vi "SpectrometerSpinCoater_v10.vi"() -> ()   [LabVIEW 2020]
uses:
  <instrlib>/Classes/CCD/Abstract_CCD/Abstract_CCD.lvclass
  TypDef/DeviceQueue_Action.ctl
  TypDef/DeviceQueue_TypeDef.ctl
  TypDef/DataQueue_Action.ctl
  TypDef/DataQueue_TypeDef.ctl
  <instrlib>/Classes/CCD/Avantes/Avantes.lvclass
  <vilib>/Utility/error.llb/DialogType.ctl
  <vilib>/Analysis/NI_AALBase.lvlib
  <vilib>/Analysis/baseanly.llb/A x Vector.vi
  <instrlib>/Classes/SpinCoater/SpinCoater.lvclass
  TypDef/TabControl.ctl
  C:/Program Files/National Instruments/LabVIEW 2020/instr.lib/Classes/CCD/Abstract_CCD/Abstract_CCD.lvclass
  C:/Program Files/National Instruments/LabVIEW 2020/instr.lib/Classes/CCD/Avantes/Avantes.lvclass
panel:
  out "Nr After Spin":u16
  out "Action":string="TimeOut"
  out "Time.spin":refnum<file>
  out "Meas.spin":refnum<file>
  out "Arduino":bool
  out "NKT":bool
  out "Spectromter":bool
  in  "Abort Button":bool
  in  "Stop Button":bool=TRUE
  in  "Tab Control":T1(tab)
  in  "Shutter Toggle":bool
  in  "Spin at end":bool
  in  "Duration after":dbl[unit]
  in  "periodic time":dbl[unit]=2.0
  in  "Program Spin Coater":T2(array[cluster])=[{"Speed (rpm)"=1500.0, "Time (s)"=5.0, "Acc (rpm/s)"=0.0}]
  in  "Spectra Count":u16
  in  "Measure_MeasureSpectrum":bool
  out "Overall Time":dbl=13.0
  in  "Seconds after Spin":dbl[unit]=3.0
  in  "Seconds to Spin":dbl[unit]=5.0
  in  "Calculate Frames":bool=TRUE
  in  "Frames":i32=34211
  in  "StartMeasurement_Button":bool
  in  "Measure_Preview":bool
  out "Measure_Graph":T3(graph) caption="XY Graph"
  in  "Measure_FramesSpectrometer":dbl=200.0 caption="Frames for Spectrometer"
  in  "StartSpin_Button":bool
  in  "Record RefSpec":bool
  in  "Measure:\nRecord_Darkspec":bool
  in  "Measure_Comments":string="Just for testing" caption="Comments"
  in  "Measure_FileName":string="TestingAfter" caption="File Name"
  in  "Measure_SavePath":path=path "C:/Users/Timo/Desktop/testz" caption="Save Path"
  out "Measure_FrameRate":dbl[unit]=2631.5791015625 caption="Frame Rate"
  in  "Measure_IntegrationTime":dbl[unit]=3e-05 caption="Integration Time"
  out "SS_StepsLeft":dbl
  out "SS_TimePrediction":dbl[unit]=-6.0
  out "Horizontal Progress Bar":u8(slide) scale=0.0..100.0
  in  "SpectralStability:\nRecord_Darkspec":bool
  in  "SpectralStability_Record":bool
  in  "SpectralStability_\nMeasurementNumber":u32 caption="Measurement Number"
  in  "SpectralStability_Duration":dbl[unit] caption="Duration"
  in  "Duration/Times":bool
  in  "SpectralStability_\nPeriodicTime":dbl[unit] caption="Periodic Time"
  in  "SpectralStability_MeasureSpectrum":bool
  in  "SpectralStability_Preview":bool
  out "SpectralStability_Graph":T3(graph) caption="XY Graph"
  in  "SpectralStability_FramesSpectrometer":dbl=200.0 caption="Frames for Spectrometer"
  in  "SpectralStability_Comments":string="Just for testing" caption="Comments"
  in  "SpectralStability_FileName":string="TestingAfter" caption="File Name"
  in  "SpectralStability_SavePath":path=path "C:/Users/Timo/Desktop/Test/180824" caption="Save Path"
  out "SpectralStability_FrameRate":dbl[unit]=2631.5791015625 caption="Frame Rate"
  in  "SpectralStability_IntegrationTime":dbl[unit]=3e-05 caption="Integration Time"
  in  "Shutter Close":bool
  in  "Shutter Open":bool
  in  "SHUTTER DEBUG":bool
  in  "Shutter Position":u16=1000
  in  "Dividider Get Spectra":u32=1 min=1
  in  "Automatically \nadjust count":bool=TRUE
  in  "Reset Count\nafter Spin Coating":bool=TRUE
  in  "ESC_Speed":dbl
  in  "ESC_Milliseconds":dbl
  in  "ESC DEBUG":bool
  in  "Port Arduino":refnum<visa-resource-name>="COM4"
  out "Error Arduino":bool caption="Error"
  in  "Init_Arduino":bool caption="Init"
  out "Caption_Settings_Arduino":string="Arduino"
  out "Caption_Settings_NKT":string="NKT Laser"
  out "Error_Spectromter":bool caption="Error"
  in  "Init_Spectrometer":bool caption="Init"
  out "Caption_Settings_Spectrometer":string="Spectromter"
  # "Speed (rpm)   Time (s)        Acceleration \n                                               (rpm/s)"
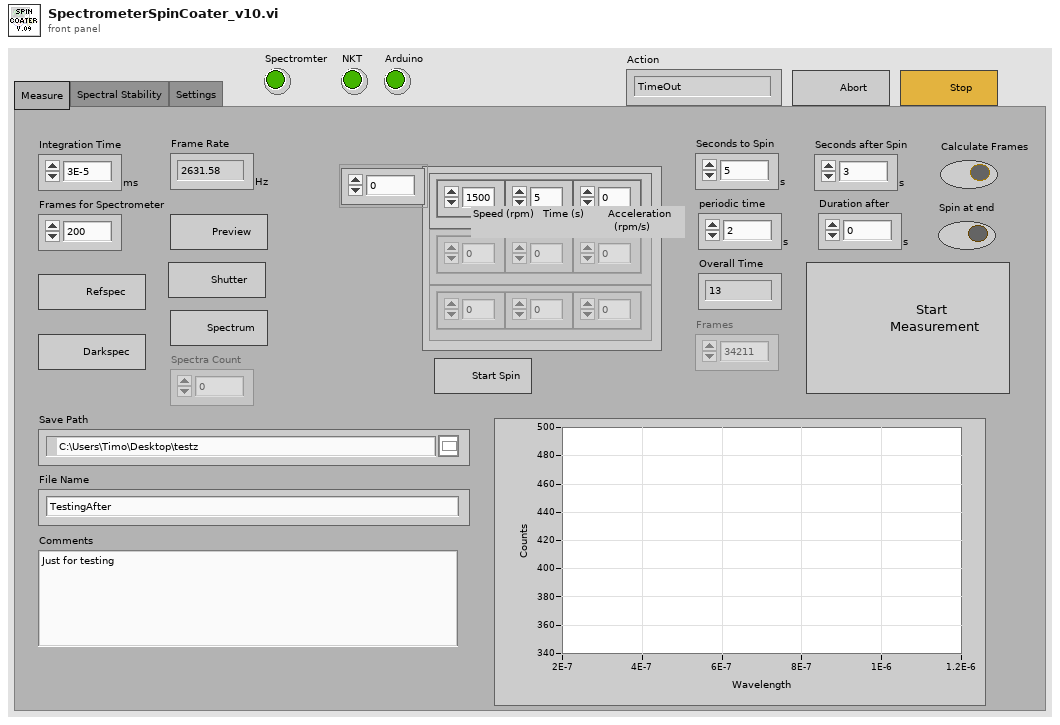
[diagram p1: front panel]
types:
  T1 = enum32{"Measure", "Spectral Stability", "Settings"}
  T2 = cluster{"Speed (rpm)":dbl, "Time (s)":dbl, "Acc (rpm/s)":dbl}[]
  T3 = cluster{"Wavlength":dbl[unit][], "Image":dbl[]}[]
  T4 = cluster{"Dark":cluster{"Image":dbl[][][], "Frame Size":cluster{"F":i32, "Y":i32, "X":i32}}[], "Ref":cluster{"Image":dbl[][][], "Frame Size":cluster{"F":i32, "Y":i32, "X":i32}}[], "Wavlength":dbl[unit][], "spec":dbl[][]}
  T5 = cluster{"Abstract_CCD.lvclass":refnum<class "Abstract_CCD.lvclass">, "SpinCoater.lvclass":refnum<class "SpinCoater.lvclass">}
  T6 = typedef "DataQueue_TypeDef.ctl" = cluster{"QueueAction":T7, "Data":cluster{"Image":dbl[][][], "Frame Size":cluster{"F":i32, "Y":i32, "X":i32}}[], "Data_Raw":cluster{"Image":dbl[][][], "Frame Size":cluster{"F":i32, "Y":i32, "X":i32}}[], "Data_Dark":cluster{"Image":dbl[][][], "Frame Size":cluster{"F":i32, "Y":i32, "X":i32}}[], "Data_Ref":cluster{"Image":dbl[][][], "Frame Size":cluster{"F":i32, "Y":i32, "X":i32}}[], "Device Information":string[], "Numeric Control":dbl, "Boolean":bool, "Wavelength":dbl[unit][], "Time":dbl[], "Time Stamp":timestamp, "Numeric Control 2":dbl, "TabControl":T8}
  T7 = typedef "DataQueue_Action.ctl" = enum16{"TimeOut", "Close_Program", "Abort", "Stop_Measurement", "Measure_InSituSpinCoating", "Measure_Spectrum", "Measure_SpectrumAdvanced", "Measure_SpectralStability", "Save_InSitu", "Save_SpectralStability", "Set_Ref", "Set_Dark", "Set_Wavelength", "Spectrometer_Measure", "Spectrometer_Preview", "Transfer_Settings"}
  T8 = typedef "TabControl.ctl" = enum16{"Measure", "Spectral Stability", "Settings"}
  T9 = typedef "DeviceQueue_TypeDef.ctl" = cluster{"QueueAction":T10, "Numeric 1":dbl, "Numeric 2":dbl, "Boolean 1":bool, "Boolean 2":bool, "Spin Program":dbl[][], "Spin Prg v07":cluster{"Speed (rpm)":dbl, "Time (s)":dbl, "Acc (rpm/s)":dbl}[], "Time Stamp":timestamp, "TabControl":T8}
  T10 = typedef "DeviceQueue_Action.ctl" = enum16{"TimeOut", "Wait", "Close_Program", "Abort", "Spectrometer_Init", "Spectrometer_Close", "Spectrometer_DeviceInformation", "Spectrometer_Measure", "Spectrometer_MeasureAdvanced", "Spectrometer_Preview", "Spectrometer_Abort", "Spectrometer_StartMeasurement", "Spectrometer_GetData", "Spectrometer_StopMeasurement", "Spectrometer_SetIntegrationTime", "Spectrometer_SetFrames", "Spectrometer_SetDarkspec", "Spectrometer_SetReference", "Spectrometer_SetTriggerMode", "Laser_Init", "Laser_Close", "Arduino_Init", "Arduino_Close", "Arduino_LoadProgram", "Arduino_StartProgram", "Arduino_SetSpeed", "Arduino_SetMillis", "Arduino_StopSpin", "Arduino_Shutter_SetPosition", "Arduino_Shutter_Close", "Arduino_Shutter_Open", "Measure_InSitu", "Measure_Spectrum", "Measure_InSituAdvanced", "Measure_SpectralStability", "Measure_Stop"}
  T11 = cluster{"Image":dbl[][][], "Frame Size":cluster{"F":i32, "Y":i32, "X":i32}}[]
  T12 = typedef "DialogType.ctl" = u16
  T13 = enum16{"open", "replace", "create", "open or create", "replace or create", "replace or create with confirmation"}
  T14 = cluster{"Image":dbl[][][], "Frame Size":cluster{"F":i32, "Y":i32, "X":i32}}
  T15 = cluster{"Wavlength":dbl[unit][], "A x Vector":dbl[]}
  T16 = cluster{"Wavlength":dbl[unit][], "A x Vector":dbl[]}[]
  T17 = cluster{u16[][][], u16[][][], dbl[], "Numeric Control":dbl, "Numeric Control 2":dbl}
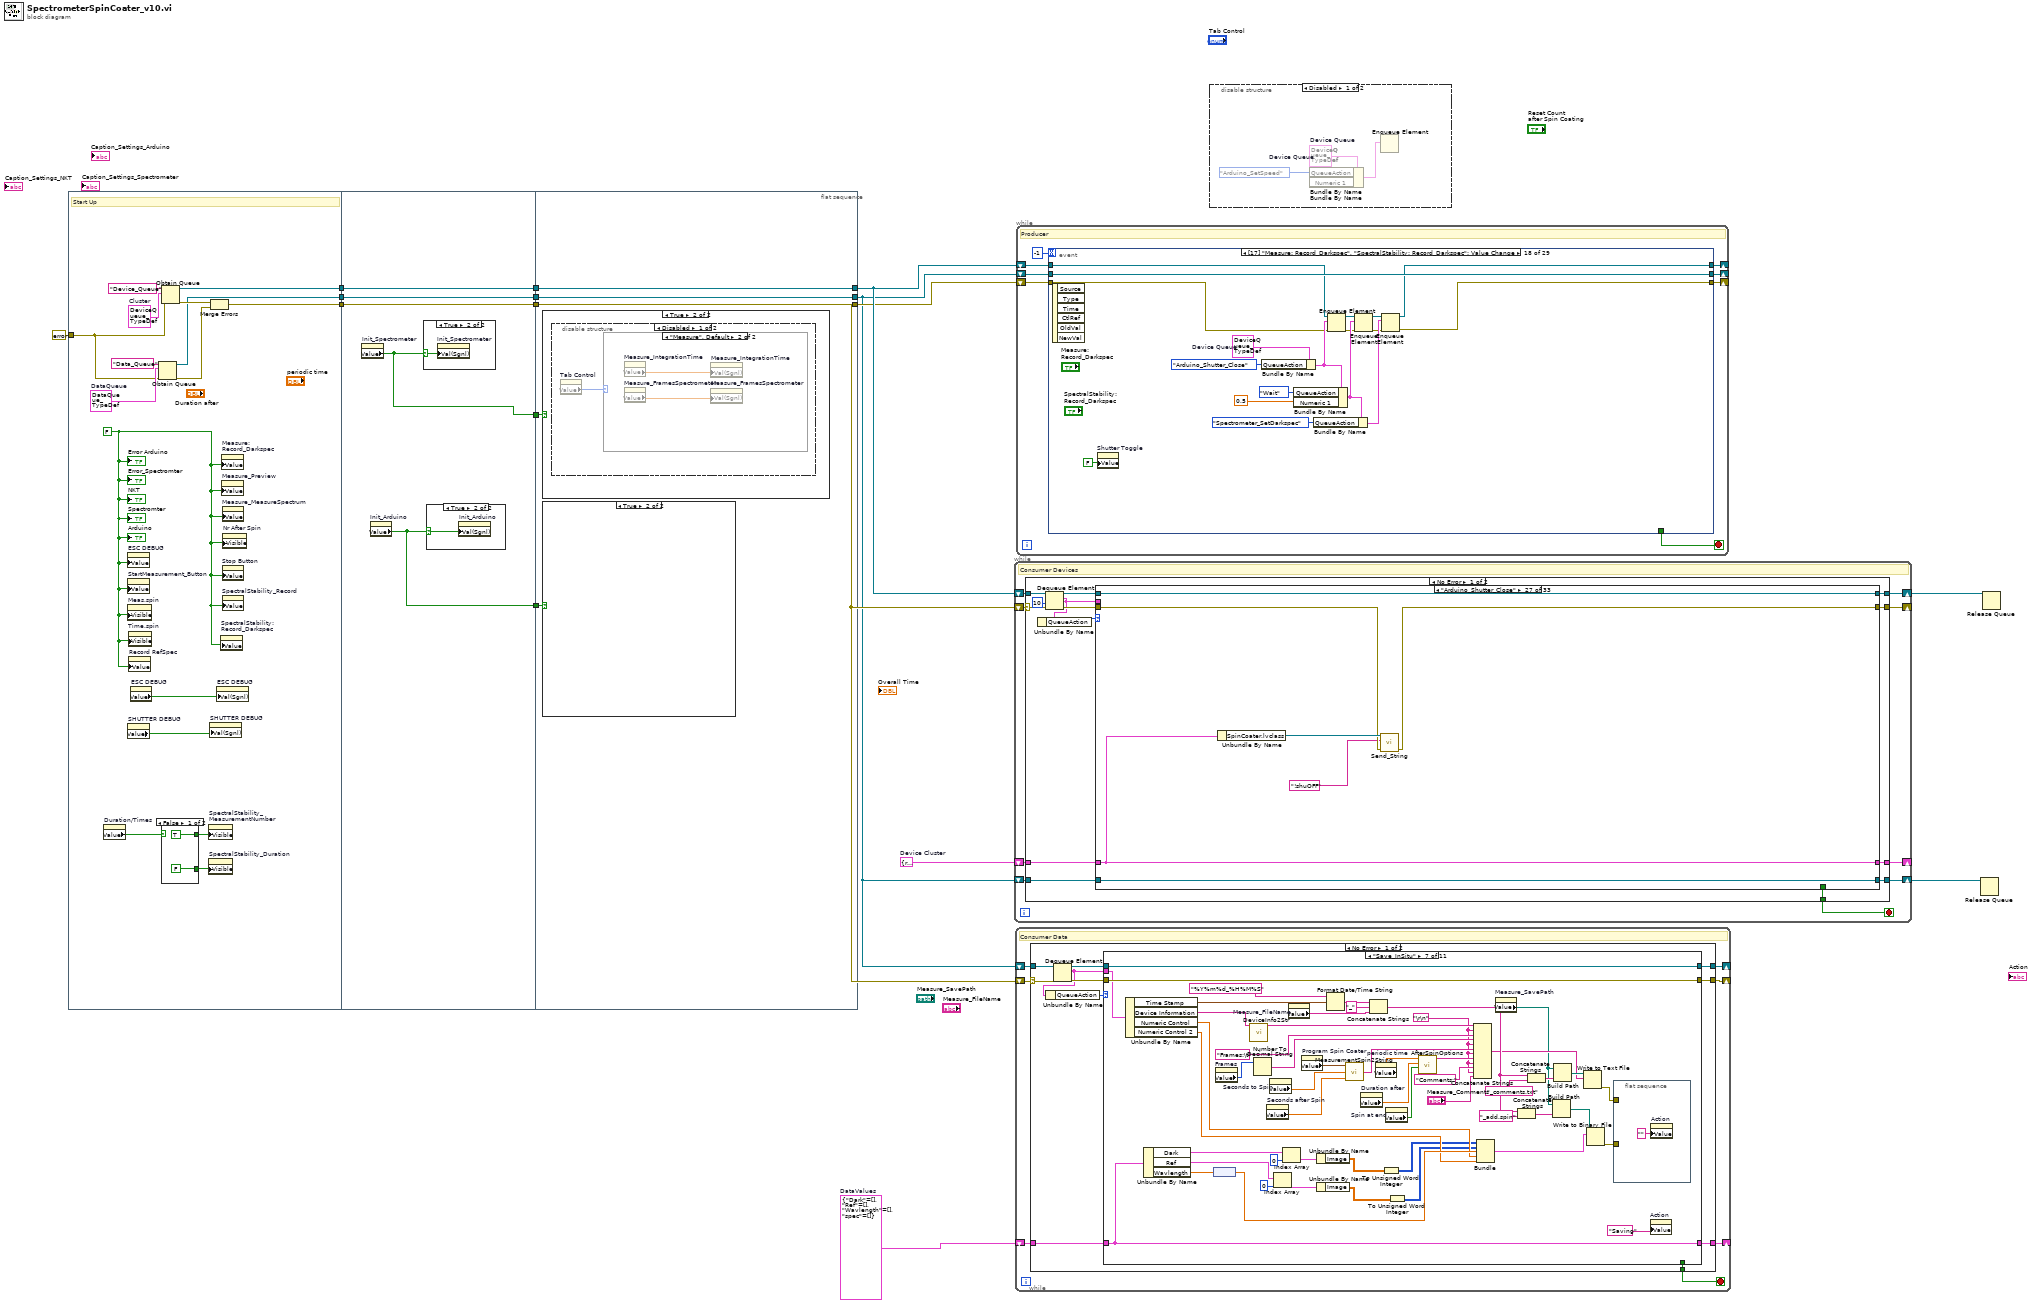
[diagram p0: block diagram]
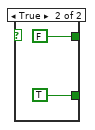
[diagram p3: hidden frame]
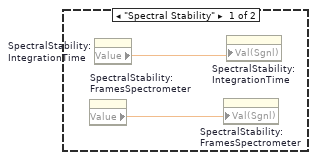
[diagram p8: hidden frame]
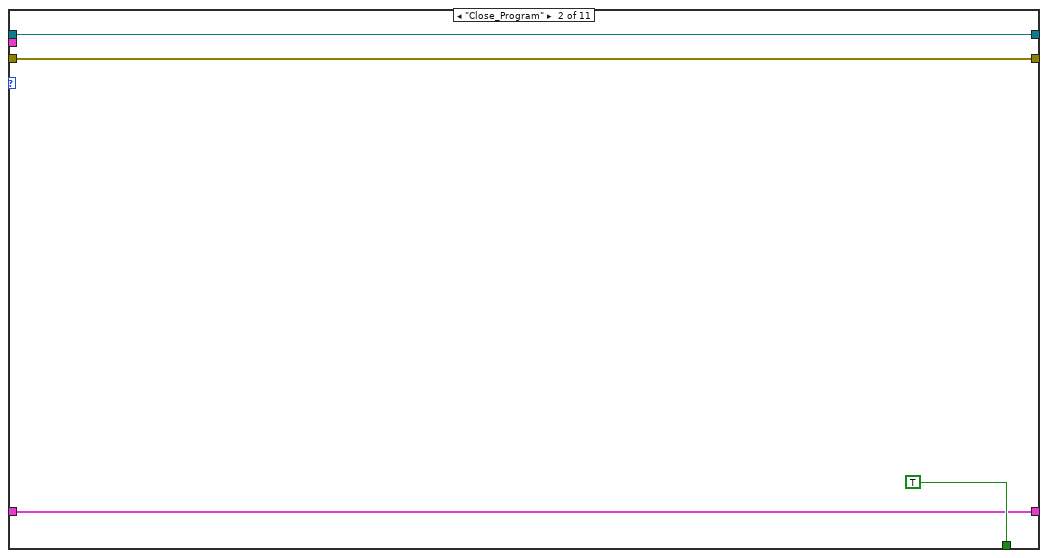
[diagram p11: hidden frame]
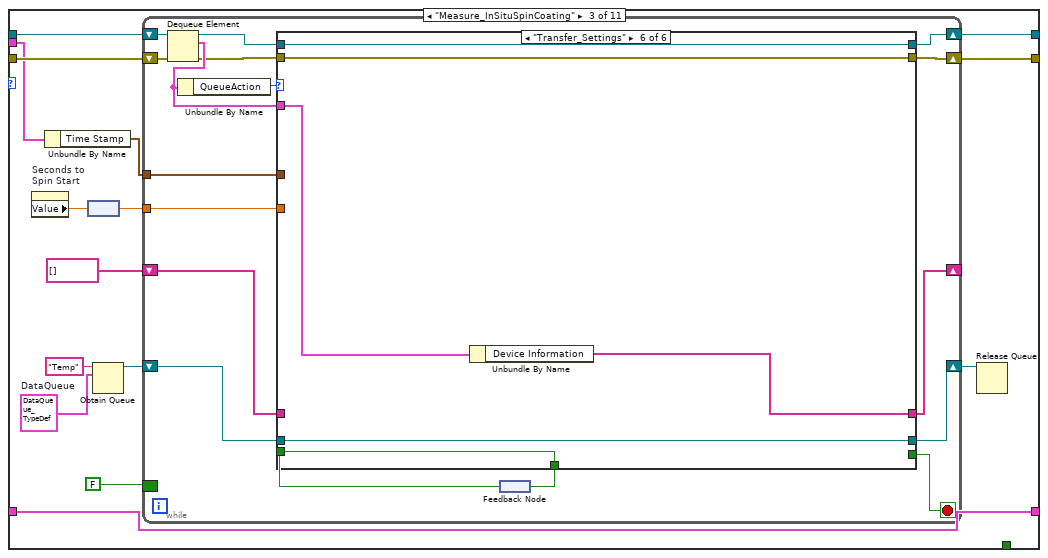
[diagram p12: hidden frame]
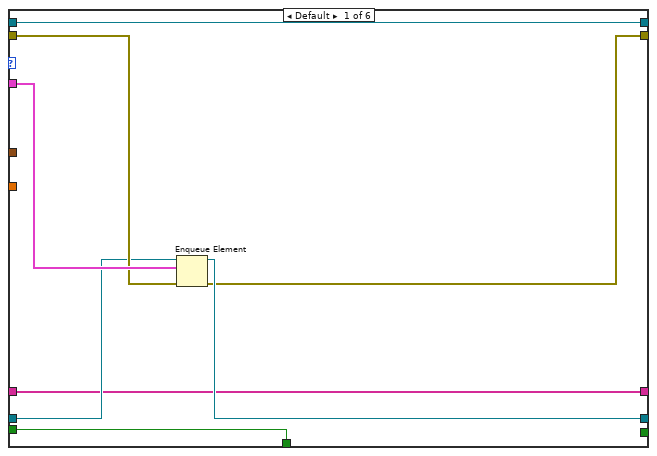
[diagram p13: hidden frame]
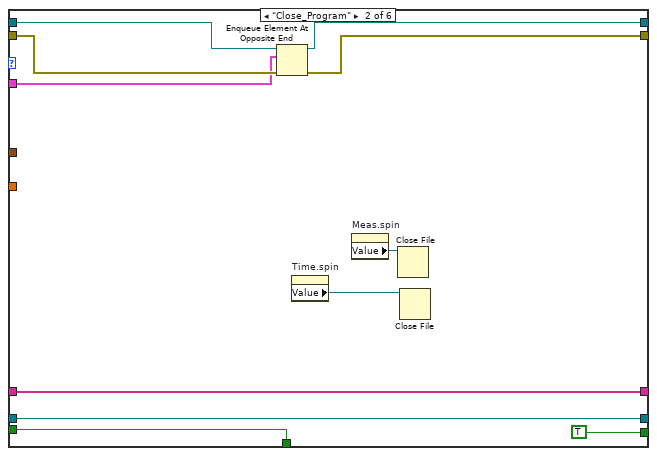
[diagram p14: hidden frame]
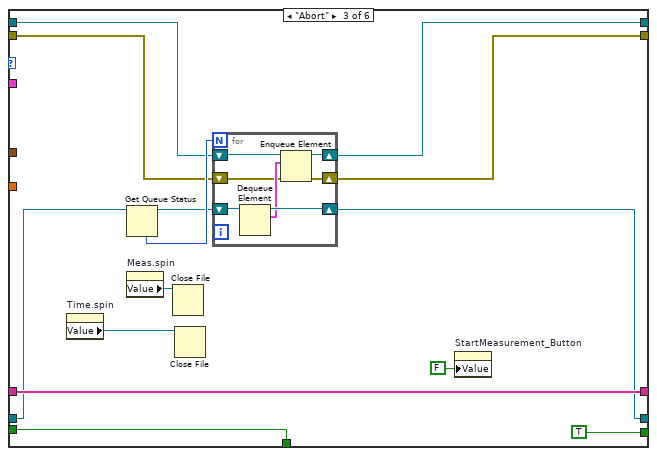
[diagram p15: hidden frame]
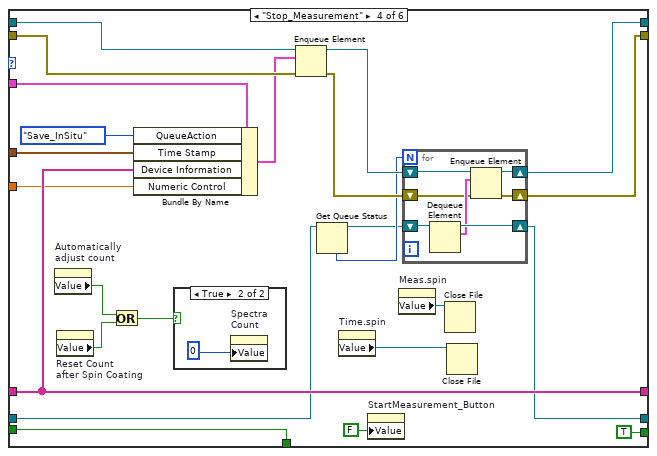
[diagram p16: hidden frame]
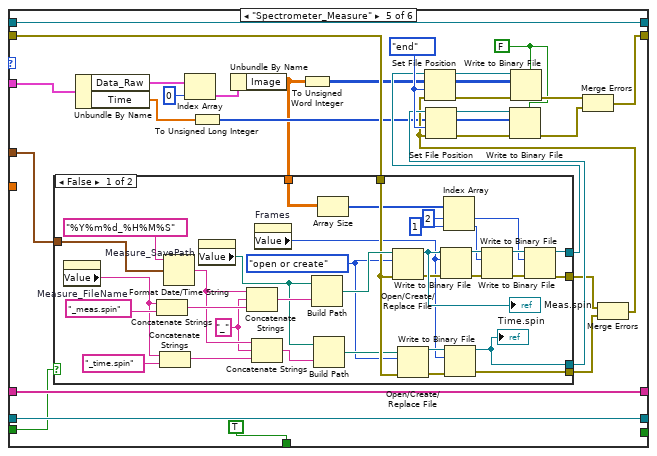
[diagram p18: hidden frame]
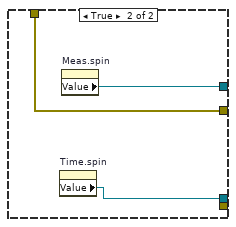
[diagram p19: hidden frame]
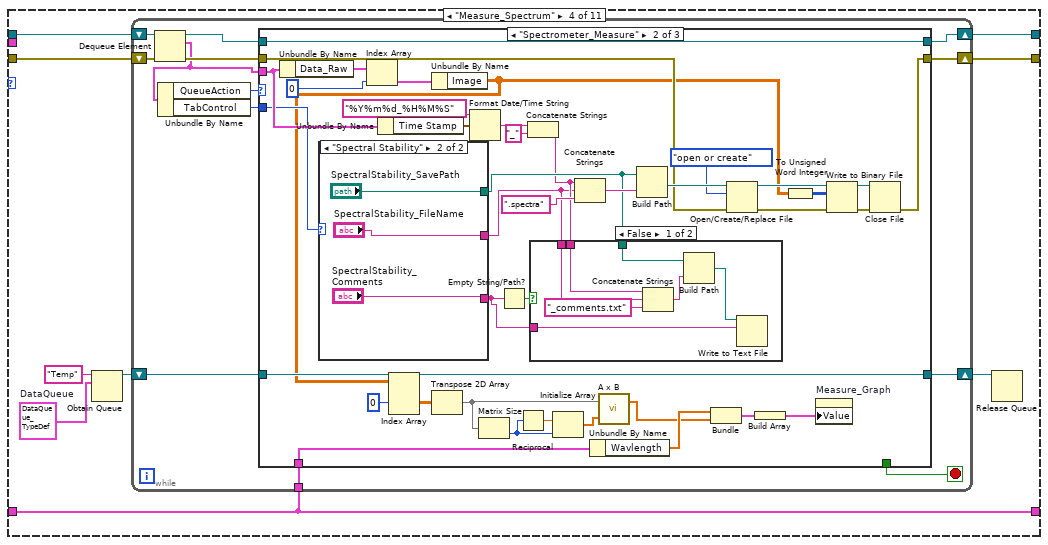
[diagram p20: hidden frame]
diagram:
  w6 = T4 {"Dark"=[], "Ref"=[], "Wavlength"=[], "spec"=[]}  # DataValues
  w11 = T5 {"Abstract_CCD.lvclass"=refnum, "SpinCoater.lvclass"=refnum}  # Device Cluster
  n1 = flat-sequence {
    tunnel: errorcluster {"status"=FALSE, "code"=0, "source"=""} ("error constant") -> [w27]
    tunnel: [w30] -> w15
    tunnel: [w24] -> w14
    tunnel: [w23] -> w13
    tunnel: w15 -> [w41]
    tunnel: w14 -> [w40]
    tunnel: w13 -> [w39]
    tunnel: [w41] -> w5
    tunnel: [w40] -> w4
    tunnel: [w39] -> w3
    tunnel: [w38] -> w2
    tunnel: [w37] -> w1
    tunnel: [w46] -> w8
    tunnel: [w47] -> w7
    tunnel: [w48] -> w12
    tunnel: w5 -> [w48]
    tunnel: w4 -> [w47]
    tunnel: w3 -> [w46]
    tunnel: w2 -> [w45]
    tunnel: w1 -> [w44]
    frame #0 {
      w28 = T6 {"QueueAction"=enum."TimeOut", "Data"=[], "Data_Raw"=[], "Data_Dark"=[], "Data_Ref"=[], "Device Information"=[], "Numeric Control"=0.0, "Boolean"=FALSE, "Wavelength"=[], "Time"=[], "Time Stamp"=timestamp(0 s since 1904-01-01), "Numeric Control 2"=0.0, "TabControl"=enum."Measure"}  # DataQueue
      w31 = T9 {"QueueAction"=enum."TimeOut", "Numeric 1"=0.0, "Numeric 2"=0.0, "Boolean 1"=FALSE, "Boolean 2"=FALSE, "Spin Program"=[], "Spin Prg v07"=[], "Time Stamp"=timestamp(0 s since 1904-01-01), "TabControl"=enum."Measure"}  # Cluster
      w18 = FALSE ("Error Arduino")
      # "Start Up"
      n2 = property on="Duration/Times" class="Bool (strict)"() -> ("Value"=w19:bool)  [unwired: 2 in, 2 out]
      n3 = property on="ESC DEBUG" class="Bool (strict)"("Value"=w18) -> ()  [unwired: 2 in, 2 out]
      n4 = property on="StartMeasurement_Button" class="Bool (strict)"("Value"=w18) -> ()  [unwired: 2 in, 2 out]
      n5 = property on="Meas.spin" class="Ref (strict)"("Visible"=w18) -> ()  [unwired: 2 in, 2 out]
      n6 = property on="SHUTTER DEBUG" class="Bool (strict)"() -> ("Value"=w17:bool)  [unwired: 2 in, 2 out]
      n7 = property on="Time.spin" class="Ref (strict)"("Visible"=w18) -> ()  [unwired: 2 in, 2 out]
      n8 = property on="Record RefSpec" class="Bool (strict)"("Value"=w18) -> ()  [unwired: 2 in, 2 out]
      n9 = property on="ESC DEBUG" class="Bool (strict)"() -> ("Value"=w22:bool)  [unwired: 2 in, 2 out]
      n10 = Obtain Queue(name (unnamed)="Data_Queue", element data type=w28, error in (no error)=w27) -> (queue out=w24:refnum<queue>, error out=w25:errorcluster)  [unwired: 2 in, 1 out]
      n11 = case shown="False" w19 {
        tunnel: [FALSE TRUE] -> w21
        tunnel: [TRUE FALSE] -> w20
        frame False {
        }
        frame True {
        }
      }
      n12 = Obtain Queue(name (unnamed)="Device_Queue", element data type=w31, error in (no error)=w27) -> (queue out=w30:refnum<queue>, error out=w26:errorcluster)  [unwired: 2 in, 1 out]
      n13 = property on="SpectralStability_\nMeasurementNumber" class="DigNum (strict)"("Visible"=w20) -> ()  [unwired: 2 in, 2 out]
      n14 = property on="SpectralStability_Duration" class="DigNum (strict)"("Visible"=w21) -> ()  [unwired: 2 in, 2 out]
      n15 = property on="SHUTTER DEBUG" class="Bool (strict)"("Val(Sgnl)"=w17) -> ()  [unwired: 2 in, 2 out]
      n16 = Merge Errors(w26, w25) -> (w23:errorcluster)
      n17 = property on="ESC DEBUG" class="Bool (strict)"("Val(Sgnl)"=w22) -> ()  [unwired: 2 in, 2 out]
      n18 = property on="SpectralStability:\nRecord_Darkspec" class="Bool (strict)"("Value"=w18) -> ()  [unwired: 2 in, 2 out]
      n19 = property on="Measure:\nRecord_Darkspec" class="Bool (strict)"("Value"=w18) -> ()  [unwired: 2 in, 2 out]
      n20 = property on="Measure_Preview" class="Bool (strict)"("Value"=w18) -> ()  [unwired: 2 in, 2 out]
      n21 = property on="Measure_MeasureSpectrum" class="Bool (strict)"("Value"=w18) -> ()  [unwired: 2 in, 2 out]
      n22 = property on="Stop Button" class="Bool (strict)"("Value"=w18) -> ()  [unwired: 2 in, 2 out]
      n23 = property on="SpectralStability_Record" class="Bool (strict)"("Value"=w18) -> ()  [unwired: 2 in, 2 out]
      n24 = property on="Nr After Spin" class="DigNum (strict)"("Visible"=w18) -> ()  [unwired: 2 in, 2 out]
      "Error_Spectromter" <- w18
      "Error Arduino" <- w18
      "Spectromter" <- w18
      "NKT" <- w18
      "Arduino" <- w18
    }
    frame #1 {
      n25 = property on="Init_Spectrometer" class="Bool (strict)"() -> ("Value"=w38:bool)  [unwired: 2 in, 2 out]
      n26 = property on="Init_Arduino" class="Bool (strict)"() -> ("Value"=w37:bool)  [unwired: 2 in, 2 out]
      n27 = case shown="True" w38 {
        selector: w38 -> [_ w43]
        frame False {
        }
        frame True {
          n28 = property on="Init_Spectrometer" class="Bool (strict)"("Val(Sgnl)"=w43) -> ()  [unwired: 2 in, 2 out]
        }
      }
      n29 = case shown="True" w37 {
        selector: w37 -> [_ w42]
        frame False {
        }
        frame True {
          n30 = property on="Init_Arduino" class="Bool (strict)"("Val(Sgnl)"=w42) -> ()  [unwired: 2 in, 2 out]
        }
      }
    }
    frame #2 {
      n31 = case shown="True" w45 {
        frame False {
        }
        frame True {
          n32 = disable-structure shown="Disabled" {
            frame Disabled {
              n33 = property on="Tab Control" class="TabCtl (strict)"() -> ("Value"=w49:T1)  [unwired: 2 in, 2 out]
              n34 = case shown="\"Measure\", Default" w49 {
                frame "Spectral Stability" {
                  n35 = property on="SpectralStability:\nFramesSpectrometer" class="DigNum (strict)"() -> ("Value"=w50:dbl)  [unwired: 2 in, 2 out]
                  n36 = property on="SpectralStability:\nIntegrationTime" class="DigNum (strict)"() -> ("Value"=w51:dbl[unit])  [unwired: 2 in, 2 out]
                  n37 = property on="SpectralStability:\nFramesSpectrometer" class="DigNum (strict)"("Val(Sgnl)"=w50) -> ()  [unwired: 2 in, 2 out]
                  n38 = property on="SpectralStability:\nIntegrationTime" class="DigNum (strict)"("Val(Sgnl)"=w51) -> ()  [unwired: 2 in, 2 out]
                }
                frame "Measure", Default {
                  n39 = property on="Measure_IntegrationTime" class="DigNum (strict)"() -> ("Value"=w52:dbl[unit])  [unwired: 2 in, 2 out]
                  n40 = property on="Measure_FramesSpectrometer" class="DigNum (strict)"() -> ("Value"=w53:dbl)  [unwired: 2 in, 2 out]
                  n41 = property on="Measure_IntegrationTime" class="DigNum (strict)"("Val(Sgnl)"=w52) -> ()  [unwired: 2 in, 2 out]
                  n42 = property on="Measure_FramesSpectrometer" class="DigNum (strict)"("Val(Sgnl)"=w53) -> ()  [unwired: 2 in, 2 out]
                }
              }
            }
            frame Enabled {
            }
          }
        }
      }
      n43 = case shown="True" w44 {
        frame False {
        }
        frame True {
        }
      }
    }
  }
  n44 = while {
    shift-right: [w58] -> _
    shift-left: w8 -> [w62]
    shift-right: [w59] -> w10
    shift-left: w12 -> [w61]
    shift-right: [w56] -> w9
    shift-left: w7 -> [w57]
    shift-right: [w54] -> _
    shift-left: w11 -> [w55]
    stop <- w60 stop-if-true
    # "Consumer Devices"
    n45 = case shown="No Error" w62 {
      selector: w62 -> [w75 w792]
      tunnel: w61 -> [w76 w793]
      tunnel: [w72 _] -> w60
      tunnel: [w71 w793] -> w59
      tunnel: [w69 w789] -> w58
      tunnel: w57 -> [w67 w787]
      tunnel: [w68 w787] -> w56
      tunnel: w55 -> [w66 w788]
      tunnel: [w65 w788] -> w54
      frame No Error {
        n46 = Dequeue Element(queue=w76, timeout in ms (-1)=10, error in (no error)=w75) -> (queue out=w74:refnum<queue>, element=w64:T9, error out=w70:errorcluster)  [unwired: 1 out]
        n47 = Unbundle By Name(w64) -> ("QueueAction"=w73:T10)
        n48 = case shown="\"Arduino_Shutter_Close\"" w73 {
          tunnel: w74 -> [w81 w102 w143 w161 w172 w227 w246 w271 w282 w305 w312 w331 w333 w364 w383 w398 w408 w420 w432 w453 w475 w480 w487 w499 w505 w517 w524 w531 w540 w586 w680 w748 w758]
          tunnel: [_ _ w145 _ _ _ _ _ _ _ _ _ _ _ _ _ _ _ _ _ _ _ _ _ _ _ _ _ _ _ _ _ _] -> w72
          tunnel: [w81 w102 w128 w147 w168 w227 w246 w271 w283 w305 w312 w331 w333 w364 w383 w398 w408 w420 w431 w453 w475 w480 w487 w499 w505 w517 w524 w531 w540 w548 w596 w739 w761] -> w71
          tunnel: w70 -> [w80 w101 w127 w160 w183 w228 w245 w270 w278 w308 w316 w328 w343 w362 w373 w389 w405 w416 w427 w456 w469 w477 w485 w494 w502 w508 w520 w527 w533 w542 w641 w747 w757]
          tunnel: [w80 w101 w126 w148 w171 w222 w244 w269 w276 w306 w313 w318 w337 w361 w368 w385 w403 w410 w430 w455 w466 w476 w483 w493 w501 w507 w519 w526 w532 w549 w595 w738 w762] -> w69
          tunnel: [w78 w99 w125 w165 w169 w224 w237 w251 w287 w304 w311 w322 w345 w365 w377 w392 w399 w412 w434 w454 w474 w482 w491 w497 w506 w516 w523 w530 w535 w557 w653 w746 w778] -> w68
          tunnel: w67 -> [w78 w99 w125 w165 w170 w224 w236 w260 w288 w304 w311 w323 w345 w365 w380 w395 w399 w414 w434 w454 w474 w482 w491 w497 w506 w516 w523 w530 w536 w557 w653 w746 w778]
          tunnel: w66 -> [w79 w100 w124 w164 w180 w226 w243 w268 w281 w303 w315 w324 w336 w358 w376 w391 w402 w409 w429 w449 w468 w481 w490 w496 w504 w515 w522 w529 w534 w589 w683 w745 w777]
          tunnel: [w79 w100 w124 w164 w174 w225 w243 w268 w280 w301 w310 w324 w334 w359 w375 w390 w400 w409 w433 w447 w465 w481 w490 w496 w504 w515 w522 w529 w534 w589 w683 w745 w777] -> w65
          tunnel: w64 -> [_ w95 _ _ w167 _ w235 w262 w274 _ _ w330 w340 w366 _ _ w406 _ _ _ w473 _ w489 w498 _ w513 _ _ _ _ w623 w736 w752]
          frame "TimeOut", Default {
            n49 = property on="Action" class="Str"("Value"="TimeOut" ("Action")) -> ()  [unwired: 2 in, 2 out]
          }
          frame "Wait" {
            n50 = flat-sequence {
              tunnel: [w113] -> w96
              tunnel: w95 -> [w113]
              tunnel: [w112] -> w93
              frame #0 {
                n51 = Tick Count (ms)() -> (millisecond timer value=w112:u32)
              }
            }
            n52 = Unbundle By Name(w96) -> ("Numeric 1"=w87:dbl)
            n53 = property on="SS:PeriodicTime" class="DigNum (strict)"() -> ("Value"=w89:dbl[unit])  [unwired: 2 in, 2 out]
            n54 = Multiply(x=w87, y=1000.0) -> (x*y=w91:dbl)
            n55 = node(w87) -> (w88:dbl[unit])
            n56 = property on="SS_StepsLeft" class="DigNum (strict)"() -> ("Value"=w86:dbl)  [unwired: 2 in, 2 out]
            n57 = Round Toward -Infinity(1:w87) -> (0:w90:dbl)
            n58 = Subtract(x=w89, y=w88) -> (x-y=w83:dbl[unit])
            n59 = Decrement(x=w86) -> (x-1=w85:dbl)
            n60 = Multiply(x=w85, y=w89) -> (x*y=w84:dbl[unit])
            n61 = Add(x=w84, y=w83) -> (x+y=w82:dbl[unit])
            n62 = for {
              N: w90 -> [_]
              tunnel: 1000.0 ("y") -> [w114]
              tunnel: [w122] -> w94
              tunnel: w82 -> [w119]
              i -> [w117]
              stop <- w122 stop-if-true
              n63 = Increment(x=w117) -> (x+1=w115:i32)
              n64 = Multiply(x=w114, y=w115) -> (x*y=w116:dbl)
              n65 = node(w116) -> (w118:dbl[unit])
              n66 = property on="Stop Button" class="Bool (strict)"() -> ("Value"=w122:bool)  [unwired: 2 in, 2 out]
              n67 = Wait (ms)(milliseconds to wait=w114) -> (millisecond timer value=w120:u32)
              n68 = Subtract(x=w119, y=w118) -> (x-y=w121:dbl[unit])
              n69 = flat-sequence {
                tunnel: w121 -> [w123]
                tunnel: w120 -> [_]
                frame #0 {
                  n70 = property on="SS_TimePrediction" class="DigNum (strict)"("Value"=w123) -> ()  [unwired: 2 in, 2 out]
                }
              }
            }
            n71 = property on="Action" class="Str"("Value"="Wait" ("Action")) -> ()  [unwired: 2 in, 2 out]
            n72 = case shown="False" w94 {
              tunnel: w93 -> [w108 _]
              tunnel: w91 -> [w103 _]
              frame False {
                n73 = flat-sequence {
                  tunnel: [w111] -> w109
                  frame #0 {
                    n74 = Tick Count (ms)() -> (millisecond timer value=w111:u32)
                  }
                }
                n75 = Subtract(x=w109, y=w108) -> (x-y=w107:u32)
                n76 = To Double Precision Float(number=w107) -> (double precision float=w104:dbl)
                n77 = Subtract(x=w103, y=w104) -> (x-y=w105:dbl)
                n78 = Greater Than 0?(x=w105) -> (x > 0?=w106:bool)
                n79 = case shown="True" w106 {
                  tunnel: w105 -> [_ w110]
                  frame False {
                  }
                  frame True {
                    n80 = Wait (ms)(milliseconds to wait=w110) -> ()  [unwired: 1 out]
                  }
                }
              }
              frame True {
                # "If Aborted, do nothing"
              }
            }
          }
          frame "Close_Program" {
            w144 = T9 {"QueueAction"=enum."TimeOut", "Numeric 1"=0.0, "Numeric 2"=0.0, "Boolean 1"=FALSE, "Boolean 2"=FALSE, "Spin Program"=[], "Spin Prg v07"=[], "Time Stamp"=timestamp(0 s since 1904-01-01), "TabControl"=enum."Measure"}  # Device Queue
            n81 = Bundle By Name(cluster=w144, "QueueAction"=DeviceQueue_Action."Spectrometer_Close") -> (w139:T9)
            n82 = Bundle By Name(cluster=w139, "QueueAction"=DeviceQueue_Action."Laser_Close") -> (w137:T9)
            n83 = Bundle By Name(cluster=w137, "QueueAction"=DeviceQueue_Action."Arduino_Close") -> (w131:T9)
            n84 = Enqueue Element(queue=w143, element=w139, error in (no error)=w127) -> (queue out=w141:refnum<queue>, error out=w136:errorcluster)  [unwired: 1 in, 1 out]
            n85 = Bundle By Name(cluster=w131, "QueueAction"=DeviceQueue_Action."Close_Program") -> (w129:T9)
            n86 = Enqueue Element(queue=w141, element=w137, error in (no error)=w136) -> (queue out=w135:refnum<queue>, error out=w134:errorcluster)  [unwired: 1 in, 1 out]
            n87 = Enqueue Element(queue=w135, element=w131, error in (no error)=w134) -> (queue out=w133:refnum<queue>, error out=w132:errorcluster)  [unwired: 1 in, 1 out]
            n88 = Enqueue Element(queue=w133, element=w129, error in (no error)=w132) -> (queue out=w128:refnum<queue>, error out=w126:errorcluster)  [unwired: 1 in, 1 out]
            n89 = First Call?() -> (First Call?: T/F=w146:bool)
            n90 = Not(x=w146) -> (.not. x?=w145:bool)
          }
          frame "Abort" {
            w163 = T9 {"QueueAction"=enum."TimeOut", "Numeric 1"=0.0, "Numeric 2"=0.0, "Boolean 1"=FALSE, "Boolean 2"=FALSE, "Spin Program"=[], "Spin Prg v07"=[], "Time Stamp"=timestamp(0 s since 1904-01-01), "TabControl"=enum."Measure"}  # Device Queue
            n91 = Flush Queue(queue=w161, error in (no error)=w160) -> (queue out=w159:refnum<queue>, error out=w158:errorcluster)  [unwired: 1 out]
            n92 = Bundle By Name(cluster=w163, "QueueAction"=DeviceQueue_Action."Spectrometer_StopMeasurement") -> (w155:T9)
            n93 = Bundle By Name(cluster=w155, "QueueAction"=DeviceQueue_Action."Arduino_StopSpin") -> (w151:T9)
            n94 = Enqueue Element(queue=w159, element=w155, error in (no error)=w158) -> (queue out=w157:refnum<queue>, error out=w156:errorcluster)  [unwired: 1 in, 1 out]
            n95 = Bundle By Name(cluster=w151, "QueueAction"=DeviceQueue_Action."Measure_Stop") -> (w150:T9)
            n96 = Enqueue Element(queue=w157, element=w151, error in (no error)=w156) -> (queue out=w153:refnum<queue>, error out=w152:errorcluster)  [unwired: 1 in, 1 out]
            n97 = Enqueue Element(queue=w153, element=w150, error in (no error)=w152) -> (queue out=w147:refnum<queue>, error out=w148:errorcluster)  [unwired: 1 in, 1 out]
          }
          frame "Spectrometer_Init" {
            n98 = call-dynamic "Init.vi"("error in (no error)"=w183, "Variant"=0, "Avantes in"=refnum<class "Avantes.lvclass"> refnum ("Avantes.lvclass")) -> ("error out"=w182:errorcluster, "Avantes out"=w181:refnum<class "Avantes.lvclass">)  [unwired: 7 in]
            n99 = call-dynamic "IsInit.vi"("error in (no error)"=w182, "Avantes in"=w181) -> ("error out"=w178:errorcluster, "Is Init?"=w177:bool, "Avantes out"=w179:refnum<class "Avantes.lvclass">)  [unwired: 7 in]
            n100 = Unbundle By Name(w167) -> ("TabControl"=w166:T8)
            n101 = property on="Spectromter" class="Bool (strict)"("Value"=w177) -> ()  [unwired: 2 in, 2 out]
            n102 = property on="Init_Spectrometer" class="Bool (strict)"("Value"=w177) -> ()  [unwired: 2 in, 2 out]
            n103 = call-dynamic "Set_ExposurePerFrame.vi"("error in (no error)"=w178, "Exposure per Frame"=1, "Avantes in"=w179) -> ("error out"=w173:errorcluster, "Avantes out"=w176:refnum<class "Avantes.lvclass">)  [unwired: 7 in]
            n104 = case shown="False" w177 {
              tunnel: w176 -> [_ w206]
              tunnel: w173 -> [w189 w204]
              tunnel: [refnum<class "Abstract_CCD.lvclass"> refnum ("Abstract_CCD.lvclass") w205] -> w175
              tunnel: w172 -> [w187 w216]
              tunnel: [w189 w209] -> w171
              tunnel: w170 -> [w188 w201]
              tunnel: [w188 w199] -> w169
              tunnel: [w187 w197] -> w168
              tunnel: w167 -> [_ w194]
              tunnel: w166 -> [_ w193]
              frame False {
              }
              frame True {
                w207 = T6 {"QueueAction"=enum."TimeOut", "Data"=[], "Data_Raw"=[], "Data_Dark"=[], "Data_Ref"=[], "Device Information"=[], "Numeric Control"=0.0, "Boolean"=FALSE, "Wavelength"=[], "Time"=[], "Time Stamp"=timestamp(0 s since 1904-01-01), "Numeric Control 2"=0.0, "TabControl"=enum."Measure"}  # DataQueue
                n105 = case shown="\"Spectral Stability\"" w193 {
                  tunnel: [w218 w220] -> w192
                  tunnel: [w217 w219] -> w191
                  frame "Measure", Default {
                    n106 = property on="Measure_IntegrationTime" class="DigNum (strict)"() -> ("Value"=w218:dbl[unit])  [unwired: 2 in, 2 out]
                    n107 = property on="Measure_FramesSpectrometer" class="DigNum (strict)"() -> ("Value"=w217:dbl)  [unwired: 2 in, 2 out]
                  }
                  frame "Spectral Stability" {
                    n108 = property on="SpectralStability_FramesSpectrometer" class="DigNum (strict)"() -> ("Value"=w219:dbl)  [unwired: 2 in, 2 out]
                    n109 = property on="SpectralStability_IntegrationTime" class="DigNum (strict)"() -> ("Value"=w220:dbl[unit])  [unwired: 2 in, 2 out]
                  }
                }
                n110 = call-dynamic "Get_WavelengthAxis.vi"("error in (no error)"=w204, "Avantes in"=w206) -> ("error out"=w203:errorcluster, "lambda"=w198:dbl[unit][], "Avantes out"=w205:refnum<class "Avantes.lvclass">)  [unwired: 7 in]
                n111 = Unbundle(w203) -> ("status"=w202:bool)  [unwired: 2 out]
                n112 = property on="Error_Spectromter" class="Bool (strict)"("Value"=w202) -> ()  [unwired: 2 in, 2 out]
                n113 = property on="Calculate Frames" class="Bool (strict)"() -> ("Value"=w195:bool)  [unwired: 2 in, 2 out]
                n114 = Bundle By Name(cluster=w207, "QueueAction"=DataQueue_Action."Set_Wavelength", "Wavelength"=w198) -> (w208:T6)
                n115 = node(w192) -> (w214:dbl)
                n116 = Bundle By Name(cluster=w194, "QueueAction"=DeviceQueue_Action."Spectrometer_SetIntegrationTime", "Numeric 1"=w214, "Boolean 1"=w195) -> (w212:T9)
                n117 = Enqueue Element(queue=w201, element=w208) -> (queue out=w199:refnum<queue>)  [unwired: 2 in, 2 out]
                n118 = Bundle By Name(cluster=w212, "QueueAction"=DeviceQueue_Action."Spectrometer_SetFrames", "Numeric 1"=w191) -> (w211:T9)
                n119 = Enqueue Element(queue=w216, element=w212, error in (no error)=w204) -> (queue out=w213:refnum<queue>, error out=w210:errorcluster)  [unwired: 1 in, 1 out]
                n120 = Enqueue Element(queue=w213, element=w211, error in (no error)=w210) -> (queue out=w197:refnum<queue>, error out=w209:errorcluster)  [unwired: 1 in, 1 out]
              }
            }
            n121 = Bundle By Name(cluster=w180, "Abstract_CCD.lvclass"=w175) -> (w174:T5)
          }
          frame "Spectrometer_Close" {
            n122 = property on="Spectromter" class="Bool (strict)"("Value"=FALSE ("Spectromter")) -> ()  [unwired: 2 in, 2 out]
            n123 = Unbundle By Name(w226) -> ("Abstract_CCD.lvclass"=w229:refnum<class "Abstract_CCD.lvclass">)
            n124 = flat-sequence {
              tunnel: [refnum<class "Abstract_CCD.lvclass"> refnum ("Abstract_CCD.lvclass")] -> w223
              tunnel: w222 -> [_]
              frame #0 {
              }
            }
            n125 = call-dynamic "Close.vi"("error in (no error)"=w228, "Abstract_CCD in"=w229) -> ("error out"=w222:errorcluster)  [unwired: 8 in, 1 out]
            n126 = Bundle By Name(cluster=w226, "Abstract_CCD.lvclass"=w223) -> (w225:T5)
          }
          frame "Spectrometer_Measure" {
            w248 = T6 {"QueueAction"=enum."TimeOut", "Data"=[], "Data_Raw"=[], "Data_Dark"=[], "Data_Ref"=[], "Device Information"=[], "Numeric Control"=0.0, "Boolean"=FALSE, "Wavelength"=[], "Time"=[], "Time Stamp"=timestamp(0 s since 1904-01-01), "Numeric Control 2"=0.0, "TabControl"=enum."Measure"}  # DataQueue
            n127 = Unbundle By Name(w243) -> ("Abstract_CCD.lvclass"=w247:refnum<class "Abstract_CCD.lvclass">)
            n128 = Unbundle By Name(w235) -> ("Time Stamp"=w232:timestamp, "TabControl"=w233:T8)
            n129 = Get Date/Time In Seconds() -> (seconds since 1Jan1904=w231:timestamp)
            n130 = Subtract(x=w231, y=w232) -> (x-y=w234:dbl)
            n131 = call-dynamic "Measure.vi"("error in (no error)"=w245, "Abstract_CCD in"=w247) -> ("error out"=w244:errorcluster, "Data Raw"=w240:T11, "Data"=w241:T11, "Darkspec"=w239:T11, "Time"=w238:dbl[])  [unwired: 3 in, 2 out]
            n132 = Bundle By Name(cluster=w248, "QueueAction"=DataQueue_Action."Spectrometer_Measure", "Data"=w241, "Data_Raw"=w240, "Data_Dark"=w239, "Time"=w238, "Time Stamp"=w232, "Numeric Control 2"=w234, "TabControl"=w233) -> (w249:T6)
            n133 = Enqueue Element(queue=w236, element=w249) -> (queue out=w237:refnum<queue>)  [unwired: 2 in, 2 out]
          }
          frame "Spectrometer_MeasureAdvanced" {
            w259 = T6 {"QueueAction"=enum."TimeOut", "Data"=[], "Data_Raw"=[], "Data_Dark"=[], "Data_Ref"=[], "Device Information"=[], "Numeric Control"=0.0, "Boolean"=FALSE, "Wavelength"=[], "Time"=[], "Time Stamp"=timestamp(0 s since 1904-01-01), "Numeric Control 2"=0.0, "TabControl"=enum."Measure"}  # DataQueue
            w273 = T6 {"QueueAction"=enum."TimeOut", "Data"=[], "Data_Raw"=[], "Data_Dark"=[], "Data_Ref"=[], "Device Information"=[], "Numeric Control"=0.0, "Boolean"=FALSE, "Wavelength"=[], "Time"=[], "Time Stamp"=timestamp(0 s since 1904-01-01), "Numeric Control 2"=0.0, "TabControl"=enum."Measure"}  # DataQueue
            n134 = Unbundle By Name(w268) -> ("Abstract_CCD.lvclass"=w272:refnum<class "Abstract_CCD.lvclass">)
            n135 = Unbundle By Name(w262) -> ("Time Stamp"=w261:timestamp)
            n136 = call-dynamic "Measure.vi"("error in (no error)"=w270, "Abstract_CCD in"=w272) -> ("error out"=w269:errorcluster, "Data Raw"=w265:T11, "Data"=w266:T11, "Darkspec"=w264:T11, "Time"=w263:dbl[])  [unwired: 3 in, 2 out]
            n137 = Bundle By Name(cluster=w259, "QueueAction"=DataQueue_Action."Measure_SpectrumAdvanced") -> (w257:T6)
            n138 = Bundle By Name(cluster=w273, "QueueAction"=DataQueue_Action."Spectrometer_Measure", "Data"=w266, "Data_Raw"=w265, "Data_Dark"=w264, "Time"=w263, "Time Stamp"=w261) -> (w254:T6)
            n139 = Enqueue Element(queue=w260, element=w257) -> (queue out=w256:refnum<queue>)  [unwired: 2 in, 2 out]
            n140 = Enqueue Element(queue=w256, element=w254) -> (queue out=w255:refnum<queue>)  [unwired: 2 in, 2 out]
            n141 = Bundle By Name(cluster=w254, "QueueAction"=DataQueue_Action."Stop_Measurement") -> (w252:T6)
            n142 = property on="Action" class="Str"("Value"="Measure Spectra A" ("Action")) -> ()  [unwired: 2 in, 2 out]
            n143 = Enqueue Element(queue=w255, element=w252) -> (queue out=w251:refnum<queue>)  [unwired: 2 in, 2 out]
          }
          frame "Spectrometer_Preview" {
            w289 = T6 {"QueueAction"=enum."TimeOut", "Data"=[], "Data_Raw"=[], "Data_Dark"=[], "Data_Ref"=[], "Device Information"=[], "Numeric Control"=0.0, "Boolean"=FALSE, "Wavelength"=[], "Time"=[], "Time Stamp"=timestamp(0 s since 1904-01-01), "Numeric Control 2"=0.0, "TabControl"=enum."Measure"}  # DataQueue
            n144 = Unbundle By Name(w281) -> ("Abstract_CCD.lvclass"=w279:refnum<class "Abstract_CCD.lvclass">)
            n145 = Unbundle By Name(w274) -> ("TabControl"=w275:T8)
            n146 = call-dynamic "Measure.vi"("error in (no error)"=w278, "Abstract_CCD in"=w279) -> ("error out"=w276:errorcluster, "Data Raw"=w286:T11, "Abstract_CCD out"=w277:refnum<class "Abstract_CCD.lvclass">)  [unwired: 3 in, 4 out]
            n147 = case shown="\"Measure\"" w275 {
              tunnel: [FALSE ("Value") w293 w294] -> w284
              tunnel: w276 -> [_ w292 _]
              frame Default {
              }
              frame "Measure" {
                n148 = property on="Measure_Preview" class="Bool (strict)"(error in=w292) -> ("Value"=w293:bool)  [unwired: 1 in, 2 out]
              }
              frame "Spectral Stability" {
                n149 = property on="SpectralStability_Preview" class="Bool (strict)"() -> ("Value"=w294:bool)  [unwired: 2 in, 2 out]
              }
            }
            n150 = case shown="True" w284 {
              tunnel: [w295 w298] -> w283
              tunnel: w282 -> [w295 w297]
              tunnel: w274 -> [_ w296]
              frame False {
              }
              frame True {
                n151 = Bundle By Name(cluster=w296, "QueueAction"=DeviceQueue_Action."Spectrometer_Preview") -> (w299:T9)
                n152 = Enqueue Element(queue=w297, element=w299) -> (queue out=w298:refnum<queue>)  [unwired: 2 in, 2 out]
              }
            }
            n153 = Bundle By Name(cluster=w289, "Data_Raw"=w286, "QueueAction"=DataQueue_Action."Spectrometer_Preview", "TabControl"=w275) -> (w290:T6)
            n154 = Enqueue Element(queue=w288, element=w290) -> (queue out=w287:refnum<queue>)  [unwired: 2 in, 2 out]
            n155 = Bundle By Name(cluster=w281, "Abstract_CCD.lvclass"=w277) -> (w280:T5)
          }
          frame "Spectrometer_StartMeasurement" {
            n156 = Unbundle By Name(w303) -> ("Abstract_CCD.lvclass"=w307:refnum<class "Abstract_CCD.lvclass">)
            n157 = call-dynamic "StartMeasure.vi"("error in (no error)"=w308, "Frames"=-1, "Abstract_CCD in"=w307) -> ("error out"=w306:errorcluster, "Abstract_CCD out"=w302:refnum<class "Abstract_CCD.lvclass">)  [unwired: 7 in]
            n158 = Bundle By Name(cluster=w303, "Abstract_CCD.lvclass"=w302) -> (w301:T5)
          }
          frame "Spectrometer_StopMeasurement" {
            n159 = Unbundle By Name(w315) -> ("Abstract_CCD.lvclass"=w317:refnum<class "Abstract_CCD.lvclass">)
            n160 = call-dynamic "StopMeasurement.vi"("error in (no error)"=w316, "Abstract_CCD in"=w317) -> ("error out"=w313:errorcluster, "Abstract_CCD out"=w314:refnum<class "Abstract_CCD.lvclass">)  [unwired: 8 in]
            n161 = Bundle By Name(cluster=w315, "Abstract_CCD.lvclass"=w314) -> (w310:T5)
          }
          frame "Spectrometer_GetData" {
            w327 = T6 {"QueueAction"=enum."TimeOut", "Data"=[], "Data_Raw"=[], "Data_Dark"=[], "Data_Ref"=[], "Device Information"=[], "Numeric Control"=0.0, "Boolean"=FALSE, "Wavelength"=[], "Time"=[], "Time Stamp"=timestamp(0 s since 1904-01-01), "Numeric Control 2"=0.0, "TabControl"=enum."Measure"}  # DataQueue
            n162 = Unbundle By Name(w324) -> ("Abstract_CCD.lvclass"=w329:refnum<class "Abstract_CCD.lvclass">)
            n163 = Unbundle By Name(w330) -> ("Numeric 1"=w321:dbl)
            n164 = call-dynamic "Measure_GetData.vi"("error in (no error)"=w328, "SpectraCount"=w321, "Abstract_CCD in"=w329) -> ("error out"=w318:errorcluster, "Data_Raw"=w320:T11, "Time"=w319:dbl[])  [unwired: 5 in, 1 out]
            n165 = Bundle By Name(cluster=w327, "QueueAction"=DataQueue_Action."Spectrometer_Measure", "Data_Raw"=w320, "Time"=w319) -> (w326:T6)
            n166 = Enqueue Element(queue=w323, element=w326) -> (queue out=w322:refnum<queue>)  [unwired: 2 in, 2 out]
          }
          frame "Spectrometer_SetIntegrationTime" {
            n167 = Unbundle By Name(w340) -> ("Numeric 1"=w342:dbl)
            n168 = Unbundle By Name(w336) -> ("Abstract_CCD.lvclass"=w344:refnum<class "Abstract_CCD.lvclass">)
            n169 = Unbundle By Name(w340) -> ("TabControl"=w332:T8, "Boolean 1"=w339:bool)
            n170 = node(w342) -> (w341:dbl[unit])
            n171 = call-dynamic "Set_ExposureTime.vi"("error in (no error)"=w343, "Exposure Time"=w341, "Abstract_CCD in"=w344) -> ("error out"=w347:errorcluster, "Abstract_CCD out"=w346:refnum<class "Abstract_CCD.lvclass">)  [unwired: 7 in]
            n172 = call-dynamic "Get_FrameRate.vi"("error in (no error)"=w347, "Abstract_CCD in"=w346) -> ("error out"=w337:errorcluster, "Frame Rate"=w338:dbl[unit], "Abstract_CCD out"=w335:refnum<class "Abstract_CCD.lvclass">)  [unwired: 7 in]
            n173 = Bundle By Name(cluster=w336, "Abstract_CCD.lvclass"=w335) -> (w334:T5)
            n174 = case shown="\"Measure\"" w332 {
              tunnel: w339 -> [_ _ w350]
              tunnel: w338 -> [_ w348 w349]
              frame Default {
              }
              frame "Spectral Stability" {
                "SpectralStability_FrameRate" <- w348
              }
              frame "Measure" {
                n175 = case shown="True" w350 {
                  tunnel: w349 -> [_ w354]
                  frame False {
                  }
                  frame True {
                    n176 = property on="Program Spin Coater" class="Arr (strict)"() -> ("Value"=w351:T2)  [unwired: 2 in, 2 out]
                    n177 = property on="Seconds to Spin" class="DigNum (strict)"() -> ("Value"=w356:dbl[unit])  [unwired: 2 in, 2 out]
                    n178 = property on="Seconds after Spin" class="DigNum (strict)"() -> ("Value"=w355:dbl[unit])  [unwired: 2 in, 2 out]
                    n179 = call "CalculateFrames_v02.vi"("Program Spin Coater"=w351, "Seconds End"=w355, "Seconds Start"=w356, "Frame Rate"=w354) -> ("Time"=w353:dbl, "Frames"=w352:i32)  [unwired: 6 in]
                    n180 = property on="Frames" class="DigNum (strict)"("Value"=w352) -> ()  [unwired: 2 in, 2 out]
                    n181 = property on="Overall Time" class="DigNum (strict)"("Value"=w353) -> ()  [unwired: 2 in, 2 out]
                  }
                }
                "Measure_FrameRate" <- w349
              }
            }
          }
          frame "Spectrometer_SetFrames" {
            n182 = Unbundle By Name(w358) -> ("Abstract_CCD.lvclass"=w363:refnum<class "Abstract_CCD.lvclass">)
            n183 = Unbundle By Name(w366) -> ("Numeric 1"=w360:dbl)
            n184 = call-dynamic "Set_Frames.vi"("error in (no error)"=w362, "Frames"=w360, "Abstract_CCD in"=w363) -> ("error out"=w361:errorcluster, "Abstract_CCD out"=w357:refnum<class "Abstract_CCD.lvclass">)  [unwired: 7 in]
            n185 = Bundle By Name(cluster=w358, "Abstract_CCD.lvclass"=w357) -> (w359:T5)
          }
          frame "Spectrometer_SetDarkspec" {
            w381 = T6 {"QueueAction"=enum."TimeOut", "Data"=[], "Data_Raw"=[], "Data_Dark"=[], "Data_Ref"=[], "Device Information"=[], "Numeric Control"=0.0, "Boolean"=FALSE, "Wavelength"=[], "Time"=[], "Time Stamp"=timestamp(0 s since 1904-01-01), "Numeric Control 2"=0.0, "TabControl"=enum."Measure"}  # DataQueue
            n186 = Unbundle By Name(w376) -> ("Abstract_CCD.lvclass"=w374:refnum<class "Abstract_CCD.lvclass">)
            n187 = call-dynamic "Measure.vi"("error in (no error)"=w373, "Abstract_CCD in"=w374) -> ("error out"=w371:errorcluster, "Data Raw"=w378:T11, "Abstract_CCD out"=w372:refnum<class "Abstract_CCD.lvclass">)  [unwired: 3 in, 4 out]
            n188 = Bundle By Name(cluster=w381, "QueueAction"=DataQueue_Action."Set_Dark", "Data_Dark"=w378) -> (w382:T6)
            n189 = Enqueue Element(queue=w380, element=w382) -> (queue out=w377:refnum<queue>)  [unwired: 2 in, 2 out]
            n190 = Bundle By Name(cluster=w376, "Abstract_CCD.lvclass"=w372) -> (w375:T5)
            n191 = property on="Measure:\nRecord_Darkspec" class="Bool (strict)"(error in=w371, "Value"=FALSE ("Record_Darkspec")) -> (error out=w369:errorcluster)  [unwired: 1 in, 1 out]
            n192 = property on="SpectralStability:\nRecord_Darkspec" class="Bool (strict)"(error in=w369, "Value"=FALSE ("SpectralStability:\nRecord_Darkspec")) -> (error out=w368:errorcluster)  [unwired: 1 in, 1 out]
          }
          frame "Spectrometer_SetReference" {
            w396 = T6 {"QueueAction"=enum."TimeOut", "Data"=[], "Data_Raw"=[], "Data_Dark"=[], "Data_Ref"=[], "Device Information"=[], "Numeric Control"=0.0, "Boolean"=FALSE, "Wavelength"=[], "Time"=[], "Time Stamp"=timestamp(0 s since 1904-01-01), "Numeric Control 2"=0.0, "TabControl"=enum."Measure"}  # DataQueue
            n193 = Unbundle By Name(w391) -> ("Abstract_CCD.lvclass"=w388:refnum<class "Abstract_CCD.lvclass">)
            n194 = call-dynamic "Measure.vi"("error in (no error)"=w389, "Abstract_CCD in"=w388) -> ("error out"=w386:errorcluster, "Data Raw"=w393:T11, "Abstract_CCD out"=w387:refnum<class "Abstract_CCD.lvclass">)  [unwired: 3 in, 4 out]
            n195 = Bundle By Name(cluster=w396, "QueueAction"=DataQueue_Action."Set_Ref", "Data_Ref"=w393) -> (w397:T6)
            n196 = Enqueue Element(queue=w395, element=w397) -> (queue out=w392:refnum<queue>)  [unwired: 2 in, 2 out]
            n197 = Bundle By Name(cluster=w391, "Abstract_CCD.lvclass"=w387) -> (w390:T5)
            n198 = property on="Record RefSpec" class="Bool (strict)"(error in=w386, "Value"=FALSE ("Record RefSpec")) -> (error out=w385:errorcluster)  [unwired: 1 in, 1 out]
          }
          frame "Spectrometer_SetTriggerMode" {
            n199 = Unbundle By Name(w402) -> ("Abstract_CCD.lvclass"=w407:refnum<class "Abstract_CCD.lvclass">)
            n200 = Unbundle By Name(w406) -> ("Numeric 1"=w404:dbl)
            n201 = call-dynamic "Set_TriggerMode.vi"("error in (no error)"=w405, "Trigger Mode"=w404, "Abstract_CCD in"=w407) -> ("error out"=w403:errorcluster, "Abstract_CCD out"=w401:refnum<class "Abstract_CCD.lvclass">)  [unwired: 7 in]
            n202 = Bundle By Name(cluster=w402, "Abstract_CCD.lvclass"=w401) -> (w400:T5)
          }
          frame "Spectrometer_DeviceInformation" {
            w415 = T6 {"QueueAction"=enum."TimeOut", "Data"=[], "Data_Raw"=[], "Data_Dark"=[], "Data_Ref"=[], "Device Information"=[], "Numeric Control"=0.0, "Boolean"=FALSE, "Wavelength"=[], "Time"=[], "Time Stamp"=timestamp(0 s since 1904-01-01), "Numeric Control 2"=0.0, "TabControl"=enum."Measure"}  # DataQueue
            n203 = Unbundle By Name(w409) -> ("Abstract_CCD.lvclass"=w417:refnum<class "Abstract_CCD.lvclass">)
            n204 = call-dynamic "Get_DeviceInformation.vi"("error in (no error)"=w416, "Abstract_CCD in"=w417) -> ("error out"=w411:errorcluster, "Array"=w418:string[])  [unwired: 7 in, 1 out]
            n205 = Bundle By Name(cluster=w415, "QueueAction"=DataQueue_Action."Transfer_Settings", "Device Information"=w418) -> (w413:T6)
            n206 = Enqueue Element(queue=w414, element=w413, error in (no error)=w411) -> (queue out=w412:refnum<queue>, error out=w410:errorcluster)  [unwired: 1 in, 1 out]
          }
          frame "Arduino_Init" {
            n207 = Unbundle By Name(w429) -> ("SpinCoater.lvclass"=w428:refnum<class "SpinCoater.lvclass">)
            n208 = call-dynamic "Init.vi"("error in (no error)"=w427, "Variant"="Port Arduino", "SpinCoater in"=w428) -> ("error out"=w424:errorcluster, "SpinCoater out"=w425:refnum<class "SpinCoater.lvclass">)  [unwired: 7 in]
            n209 = call-dynamic "IsInit.vi"("error in (no error)"=w424, "SpinCoater in"=w425) -> ("error out"=w421:errorcluster, "Init"=w422:bool, "SpinCoater out"=w423:refnum<class "SpinCoater.lvclass">)  [unwired: 7 in]
            n210 = property on="Arduino" class="Bool (strict)"("Value"=w422) -> ()  [unwired: 2 in, 2 out]
            n211 = case shown="True" w422 {
              tunnel: w432 -> [w436 w445]
              tunnel: [w436 w439] -> w431
              tunnel: [w435 w438] -> w430
              tunnel: w421 -> [w435 w442]
              frame False {
              }
              frame True {
                w446 = T9 {"QueueAction"=enum."TimeOut", "Numeric 1"=0.0, "Numeric 2"=0.0, "Boolean 1"=FALSE, "Boolean 2"=FALSE, "Spin Program"=[], "Spin Prg v07"=[], "Time Stamp"=timestamp(0 s since 1904-01-01), "TabControl"=enum."Measure"}  # Device Queue
                n212 = property on="Program Spin Coater" class="Arr (strict)"() -> ("Value"=w437:T2)  [unwired: 2 in, 2 out]
                n213 = property on="Seconds to Spin" class="DigNum (strict)"() -> ("Value"=w441:dbl[unit])  [unwired: 2 in, 2 out]
                n214 = node(w441) -> (w440:dbl)
                n215 = Bundle By Name(cluster=w446, "QueueAction"=DeviceQueue_Action."Arduino_LoadProgram", "Spin Prg v07"=w437, "Numeric 1"=w440) -> (w444:T9)
                n216 = Enqueue Element(queue=w445, element=w444, error in (no error)=w442) -> (queue out=w439:refnum<queue>, error out=w438:errorcluster)  [unwired: 1 in, 1 out]
              }
            }
            n217 = Bundle By Name(cluster=w429, "SpinCoater.lvclass"=w423) -> (w433:T5)
          }
          frame "Arduino_Close" {
            n218 = Unbundle By Name(w449) -> ("SpinCoater.lvclass"=w457:refnum<class "SpinCoater.lvclass">)
            n219 = property on="Arduino" class="Bool (strict)"() -> (error out=w451:errorcluster, "Value"=w450:bool)  [unwired: 2 in, 1 out]
            n220 = property on="Arduino" class="Bool (strict)"(error in=w451, "Value"=FALSE ("Arduino")) -> ()  [unwired: 1 in, 2 out]
            n221 = case shown="False" w450 {
              tunnel: w457 -> [w458 w463]
              tunnel: w456 -> [w459 w462]
              tunnel: [w459 w461] -> w455
              tunnel: [w458 w460] -> w448
              frame False {
              }
              frame True {
                n222 = call-dynamic "Close.vi"("error in (no error)"=w462, "SpinCoater in"=w463) -> ("error out"=w461:errorcluster, "SpinCoater out"=w460:refnum<class "SpinCoater.lvclass">)  [unwired: 8 in]
              }
            }
            n223 = Bundle By Name(cluster=w449, "SpinCoater.lvclass"=w448) -> (w447:T5)
          }
          frame "Arduino_LoadProgram" {
            n224 = Unbundle By Name(w473) -> ("Spin Prg v07"=w464:T2, "Numeric 1"=w472:dbl)
            n225 = Unbundle By Name(w468) -> ("SpinCoater.lvclass"=w471:refnum<class "SpinCoater.lvclass">)
            n226 = node(w472) -> (w470:dbl[unit])
            n227 = call-dynamic "Program_Load_v02.vi"("error in (no error)"=w469, "Time Start"=w470, "Program Spin Coater"=w464, "SpinCoater in"=w471) -> ("error out"=w466:errorcluster, "SpinCoater out"=w467:refnum<class "SpinCoater.lvclass">)  [unwired: 6 in]
            n228 = Bundle By Name(cluster=w468, "SpinCoater.lvclass"=w467) -> (w465:T5)
          }
          frame "Arduino_StartProgram" {
            n229 = Unbundle By Name(w481) -> ("SpinCoater.lvclass"=w478:refnum<class "SpinCoater.lvclass">)
            n230 = call-dynamic "Program_Run.vi"("error in (no error)"=w477, "SpinCoater in"=w478) -> ("error out"=w476:errorcluster)  [unwired: 8 in, 1 out]
            n231 = property on="Action" class="Str"("Value"="Measuring" ("Action")) -> ()  [unwired: 2 in, 2 out]
          }
          frame "Arduino_SetSpeed" {
            n232 = Unbundle By Name(w490) -> ("SpinCoater.lvclass"=w486:refnum<class "SpinCoater.lvclass">)
            n233 = Unbundle By Name(w489) -> ("Numeric 1"=w488:dbl)
            n234 = To Unsigned Long Integer(number=w488) -> (unsigned 32bit integer=w484:u32)
            n235 = call-dynamic "Debug_SetSpeed.vi"("error in (no error)"=w485, "Speed"=w484, "SpinCoater in"=w486) -> ("error out"=w483:errorcluster)  [unwired: 7 in, 1 out]
          }
          frame "Arduino_SetMillis" {
            n236 = Unbundle By Name(w496) -> ("SpinCoater.lvclass"=w495:refnum<class "SpinCoater.lvclass">)
            n237 = Unbundle By Name(w498) -> ("Numeric 1"=w500:dbl)
            n238 = To Unsigned Long Integer(number=w500) -> (unsigned 32bit integer=w492:u32)
            n239 = call-dynamic "Debug_SetMillis.vi"("error in (no error)"=w494, "Milliseconds"=w492, "SpinCoater in"=w495) -> ("error out"=w493:errorcluster)  [unwired: 7 in, 1 out]
          }
          frame "Arduino_StopSpin" {
            n240 = Unbundle By Name(w504) -> ("SpinCoater.lvclass"=w503:refnum<class "SpinCoater.lvclass">)
            n241 = call-dynamic "Stop_Spin.vi"("error in (no error)"=w502, "SpinCoater in"=w503) -> ("error out"=w501:errorcluster)  [unwired: 8 in, 1 out]
          }
          frame "Arduino_Shutter_SetPosition" {
            n242 = Unbundle By Name(w513) -> ("Numeric 1"=w512:dbl)
            n243 = Unbundle By Name(w515) -> ("SpinCoater.lvclass"=w514:refnum<class "SpinCoater.lvclass">)
            n244 = Number To Decimal String(number=w512) -> (decimal integer string=w511:string)  [unwired: 1 in]
            n245 = Concatenate Strings("!shu_M" ("string"), w511) -> (w509:string)
            n246 = call-dynamic "Send_String.vi"("error in (no error)"=w508, "String"=w509, "SpinCoater in"=w514) -> ("error out"=w507:errorcluster)  [unwired: 6 in, 2 out]
          }
          frame "Arduino_Shutter_Close" {
            n247 = Unbundle By Name(w522) -> ("SpinCoater.lvclass"=w521:refnum<class "SpinCoater.lvclass">)
            n248 = call-dynamic "Send_String.vi"("error in (no error)"=w520, "String"="!shuOFF" ("string"), "SpinCoater in"=w521) -> ("error out"=w519:errorcluster)  [unwired: 6 in, 2 out]
          }
          frame "Arduino_Shutter_Open" {
            n249 = Unbundle By Name(w529) -> ("SpinCoater.lvclass"=w528:refnum<class "SpinCoater.lvclass">)
            n250 = call-dynamic "Send_String.vi"("error in (no error)"=w527, "String"="!shuON" ("string"), "SpinCoater in"=w528) -> ("error out"=w526:errorcluster)  [unwired: 6 in, 2 out]
          }
          frame "Measure_Stop" {
            w538 = T6 {"QueueAction"=enum."TimeOut", "Data"=[], "Data_Raw"=[], "Data_Dark"=[], "Data_Ref"=[], "Device Information"=[], "Numeric Control"=0.0, "Boolean"=FALSE, "Wavelength"=[], "Time"=[], "Time Stamp"=timestamp(0 s since 1904-01-01), "Numeric Control 2"=0.0, "TabControl"=enum."Measure"}  # DataQueue
            n251 = Bundle By Name(cluster=w538, "QueueAction"=DataQueue_Action."Stop_Measurement") -> (w539:T6)
            n252 = Enqueue Element(queue=w536, element=w539, error in (no error)=w533) -> (queue out=w535:refnum<queue>, error out=w532:errorcluster)  [unwired: 1 in, 1 out]
          }
          frame "Measure_InSitu" {
            w580 = T9 {"QueueAction"=enum."TimeOut", "Numeric 1"=0.0, "Numeric 2"=0.0, "Boolean 1"=FALSE, "Boolean 2"=FALSE, "Spin Program"=[], "Spin Prg v07"=[], "Time Stamp"=timestamp(0 s since 1904-01-01), "TabControl"=enum."Measure"}  # Device Queue
            w587 = T9 {"QueueAction"=enum."TimeOut", "Numeric 1"=0.0, "Numeric 2"=0.0, "Boolean 1"=FALSE, "Boolean 2"=FALSE, "Spin Program"=[], "Spin Prg v07"=[], "Time Stamp"=timestamp(0 s since 1904-01-01), "TabControl"=enum."Measure"}  # Device Queue
            n253 = Bundle By Name(cluster=w587, "QueueAction"=DeviceQueue_Action."Spectrometer_SetTriggerMode", "Numeric 1"=1.0) -> (w585:T9)
            n254 = Bundle By Name(cluster=w580, "QueueAction"=DeviceQueue_Action."Spectrometer_DeviceInformation") -> (w577:T9)
            n255 = Bundle By Name(cluster=w577, "QueueAction"=DeviceQueue_Action."Spectrometer_StartMeasurement") -> (w573:T9)
            n256 = Enqueue Element(queue=w586, element=w585, error in (no error)=w542) -> (queue out=w582:refnum<queue>, error out=w583:errorcluster)  [unwired: 1 in, 1 out]
            n257 = property on="Frames" class="DigNum (strict)"() -> ("Value"=w543:i32)  [unwired: 2 in, 2 out]
            n258 = Bundle By Name(cluster=w573, "QueueAction"=DeviceQueue_Action."Arduino_StartProgram") -> (w568:T9)
            n259 = Enqueue Element(queue=w582, element=w577, error in (no error)=w583) -> (queue out=w579:refnum<queue>, error out=w578:errorcluster)  [unwired: 1 in, 1 out]
            n260 = Bundle By Name(cluster=w568, "QueueAction"=DeviceQueue_Action."Spectrometer_GetData", "Numeric 1"="Dividider Get Spectra") -> (w563:T9)
            n261 = Divide(x=w543, y="Dividider Get Spectra") -> (x/y=w575:dbl)
            n262 = Round Toward +Infinity(x=w575) -> (ceil(x): smallest int >= x=w574:dbl)
            n263 = Enqueue Element(queue=w579, element=w573, error in (no error)=w578) -> (queue out=w572:refnum<queue>, error out=w571:errorcluster)  [unwired: 1 in, 1 out]
            n264 = Enqueue Element(queue=w572, element=w568, error in (no error)=w571) -> (queue out=w569:refnum<queue>, error out=w566:errorcluster)  [unwired: 1 in, 1 out]
            n265 = for {
              N: w574 -> [_]
              shift-right: [w590] -> w565
              shift-left: w569 -> [w594]
              tunnel: w563 -> [w591]
              shift-right: [w592] -> w564
              shift-left: w566 -> [w593]
              n266 = Enqueue Element(queue=w594, element=w591, error in (no error)=w593) -> (queue out=w590:refnum<queue>, error out=w592:errorcluster)  [unwired: 1 in, 1 out]
            }
            n267 = Bundle By Name(cluster=w563, "QueueAction"=DeviceQueue_Action."Spectrometer_StopMeasurement") -> (w559:T9)
            n268 = property on="Measure_FramesSpectrometer" class="DigNum (strict)"() -> ("Value"=w545:dbl)  [unwired: 2 in, 2 out]
            n269 = Bundle By Name(cluster=w559, "QueueAction"=DeviceQueue_Action."Measure_Stop") -> (w552:T9)
            n270 = Enqueue Element(queue=w565, element=w559, error in (no error)=w564) -> (queue out=w560:refnum<queue>, error out=w561:errorcluster)  [unwired: 1 in, 1 out]
            n271 = Bundle By Name(cluster=w552, "QueueAction"=DeviceQueue_Action."Spectrometer_SetTriggerMode", "Numeric 1"=0.0) -> (w547:T9)
            n272 = Enqueue Element(queue=w560, element=w552, error in (no error)=w561) -> (queue out=w555:refnum<queue>, error out=w556:errorcluster)  [unwired: 1 in, 1 out]
            n273 = Bundle By Name(cluster=w547, "QueueAction"=DeviceQueue_Action."Spectrometer_SetFrames", "Numeric 1"=w545) -> (w544:T9)
            n274 = Enqueue Element(queue=w555, element=w547, error in (no error)=w556) -> (queue out=w554:refnum<queue>, error out=w553:errorcluster)  [unwired: 1 in, 1 out]
            n275 = Enqueue Element(queue=w554, element=w544, error in (no error)=w553) -> (queue out=w548:refnum<queue>, error out=w549:errorcluster)  [unwired: 1 in, 1 out]
          }
          frame "Measure_InSituAdvanced" {
            w681 = T9 {"QueueAction"=enum."TimeOut", "Numeric 1"=0.0, "Numeric 2"=0.0, "Boolean 1"=FALSE, "Boolean 2"=FALSE, "Spin Program"=[], "Spin Prg v07"=[], "Time Stamp"=timestamp(0 s since 1904-01-01), "TabControl"=enum."Measure"}  # Device Queue
            n276 = property on="Dividider Get Spectra" class="DigNum (strict)"() -> ("Value"=w640:u32)  [unwired: 2 in, 2 out]
            n277 = Bundle By Name(cluster=w681, "QueueAction"=DeviceQueue_Action."Spectrometer_SetTriggerMode", "Numeric 1"=1.0) -> (w636:T9)
            n278 = Bundle By Name(cluster=w636, "QueueAction"=DeviceQueue_Action."Spectrometer_DeviceInformation") -> (w673:T9)
            n279 = Bundle By Name(cluster=w673, "QueueAction"=DeviceQueue_Action."Spectrometer_StartMeasurement") -> (w669:T9)
            n280 = Enqueue Element(queue=w680, element=w636, error in (no error)=w641) -> (queue out=w677:refnum<queue>, error out=w678:errorcluster)  [unwired: 1 in, 1 out]
            n281 = Bundle By Name(cluster=w669, "QueueAction"=DeviceQueue_Action."Arduino_StartProgram") -> (w664:T9)
            n282 = property on="Frames" class="DigNum (strict)"() -> ("Value"=w642:i32)  [unwired: 2 in, 2 out]
            n283 = Unbundle By Name(w623) -> ("Time Stamp"=w622:timestamp)
            n284 = Enqueue Element(queue=w677, element=w673, error in (no error)=w678) -> (queue out=w675:refnum<queue>, error out=w674:errorcluster)  [unwired: 1 in, 1 out]
            n285 = Divide(x=w642, y=w640) -> (x/y=w671:dbl)
            n286 = Bundle By Name(cluster=w664, "QueueAction"=DeviceQueue_Action."Spectrometer_GetData", "Numeric 1"=w640) -> (w659:T9)
            n287 = Round Toward +Infinity(x=w671) -> (ceil(x): smallest int >= x=w670:dbl)
            n288 = Enqueue Element(queue=w675, element=w669, error in (no error)=w674) -> (queue out=w668:refnum<queue>, error out=w667:errorcluster)  [unwired: 1 in, 1 out]
            n289 = Enqueue Element(queue=w668, element=w664, error in (no error)=w667) -> (queue out=w665:refnum<queue>, error out=w662:errorcluster)  [unwired: 1 in, 1 out]
            n290 = Bundle By Name(cluster=w659, "QueueAction"=DeviceQueue_Action."Spectrometer_StopMeasurement") -> (w655:T9)
            n291 = for {
              N: w670 -> [_]
              shift-right: [w731] -> w661
              shift-left: w665 -> [w735]
              tunnel: w659 -> [w732]
              shift-right: [w733] -> w660
              shift-left: w662 -> [w734]
              n292 = Enqueue Element(queue=w735, element=w732, error in (no error)=w734) -> (queue out=w731:refnum<queue>, error out=w733:errorcluster)  [unwired: 1 in, 1 out]
            }
            n293 = property on="Measure_FramesSpectrometer" class="DigNum (strict)"() -> ("Value"=w643:dbl)  [unwired: 2 in, 2 out]
            n294 = property on="periodic time" class="DigNum (strict)"() -> ("Value"=w635:dbl[unit])  [unwired: 2 in, 2 out]
            n295 = Bundle By Name(cluster=w655, "QueueAction"=DeviceQueue_Action."Measure_Stop") -> (w648:T9)
            n296 = property on="Duration after" class="DigNum (strict)"() -> ("Value"=w634:dbl[unit])  [unwired: 2 in, 2 out]
            n297 = node(w635) -> (w605:dbl)
            n298 = property on="periodic time" class="DigNum (strict)"() -> ("Value"=w633:dbl[unit])  [unwired: 2 in, 2 out]
            n299 = Bundle By Name(cluster=w648, "QueueAction"=DeviceQueue_Action."Spectrometer_SetTriggerMode", "Numeric 1"=0.0) -> (w645:T9)
            n300 = Enqueue Element(queue=w661, element=w655, error in (no error)=w660) -> (queue out=w656:refnum<queue>, error out=w657:errorcluster)  [unwired: 1 in, 1 out]
            n301 = node(w634) -> (w628:dbl)
            n302 = Bundle By Name(cluster=w645, "QueueAction"=DeviceQueue_Action."Spectrometer_SetFrames", "Numeric 1"=w643) -> (w625:T9)
            n303 = Enqueue Element(queue=w656, element=w648, error in (no error)=w657) -> (queue out=w651:refnum<queue>, error out=w652:errorcluster)  [unwired: 1 in, 1 out]
            n304 = node(w633) -> (w627:dbl)
            n305 = Bundle By Name(cluster=w625, "QueueAction"=DeviceQueue_Action."Wait", "Numeric 1"=w605) -> (w607:T9)
            n306 = Enqueue Element(queue=w651, element=w645, error in (no error)=w652) -> (queue out=w650:refnum<queue>, error out=w649:errorcluster)  [unwired: 1 in, 1 out]
            n307 = Not Equal To 0?(x=w627) -> (x != 0?=w631:bool)
            n308 = Not Equal To 0?(x=w628) -> (x != 0?=w632:bool)
            n309 = Divide(x=w628, y=w627) -> (x/y=w629:dbl)
            n310 = Bundle By Name(cluster=w607, "QueueAction"=DeviceQueue_Action."Spectrometer_MeasureAdvanced", "Time Stamp"=w622) -> (w606:T9)
            n311 = And(x=w632, y=w631) -> (x .and. y?=w630:bool)
            n312 = Round Toward +Infinity(x=w629) -> (ceil(x): smallest int >= x=w626:dbl)
            n313 = Enqueue Element(queue=w650, element=w625, error in (no error)=w649) -> (queue out=w639:refnum<queue>, error out=w638:errorcluster)  [unwired: 1 in, 1 out]
            n314 = Bundle By Name(cluster=w606, "QueueAction"=DeviceQueue_Action."Arduino_SetSpeed", "Numeric 1"=1500.0) -> (w617:T9)
            n315 = Bundle By Name(cluster=w617, "Numeric 1"=0.0) -> (w609:T9)
            n316 = property on="Measure_FrameRate" class="DigNum (strict)"() -> ("Value"=w614:dbl[unit])  [unwired: 2 in, 2 out]
            n317 = property on="Measure_FramesSpectrometer" class="DigNum (strict)"() -> ("Value"=w613:dbl)  [unwired: 2 in, 2 out]
            n318 = Divide(x=w613, y=w614) -> (x/y=w615:dbl[unit])
            n319 = Bundle By Name(cluster=w607, "Numeric 1"=1.0) -> (w610:T9)
            n320 = node(w615) -> (w604:dbl)
            n321 = Subtract(x=w605, y=w604) -> (x-y=w603:dbl)
            n322 = Bundle By Name(cluster=w607, "Numeric 1"=w603) -> (w602:T9)
            n323 = Round Toward +Infinity(x=w604) -> (ceil(x): smallest int >= x=w616:dbl)
            n324 = Add(x=w616, y=2.0) -> (x+y=w611:dbl)
            n325 = Bundle By Name(cluster=w610, "Numeric 1"=w611) -> (w599:T9)
            n326 = case shown="True" w630 {
              tunnel: w639 -> [w685 w687]
              tunnel: w638 -> [w684 w690]
              tunnel: w626 -> [_ w703]
              tunnel: w606 -> [_ w702]
              tunnel: w602 -> [_ w698]
              tunnel: w617 -> [_ w697]
              tunnel: w610 -> [_ w696]
              tunnel: w606 -> [_ w695]
              tunnel: w599 -> [_ w694]
              tunnel: w609 -> [_ w693]
              tunnel: [w684 w692] -> w601
              tunnel: [w685 w691] -> w600
              tunnel: w607 -> [_ w686]
              frame False {
              }
              frame True {
                n327 = Enqueue Element(queue=w687, element=w686, error in (no error)=w690) -> (queue out=w688:refnum<queue>, error out=w689:errorcluster)  [unwired: 1 in, 1 out]
                n328 = for {
                  N: w703 -> [_]
                  shift-right: [w724] -> w700
                  shift-left: w688 -> [w730]
                  shift-right: [w723] -> w699
                  shift-left: w689 -> [w729]
                  tunnel: w702 -> [w728]
                  tunnel: w698 -> [w725]
                  n329 = Enqueue Element(queue=w730, element=w728, error in (no error)=w729) -> (queue out=w726:refnum<queue>, error out=w727:errorcluster)  [unwired: 1 in, 1 out]
                  n330 = Enqueue Element(queue=w726, element=w725, error in (no error)=w727) -> (queue out=w724:refnum<queue>, error out=w723:errorcluster)  [unwired: 1 in, 1 out]
                }
                n331 = case shown="True" "Spin at end" {
                  tunnel: w700 -> [w705 w722]
                  tunnel: w699 -> [w704 w721]
                  tunnel: w697 -> [_ w716]
                  tunnel: w696 -> [_ w715]
                  tunnel: w695 -> [_ w714]
                  tunnel: w694 -> [_ w709]
                  tunnel: w693 -> [_ w708]
                  tunnel: [w704 w707] -> w692
                  tunnel: [w705 w706] -> w691
                  frame False {
                  }
                  frame True {
                    n332 = Enqueue Element(queue=w722, element=w716, error in (no error)=w721) -> (queue out=w720:refnum<queue>, error out=w719:errorcluster)  [unwired: 1 in, 1 out]
                    n333 = Enqueue Element(queue=w720, element=w715, error in (no error)=w719) -> (queue out=w718:refnum<queue>, error out=w717:errorcluster)  [unwired: 1 in, 1 out]
                    n334 = Enqueue Element(queue=w718, element=w714, error in (no error)=w717) -> (queue out=w713:refnum<queue>, error out=w712:errorcluster)  [unwired: 1 in, 1 out]
                    n335 = Enqueue Element(queue=w713, element=w709, error in (no error)=w712) -> (queue out=w710:refnum<queue>, error out=w711:errorcluster)  [unwired: 1 in, 1 out]
                    n336 = Enqueue Element(queue=w710, element=w708, error in (no error)=w711) -> (queue out=w706:refnum<queue>, error out=w707:errorcluster)  [unwired: 1 in, 1 out]
                  }
                }
              }
            }
            n337 = Bundle By Name(cluster=w599, "QueueAction"=DeviceQueue_Action."Arduino_Shutter_Close") -> (w598:T9)
            n338 = Enqueue Element(queue=w600, element=w598, error in (no error)=w601) -> (queue out=w596:refnum<queue>, error out=w595:errorcluster)  [unwired: 1 in, 1 out]
            "Nr After Spin" <- u16 0 ("Nr After Spin")
          }
          frame "Measure_Spectrum" {
            n339 = Unbundle By Name(w736) -> ("Time Stamp"=w737:timestamp)
            n340 = Bundle By Name(cluster=w736, "QueueAction"=DeviceQueue_Action."Spectrometer_Measure", "Time Stamp"=w737) -> (w742:T9)
            n341 = Bundle By Name(cluster=w742, "QueueAction"=DeviceQueue_Action."Measure_Stop") -> (w740:T9)
            n342 = Enqueue Element(queue=w748, element=w742, error in (no error)=w747) -> (queue out=w743:refnum<queue>, error out=w744:errorcluster)  [unwired: 1 in, 1 out]
            n343 = Enqueue Element(queue=w743, element=w740, error in (no error)=w744) -> (queue out=w739:refnum<queue>, error out=w738:errorcluster)  [unwired: 1 in, 1 out]
          }
          frame "Measure_SpectralStability" {
            n344 = Bundle By Name(cluster=w752, "QueueAction"=DeviceQueue_Action."Spectrometer_DeviceInformation") -> (w755:T9)
            n345 = property on="SpectralStability_\nFrameRate" class="DigNum (strict)"() -> ("Value"=w775:dbl[unit])  [unwired: 2 in, 2 out]
            n346 = property on="SpectralStability_\nFramesSpectrometer" class="DigNum (strict)"() -> ("Value"=w776:dbl)  [unwired: 2 in, 2 out]
            n347 = Bundle By Name(cluster=w755, "QueueAction"=DeviceQueue_Action."Spectrometer_Measure") -> (w754:T9)
            n348 = Enqueue Element(queue=w758, element=w755, error in (no error)=w757) -> (queue out=w760:refnum<queue>, error out=w759:errorcluster)  [unwired: 1 in, 1 out]
            n349 = Divide(x=w776, y=w775) -> (x/y=w770:dbl[unit])
            n350 = Unbundle By Name(w752) -> ("Numeric 1"=w751:dbl)
            n351 = Subtract(x="SpectralStability_\nPeriodicTime", y=w770) -> (x-y=w769:dbl[unit])
            n352 = Enqueue Element(queue=w760, element=w754, error in (no error)=w759) -> (queue out=w774:refnum<queue>, error out=w773:errorcluster)  [unwired: 1 in, 1 out]
            n353 = node(w769) -> (w768:dbl)
            n354 = Decrement(x=w751) -> (x-1=w750:dbl)
            n355 = Bundle By Name(cluster=w754, "QueueAction"=DeviceQueue_Action."Wait", "Numeric 1"=w768) -> (w764:T9)
            n356 = for {
              N: w750 -> [_]
              shift-right: [w780] -> w767
              shift-left: w774 -> [w786]
              shift-right: [w779] -> w766
              shift-left: w773 -> [w785]
              tunnel: w764 -> [w782]
              tunnel: w754 -> [w781]
              n357 = Enqueue Element(queue=w786, element=w782, error in (no error)=w785) -> (queue out=w784:refnum<queue>, error out=w783:errorcluster)  [unwired: 1 in, 1 out]
              n358 = Enqueue Element(queue=w784, element=w781, error in (no error)=w783) -> (queue out=w780:refnum<queue>, error out=w779:errorcluster)  [unwired: 1 in, 1 out]
            }
            n359 = Bundle By Name(cluster=w764, "QueueAction"=DeviceQueue_Action."Measure_Stop") -> (w763:T9)
            n360 = Enqueue Element(queue=w767, element=w763, error in (no error)=w766) -> (queue out=w761:refnum<queue>, error out=w762:errorcluster)  [unwired: 1 in, 1 out]
          }
        }
      }
      frame Error {
        w791 = T12 4 items=["no dialog", "OK message", "continue or stop message", "OK message + warnings", "continue/stop + warnings"] ("type of dialog (OK msg:1)")
        n361 = call <vilib>:"General Error Handler.vi"("type of dialog (OK msg:1)"=w791, "error in (no error)"=w792) -> ("error out"=w790:errorcluster)  [unwired: 9 in, 4 out]
        n362 = call <vilib>:"Clear Errors.vi"("error in (no error)"=w790) -> ("error out"=w789:errorcluster)  [unwired: 5 in, 1 out]
      }
    }
  }
  n363 = while {
    shift-right: [w794] -> _
    shift-left: w8 -> [w800]
    shift-right: [w795] -> _
    shift-left: w7 -> [w799]
    shift-right: [w796] -> _
    shift-left: w6 -> [w798]
    stop <- w797 stop-if-true
    # "Consumer Data"
    n364 = case shown="No Error" w800 {
      selector: w800 -> [w811 w1498]
      tunnel: w799 -> [w810 w1499]
      tunnel: w798 -> [w808 w1496]
      tunnel: [w807 _] -> w797
      tunnel: [w806 w1496] -> w796
      tunnel: [w805 w1499] -> w795
      tunnel: [w803 w1497] -> w794
      frame No Error {
        n365 = Dequeue Element(queue=w810, error in (no error)=w811) -> (queue out=w804:refnum<queue>, element=w801:T6, error out=w802:errorcluster)  [unwired: 1 in, 1 out]
        n366 = Unbundle By Name(w801) -> ("QueueAction"=w809:T7)
        n367 = case shown="\"Save_InSitu\"" w809 {
          tunnel: w808 -> [w812 w817 w823 w996 w1101 w1203 w1411 w1447 w1456 w1478 w1491]
          tunnel: [_ TRUE _ _ _ _ _ _ _ _ _] -> w807
          tunnel: [w812 w817 w823 w996 w1101 w1194 w1411 w1451 w1470 w1477 w1491] -> w806
          tunnel: [w814 w816 w833 w1002 w1107 w1187 w1434 w1452 w1471 w1474 w1493] -> w805
          tunnel: w804 -> [w814 w816 w831 w1003 w1108 w1198 w1434 w1452 w1471 w1474 w1493]
          tunnel: [w813 w815 w832 w1001 w1106 w1188 w1433 w1453 w1472 w1475 w1492] -> w803
          tunnel: w802 -> [w813 w815 w830 w1004 w1109 w1197 w1433 w1453 w1472 w1475 w1492]
          tunnel: w801 -> [_ _ w825 _ _ w1190 w1424 w1454 w1473 w1476 w1482]
          frame "TimeOut", Default {
          }
          frame "Close_Program" {
          }
          frame "Measure_InSituSpinCoating" {
            w828 = T6 {"QueueAction"=enum."TimeOut", "Data"=[], "Data_Raw"=[], "Data_Dark"=[], "Data_Ref"=[], "Device Information"=[], "Numeric Control"=0.0, "Boolean"=FALSE, "Wavelength"=[], "Time"=[], "Time Stamp"=timestamp(0 s since 1904-01-01), "Numeric Control 2"=0.0, "TabControl"=enum."Measure"}  # DataQueue
            n368 = property on="Seconds to\nSpin Start" class="DigNum (strict)"() -> ("Value"=w820:dbl[unit])  [unwired: 2 in, 2 out]
            n369 = Unbundle By Name(w825) -> ("Time Stamp"=w824:timestamp)
            n370 = node(w820) -> (w819:dbl)
            n371 = Obtain Queue(name (unnamed)="Temp", element data type=w828) -> (queue out=w827:refnum<queue>)  [unwired: 3 in, 2 out]
            n372 = while {
              shift-right: [w841] -> w833
              shift-left: w831 -> [w850]
              shift-right: [w842] -> w832
              shift-left: w830 -> [w849]
              shift-right: [w843] -> w826
              shift-left: w827 -> [w844]
              tunnel: w824 -> [w837]
              shift-right: [w838] -> _
              shift-left: string[] [] ("Device Information") -> [w839]
              border: FALSE -> [_]
              tunnel: w819 -> [w834]
              stop <- w840 stop-if-true
              n373 = Dequeue Element(queue=w850, error in (no error)=w849) -> (queue out=w845:refnum<queue>, element=w847:T6, error out=w846:errorcluster)  [unwired: 1 in, 1 out]
              n374 = Unbundle By Name(w847) -> ("QueueAction"=w848:T7)
              n375 = feedback #1() -> (w836:bool)
              n376 = case shown="\"Transfer_Settings\"" w848 {
                tunnel: w847 -> [w858 w867 _ w913 w950 w994]
                tunnel: w846 -> [w857 w868 w874 w910 w941 w991]
                tunnel: w845 -> [w853 w869 w873 w909 w949 w992]
                tunnel: w844 -> [w856 w864 w875 w904 w938 w995]
                tunnel: [w855 w864 w870 w901 w938 w995] -> w843
                tunnel: [w854 w865 w872 w900 w939 w991] -> w842
                tunnel: [w853 w866 w871 w899 w949 w992] -> w841
                tunnel: [_ TRUE TRUE TRUE _ _] -> w840
                tunnel: w839 -> [w852 w862 w882 w911 w936 _]
                tunnel: [w852 w862 w882 w911 w936 w993] -> w838
                tunnel: w837 -> [_ _ _ w912 w951 _]
                tunnel: w836 -> [w851 w861 w881 w898 w934 w990]
                tunnel: [w851 w861 w881 w898 TRUE w990] -> w835
                tunnel: w834 -> [_ _ _ w895 _ _]
                frame Default {
                  n377 = Enqueue Element(queue=w856, element=w858, error in (no error)=w857) -> (queue out=w855:refnum<queue>, error out=w854:errorcluster)  [unwired: 1 in, 1 out]
                }
                frame "Close_Program" {
                  n378 = Enqueue Element At Opposite End(queue=w869, element=w867, error in (no error)=w868) -> (queue out=w866:refnum<queue>, error out=w865:errorcluster)  [unwired: 1 in, 1 out]
                  n379 = property on="Time.spin" class="Ref (strict)"() -> ("Value"=w859:refnum<file>)  [unwired: 2 in, 2 out]
                  n380 = property on="Meas.spin" class="Ref (strict)"() -> ("Value"=w860:refnum<file>)  [unwired: 2 in, 2 out]
                  n381 = Close File(refnum=w860) -> ()  [unwired: 1 in, 2 out]
                  n382 = Close File(refnum=w859) -> ()  [unwired: 1 in, 2 out]
                }
                frame "Abort" {
                  n383 = property on="Time.spin" class="Ref (strict)"() -> ("Value"=w879:refnum<file>)  [unwired: 2 in, 2 out]
                  n384 = Get Queue Status(queue=w875) -> (queue out=w876:refnum<queue>, # elements in queue=w877:i32)  [unwired: 2 in, 6 out]
                  n385 = property on="Meas.spin" class="Ref (strict)"() -> ("Value"=w880:refnum<file>)  [unwired: 2 in, 2 out]
                  n386 = Close File(refnum=w880) -> ()  [unwired: 1 in, 2 out]
                  n387 = Close File(refnum=w879) -> ()  [unwired: 1 in, 2 out]
                  n388 = for {
                    N: w877 -> [_]
                    shift-right: [w889] -> w870
                    shift-left: w876 -> [w890]
                    shift-right: [w886] -> w871
                    shift-left: w873 -> [w887]
                    shift-right: [w884] -> w872
                    shift-left: w874 -> [w885]
                    n389 = Dequeue Element(queue=w890) -> (queue out=w889:refnum<queue>, element=w888:T6)  [unwired: 2 in, 2 out]
                    n390 = Enqueue Element(queue=w887, element=w888, error in (no error)=w885) -> (queue out=w886:refnum<queue>, error out=w884:errorcluster)  [unwired: 1 in, 1 out]
                  }
                  n391 = property on="StartMeasurement_Button" class="Bool (strict)"("Value"=FALSE ("StartMeasurement_Button")) -> ()  [unwired: 2 in, 2 out]
                }
                frame "Stop_Measurement" {
                  n392 = property on="Automatically \nadjust count" class="Bool (strict)"() -> ("Value"=w892:bool)  [unwired: 2 in, 2 out]
                  n393 = property on="Reset Count\nafter Spin Coating" class="Bool (strict)"() -> ("Value"=w893:bool)  [unwired: 2 in, 2 out]
                  n394 = Or(x=w892, y=w893) -> (x .or. y?=w891:bool)
                  n395 = Bundle By Name(cluster=w913, "QueueAction"=DataQueue_Action."Save_InSitu", "Time Stamp"=w912, "Device Information"=w911, "Numeric Control"=w895) -> (w908:T6)
                  n396 = case shown="True" w891 {
                    frame False {
                    }
                    frame True {
                      n397 = property on="Spectra \nCount" class="DigNum (strict)"("Value"=u16 0 ("Spectra Count")) -> ()  [unwired: 2 in, 2 out]
                    }
                  }
                  n398 = Enqueue Element(queue=w909, element=w908, error in (no error)=w910) -> (queue out=w906:refnum<queue>, error out=w905:errorcluster)  [unwired: 1 in, 1 out]
                  n399 = Get Queue Status(queue=w904) -> (queue out=w902:refnum<queue>, # elements in queue=w903:i32)  [unwired: 2 in, 6 out]
                  n400 = property on="Time.spin" class="Ref (strict)"() -> ("Value"=w896:refnum<file>)  [unwired: 2 in, 2 out]
                  n401 = property on="StartMeasurement_Button" class="Bool (strict)"("Value"=FALSE ("StartMeasurement_Button")) -> ()  [unwired: 2 in, 2 out]
                  n402 = property on="Meas.spin" class="Ref (strict)"() -> ("Value"=w897:refnum<file>)  [unwired: 2 in, 2 out]
                  n403 = for {
                    N: w903 -> [_]
                    shift-right: [w921] -> w901
                    shift-left: w902 -> [w922]
                    shift-right: [w918] -> w899
                    shift-left: w906 -> [w919]
                    shift-right: [w916] -> w900
                    shift-left: w905 -> [w917]
                    n404 = Dequeue Element(queue=w922) -> (queue out=w921:refnum<queue>, element=w920:T6)  [unwired: 2 in, 2 out]
                    n405 = Enqueue Element(queue=w919, element=w920, error in (no error)=w917) -> (queue out=w918:refnum<queue>, error out=w916:errorcluster)  [unwired: 1 in, 1 out]
                  }
                  n406 = Close File(refnum=w897) -> ()  [unwired: 1 in, 2 out]
                  n407 = Close File(refnum=w896) -> ()  [unwired: 1 in, 2 out]
                }
                frame "Spectrometer_Measure" {
                  w924 = FALSE ("prepend array or string size? (T)")
                  w937 = enum16{"start", "end", "current"}."end" ("from (0:start)")
                  n408 = Unbundle By Name(w950) -> ("Data_Raw"=w946:T11, "Time"=w940:dbl[])
                  n409 = Index Array(array=w946, index=0) -> (element=w945:T14)
                  n410 = To Unsigned Long Integer(number=w940) -> (unsigned 32bit integer=w926:u32[])
                  n411 = Unbundle By Name(w945) -> ("Image"=w923:dbl[][][])
                  n412 = case shown="False" w934 {
                    tunnel: w951 -> [w983 _]
                    tunnel: w941 -> [w978 w989]
                    tunnel: [w964 w989] -> w928
                    tunnel: [w952 _] -> w929
                    tunnel: [w963 w988] -> w931
                    tunnel: [w953 w987] -> w930
                    tunnel: w923 -> [w961 _]
                    frame False {
                      w973 = T13."open or create" ("operation (0:open)")
                      w972 = "_" ("string")
                      n413 = property on="Measure_FileName" class="Str"() -> ("Value"=w981:string)  [unwired: 2 in, 2 out]
                      n414 = Concatenate Strings(w981, "_meas.spin" ("string")) -> (w984:string)
                      n415 = Concatenate Strings(w981, "_time.spin" ("string")) -> (w976:string)
                      n416 = Format Date/Time String(time format string (%c)="%Y%m%d_%H%M%S", seconds (now)=w983) -> (date/time string=w977:string)  [unwired: 1 in]
                      n417 = property on="Measure_SavePath" class="Path"() -> ("Value"=w955:path)  [unwired: 2 in, 2 out]
                      n418 = Concatenate Strings(w977, w972, w984) -> (w982:string)
                      n419 = Concatenate Strings(w977, w972, w976) -> (w975:string)
                      n420 = property on="Frames" class="DigNum (strict)"() -> ("Value"=w954:i32)  [unwired: 2 in, 2 out]
                      n421 = Build Path(base path=w955, name or relative path=w982) -> (appended path=w979:path)
                      n422 = Build Path(base path=w955, name or relative path=w975) -> (appended path=w974:path)
                      n423 = Array Size(array=w961) -> (size(s)=w960:i32[])
                      n424 = Open/Create/Replace File(file path (use dialog)=w979, error in=w978, operation (0:open)=w973) -> (refnum out=w971:refnum<file>, error out=w970:errorcluster)  [unwired: 3 in, 1 out]
                      "Meas.spin" <- w971
                      n425 = Open/Create/Replace File(file path (use dialog)=w974, error in=w978, operation (0:open)=w973) -> (refnum out=w969:refnum<file>, error out=w968:errorcluster)  [unwired: 3 in, 1 out]
                      n426 = Write to Binary File(file (use dialog)=w971, data=w954, error in=w970) -> (refnum out=w967:refnum<file>, error out=w966:errorcluster)  [unwired: 3 in, 1 out]
                      n427 = Index Array(array=w960, index #1=2 ("index"), index #2=1 ("index")) -> (element #1=w956:i32, element #2=w957:i32)
                      n428 = Write to Binary File(file (use dialog)=w969, data=w954, error in=w968) -> (refnum out=w953:refnum<file>, error out=w952:errorcluster)  [unwired: 3 in, 1 out]
                      "Time.spin" <- w953
                      n429 = Write to Binary File(file (use dialog)=w967, data=w957, error in=w966) -> (refnum out=w962:refnum<file>, error out=w965:errorcluster)  [unwired: 3 in, 1 out]
                      n430 = Write to Binary File(file (use dialog)=w962, data=w956, error in=w965) -> (refnum out=w963:refnum<file>, error out=w964:errorcluster)  [unwired: 3 in, 1 out]
                    }
                    frame True {
                      n431 = property on="Time.spin" class="Ref (strict)"() -> ("Value"=w987:refnum<file>)  [unwired: 2 in, 2 out]
                      n432 = property on="Meas.spin" class="Ref (strict)"() -> ("Value"=w988:refnum<file>)  [unwired: 2 in, 2 out]
                    }
                  }
                  n433 = To Unsigned Word Integer(number=w923) -> (unsigned 16bit integer=w925:u16[][][])
                  n434 = Merge Errors(w928, w929) -> (w927:errorcluster)
                  n435 = Set File Position(refnum=w931, from (0:start)=w937, error in=w927) -> (refnum out=w943:refnum<file>, error out=w942:errorcluster)  [unwired: 1 in]
                  n436 = Set File Position(refnum=w930, from (0:start)=w937, error in=w927) -> (refnum out=w948:refnum<file>, error out=w947:errorcluster)  [unwired: 1 in]
                  n437 = Write to Binary File(file (use dialog)=w948, data=w926, error in=w947, 5:w924) -> (error out=w932:errorcluster)  [unwired: 2 in, 2 out]
                  n438 = Write to Binary File(file (use dialog)=w943, data=w925, error in=w942, 5:w924) -> (error out=w933:errorcluster)  [unwired: 2 in, 2 out]
                  n439 = Merge Errors(w933, w932) -> (w939:errorcluster)
                }
                frame "Transfer_Settings" {
                  n440 = Unbundle By Name(w994) -> ("Device Information"=w993:string[])
                }
              }
              n441 = feedback-in #1(w835) -> ()
            }
            n442 = Release Queue(queue=w826) -> ()  [unwired: 2 in, 3 out]
          }
          frame "Measure_Spectrum" {
            w999 = T6 {"QueueAction"=enum."TimeOut", "Data"=[], "Data_Raw"=[], "Data_Dark"=[], "Data_Ref"=[], "Device Information"=[], "Numeric Control"=0.0, "Boolean"=FALSE, "Wavelength"=[], "Time"=[], "Time Stamp"=timestamp(0 s since 1904-01-01), "Numeric Control 2"=0.0, "TabControl"=enum."Measure"}  # DataQueue
            n443 = Obtain Queue(name (unnamed)="Temp", element data type=w999) -> (queue out=w998:refnum<queue>)  [unwired: 3 in, 2 out]
            n444 = while {
              shift-right: [w1008] -> w1002
              shift-left: w1003 -> [w1016]
              shift-right: [w1009] -> w1001
              shift-left: w1004 -> [w1017]
              shift-right: [w1010] -> w997
              shift-left: w998 -> [w1012]
              tunnel: w996 -> [w1006]
              stop <- w1007 stop-if-true
              n445 = Dequeue Element(queue=w1016, error in (no error)=w1017) -> (queue out=w1014:refnum<queue>, element=w1011:T6, error out=w1013:errorcluster)  [unwired: 1 in, 1 out]
              n446 = Unbundle By Name(w1011) -> ("QueueAction"=w1015:T7, "TabControl"=w1005:T8)
              n447 = case shown="\"Spectrometer_Measure\"" w1015 {
                tunnel: w1014 -> [w1018 w1046 w1086]
                tunnel: w1013 -> [w1021 w1056 w1085]
                tunnel: w1012 -> [w1023 w1062 w1088]
                tunnel: w1011 -> [w1019 w1035 _]
                tunnel: [w1022 w1062 w1084] -> w1010
                tunnel: [w1020 w1047 w1082] -> w1009
                tunnel: [w1018 w1046 w1083] -> w1008
                tunnel: [_ _ TRUE] -> w1007
                tunnel: w1006 -> [_ w1039 _]
                tunnel: w1005 -> [_ w1033 w1080]
                frame Default {
                  n448 = Enqueue Element(queue=w1023, element=w1019, error in (no error)=w1021) -> (queue out=w1022:refnum<queue>, error out=w1020:errorcluster)  [unwired: 1 in, 1 out]
                }
                frame "Spectrometer_Measure" {
                  n449 = Unbundle By Name(w1035) -> ("Data_Raw"=w1053:T11)
                  n450 = case shown="\"Spectral Stability\"" w1033 {
                    tunnel: [w1075 "SpectralStability_SavePath"] -> w1026
                    tunnel: [w1074 "SpectralStability_FileName"] -> w1024
                    tunnel: [w1070 "SpectralStability_Comments"] -> w1027
                    frame "Measure", Default {
                      n451 = property on="Spectra Count" class="DigNum (strict)"() -> ("Value"=w1076:u16)  [unwired: 2 in, 2 out]
                      n452 = property on="Measure_SavePath" class="Path"() -> ("Value"=w1075:path)  [unwired: 2 in, 2 out]
                      n453 = property on="Measure_Comments" class="Str"() -> ("Value"=w1070:string)  [unwired: 2 in, 2 out]
                      n454 = property on="Measure_FileName" class="Str"() -> ("Value"=w1071:string)  [unwired: 2 in, 2 out]
                      n455 = Number To Decimal String(number=w1076) -> (decimal integer string=w1072:string)  [unwired: 1 in]
                      n456 = Concatenate Strings(w1071, "_", w1072) -> (w1074:string)
                    }
                    frame "Spectral Stability" {
                    }
                  }
                  n457 = Index Array(array=w1053, index=0) -> (element=w1051:T14)
                  n458 = Unbundle By Name(w1035) -> ("Time Stamp"=w1034:timestamp)
                  n459 = Unbundle By Name(w1051) -> ("Image"=w1029:dbl[][][])
                  n460 = Index Array(array=w1029, index (dim 1)=0 ("disabled index (row)")) -> (element=w1045:dbl[][])  [unwired: 2 in]
                  n461 = Transpose 2D Array(2D array=w1045) -> (transposed array=w1042:dbl[][])
                  n462 = Format Date/Time String(time format string (%c)="%Y%m%d_%H%M%S", seconds (now)=w1034) -> (date/time string=w1060:string)  [unwired: 1 in]
                  n463 = Matrix Size(0:w1042) -> (2:w1043:i32)  [unwired: 1 out]
                  n464 = Empty String/Path?(string/path=w1027) -> (empty?=w1028:bool)
                  n465 = Reciprocal(x=w1043) -> (1/x=w1044:dbl)
                  n466 = Concatenate Strings(w1060, "_") -> (w1025:string)
                  n467 = case shown="False" w1028 {
                    tunnel: w1027 -> [w1069 _]
                    tunnel: w1026 -> [w1068 _]
                    tunnel: w1025 -> [w1067 _]
                    tunnel: w1024 -> [w1066 _]
                    frame False {
                      n468 = Concatenate Strings(w1067, w1066, "_comments.txt" ("string")) -> (w1063:string)
                      n469 = Build Path(base path=w1068, name or relative path=w1063) -> (appended path=w1064:path)
                      n470 = Write to Text File(file (use dialog)=w1064, text=w1069) -> ()  [unwired: 2 in, 3 out]
                    }
                    frame True {
                    }
                  }
                  n471 = Initialize Array(w1044, w1043) -> (w1041:dbl[])
                  n472 = Concatenate Strings(w1025, w1024, ".spectra" ("string")) -> (w1031:string)
                  n473 = Unbundle By Name(w1039) -> ("Wavlength"=w1036:dbl[unit][])
                  n474 = call-poly <vilib>:"A x B.vi"("Vector"=w1041, "A"=w1042) -> ("A x Vector"=w1030:dbl[])  [unwired: 1 out]
                  n475 = Build Path(base path=w1026, name or relative path=w1031) -> (appended path=w1058:path)
                  n476 = Bundle("Wavlength"=w1036, "A x Vector"=w1030) -> (w1038:T15)  [unwired: 1 in]
                  n477 = Open/Create/Replace File(file path (use dialog)=w1058, error in=w1056, operation (0:open)=T13."open or create") -> (refnum out=w1055:refnum<file>, error out=w1054:errorcluster)  [unwired: 3 in, 1 out]
                  n478 = Build Array(w1038) -> (w1037:T16)
                  n479 = To Unsigned Word Integer(number=w1029) -> (unsigned 16bit integer=w1050:u16[][][])
                  n480 = property on="Measure_Graph" class="XYGraph (strict)"("Value"=w1037) -> ()  [unwired: 2 in, 2 out]
                  n481 = Write to Binary File(file (use dialog)=w1055, data=w1050, error in=w1054) -> (refnum out=w1048:refnum<file>, error out=w1049:errorcluster)  [unwired: 3 in, 1 out]
                  n482 = Close File(refnum=w1048, error in=w1049) -> (error out=w1047:errorcluster)  [unwired: 1 out]
                }
                frame "Stop_Measurement" {
                  w1081 = FALSE ("Measure Spectrum")
                  n483 = case shown="Default" w1080 {
                    frame Default {
                    }
                    frame "Measure" {
                      n484 = property on="Automatically \nadjust count" class="Bool (strict)"() -> ("Value"=w1091:bool)  [unwired: 2 in, 2 out]
                      n485 = case shown="True" w1091 {
                        frame False {
                        }
                        frame True {
                          n486 = Increment(x="Spectra Count") -> (x+1=w1092:u16)
                          n487 = property on="Spectra Count" class="DigNum (strict)"("Value"=w1092) -> ()  [unwired: 2 in, 2 out]
                        }
                      }
                    }
                  }
                  n488 = Get Queue Status(queue=w1088) -> (queue out=w1089:refnum<queue>, # elements in queue=w1087:i32)  [unwired: 2 in, 6 out]
                  n489 = property on="SpectralStability_MeasureSpectrum" class="Bool (strict)"("Value"=w1081) -> ()  [unwired: 2 in, 2 out]
                  n490 = property on="Measure_MeasureSpectrum" class="Bool (strict)"("Value"=w1081) -> ()  [unwired: 2 in, 2 out]
                  n491 = for {
                    N: w1087 -> [_]
                    shift-right: [w1099] -> w1084
                    shift-left: w1089 -> [w1100]
                    shift-right: [w1096] -> w1083
                    shift-left: w1086 -> [w1097]
                    shift-right: [w1094] -> w1082
                    shift-left: w1085 -> [w1095]
                    n492 = Dequeue Element(queue=w1100) -> (queue out=w1099:refnum<queue>, element=w1098:T6)  [unwired: 2 in, 2 out]
                    n493 = Enqueue Element(queue=w1097, element=w1098, error in (no error)=w1095) -> (queue out=w1096:refnum<queue>, error out=w1094:errorcluster)  [unwired: 1 in, 1 out]
                  }
                }
              }
            }
            n494 = Release Queue(queue=w997) -> ()  [unwired: 2 in, 3 out]
          }
          frame "Measure_SpectrumAdvanced" {
            w1104 = T6 {"QueueAction"=enum."TimeOut", "Data"=[], "Data_Raw"=[], "Data_Dark"=[], "Data_Ref"=[], "Device Information"=[], "Numeric Control"=0.0, "Boolean"=FALSE, "Wavelength"=[], "Time"=[], "Time Stamp"=timestamp(0 s since 1904-01-01), "Numeric Control 2"=0.0, "TabControl"=enum."Measure"}  # DataQueue
            n495 = Obtain Queue(name (unnamed)="Temp", element data type=w1104) -> (queue out=w1103:refnum<queue>)  [unwired: 3 in, 2 out]
            n496 = while {
              shift-right: [w1112] -> w1107
              shift-left: w1108 -> [w1120]
              shift-right: [w1113] -> w1106
              shift-left: w1109 -> [w1121]
              shift-right: [w1114] -> w1102
              shift-left: w1103 -> [w1116]
              tunnel: w1101 -> [w1110]
              stop <- w1111 stop-if-true
              n497 = Dequeue Element(queue=w1120, error in (no error)=w1121) -> (queue out=w1118:refnum<queue>, element=w1115:T6, error out=w1117:errorcluster)  [unwired: 1 in, 1 out]
              n498 = Unbundle By Name(w1115) -> ("QueueAction"=w1119:T7)
              n499 = case shown="\"Stop_Measurement\"" w1119 {
                tunnel: w1118 -> [w1122 w1146 w1172]
                tunnel: w1117 -> [w1125 w1156 w1171]
                tunnel: w1116 -> [w1127 w1165 w1174]
                tunnel: w1115 -> [w1123 w1133 _]
                tunnel: [w1126 w1165 w1170] -> w1114
                tunnel: [w1124 w1147 w1168] -> w1113
                tunnel: [w1122 w1146 w1169] -> w1112
                tunnel: [_ _ TRUE] -> w1111
                tunnel: w1110 -> [_ w1138 _]
                frame Default {
                  n500 = Enqueue Element(queue=w1127, element=w1123, error in (no error)=w1125) -> (queue out=w1126:refnum<queue>, error out=w1124:errorcluster)  [unwired: 1 in, 1 out]
                }
                frame "Spectrometer_Measure" {
                  w1162 = "_"
                  n501 = Unbundle By Name(w1133) -> ("Time Stamp"=w1132:timestamp)
                  n502 = property on="Nr After Spin" class="DigNum (strict)"() -> ("Value"=w1131:u16)  [unwired: 2 in, 2 out]
                  n503 = Unbundle By Name(w1138) -> ("Wavlength"=w1135:dbl[unit][])
                  n504 = property on="Measure_FileName" class="Str"() -> ("Value"=w1161:string)  [unwired: 2 in, 2 out]
                  n505 = Number To Decimal String(number=w1131) -> (decimal integer string=w1129:string)  [unwired: 1 in]
                  n506 = Format Date/Time String(time format string (%c)="%Y%m%d_%H%M%S", seconds (now)=w1132) -> (date/time string=w1163:string)  [unwired: 1 in]
                  n507 = Concatenate Strings(w1163, w1162, w1161, w1162, "a" ("string"), w1129, ".spectra" ("string")) -> (w1160:string)
                  n508 = property on="Measure_SavePath" class="Path"() -> ("Value"=w1159:path)  [unwired: 2 in, 2 out]
                  n509 = Build Path(base path=w1159, name or relative path=w1160) -> (appended path=w1158:path)
                  n510 = Unbundle By Name(w1133) -> ("Data_Raw"=w1153:T11)
                  n511 = Open/Create/Replace File(file path (use dialog)=w1158, error in=w1156, operation (0:open)=T13."open or create") -> (refnum out=w1155:refnum<file>, error out=w1154:errorcluster)  [unwired: 3 in, 1 out]
                  n512 = Index Array(array=w1153, index=0) -> (element=w1151:T14)
                  n513 = Unbundle By Name(w1151) -> ("Image"=w1139:dbl[][][])
                  n514 = Index Array(array=w1139, index (dim 1)=0 ("disabled index (row)")) -> (element=w1145:dbl[][])  [unwired: 2 in]
                  n515 = Transpose 2D Array(2D array=w1145) -> (transposed array=w1142:dbl[][])
                  n516 = To Unsigned Word Integer(number=w1139) -> (unsigned 16bit integer=w1150:u16[][][])
                  n517 = Matrix Size(0:w1142) -> (2:w1143:i32)  [unwired: 1 out]
                  n518 = Write to Binary File(file (use dialog)=w1155, data=w1150, error in=w1154) -> (refnum out=w1148:refnum<file>, error out=w1149:errorcluster)  [unwired: 3 in, 1 out]
                  n519 = Reciprocal(x=w1143) -> (1/x=w1144:dbl)
                  n520 = Close File(refnum=w1148, error in=w1149) -> (error out=w1147:errorcluster)  [unwired: 1 out]
                  n521 = Initialize Array(w1144, w1143) -> (w1141:dbl[])
                  n522 = call-poly <vilib>:"A x B.vi"("Vector"=w1141, "A"=w1142) -> ("A x Vector"=w1134:dbl[])  [unwired: 1 out]
                  n523 = Bundle("Wavlength"=w1135, "A x Vector"=w1134) -> (w1137:T15)  [unwired: 1 in]
                  n524 = Build Array(w1137) -> (w1136:T16)
                  n525 = property on="Measure_Graph" class="XYGraph (strict)"("Value"=w1136) -> ()  [unwired: 2 in, 2 out]
                }
                frame "Stop_Measurement" {
                  n526 = property on="Automatically \nadjust count" class="Bool (strict)"() -> ("Value"=w1166:bool)  [unwired: 2 in, 2 out]
                  n527 = case shown="True" w1166 {
                    frame False {
                    }
                    frame True {
                      n528 = property on="Nr After Spin" class="DigNum (strict)"() -> ("Value"=w1178:u16)  [unwired: 2 in, 2 out]
                      n529 = Increment(x=w1178) -> (x+1=w1177:u16)
                      n530 = property on="Nr After Spin" class="DigNum (strict)"("Value"=w1177) -> ()  [unwired: 2 in, 2 out]
                    }
                  }
                  n531 = Get Queue Status(queue=w1174) -> (queue out=w1175:refnum<queue>, # elements in queue=w1173:i32)  [unwired: 2 in, 6 out]
                  n532 = property on="Measure_MeasureSpectrum" class="Bool (strict)"("Value"=FALSE ("Measure Spectrum")) -> ()  [unwired: 2 in, 2 out]
                  n533 = for {
                    N: w1173 -> [_]
                    shift-right: [w1184] -> w1170
                    shift-left: w1175 -> [w1185]
                    shift-right: [w1181] -> w1169
                    shift-left: w1172 -> [w1182]
                    shift-right: [w1179] -> w1168
                    shift-left: w1171 -> [w1180]
                    n534 = Dequeue Element(queue=w1185) -> (queue out=w1184:refnum<queue>, element=w1183:T6)  [unwired: 2 in, 2 out]
                    n535 = Enqueue Element(queue=w1182, element=w1183, error in (no error)=w1180) -> (queue out=w1181:refnum<queue>, error out=w1179:errorcluster)  [unwired: 1 in, 1 out]
                  }
                }
              }
            }
            n536 = Release Queue(queue=w1102) -> ()  [unwired: 2 in, 3 out]
          }
          frame "Measure_SpectralStability" {
            w1201 = T6 {"QueueAction"=enum."TimeOut", "Data"=[], "Data_Raw"=[], "Data_Dark"=[], "Data_Ref"=[], "Device Information"=[], "Numeric Control"=0.0, "Boolean"=FALSE, "Wavelength"=[], "Time"=[], "Time Stamp"=timestamp(0 s since 1904-01-01), "Numeric Control 2"=0.0, "TabControl"=enum."Measure"}  # DataQueue
            n537 = Unbundle By Name(w1190) -> ("Time Stamp"=w1196:timestamp)
            n538 = Unbundle By Name(w1190) -> ("Numeric Control"=w1186:dbl)
            n539 = property on="SpectralStability\n_SavePath" class="Path"() -> ("Value"=w1192:path)  [unwired: 2 in, 2 out]
            n540 = property on="SpectralStability\n_FileName" class="Str"() -> ("Value"=w1191:string)  [unwired: 2 in, 2 out]
            n541 = Obtain Queue(name (unnamed)="Temp", element data type=w1201) -> (queue out=w1200:refnum<queue>)  [unwired: 3 in, 2 out]
            n542 = call "Num2Str_TrailingZero.vi"("Numeric Control"=w1186) -> ("format string"=w1189:string)  [unwired: 10 in]
            n543 = Format Date/Time String(time format string (%c)="%Y%m%d_%H%M%S", seconds (now)=w1196) -> (date/time string=w1193:string)  [unwired: 1 in]
            n544 = while {
              shift-right: [w1206] -> w1194
              shift-left: w1203 -> [w1206]
              shift-right: [w1212] -> _
              shift-left: w1200 -> [w1214]
              border: 0 -> [_]
              shift-right: [w1213] -> w1187
              shift-left: w1198 -> [w1222]
              shift-right: [w1211] -> w1188
              shift-left: w1197 -> [w1221]
              tunnel: w1193 -> [w1209]
              tunnel: w1192 -> [w1208]
              tunnel: w1191 -> [w1207]
              tunnel: w1189 -> [w1205]
              tunnel: w1186 -> [w1204]
              stop <- w1210 stop-if-true
              n545 = Dequeue Element(queue=w1222, error in (no error)=w1221) -> (queue out=w1220:refnum<queue>, element=w1218:T6, error out=w1219:errorcluster)  [unwired: 1 in, 1 out]
              n546 = Unbundle By Name(w1218) -> ("QueueAction"=w1217:T7)
              n547 = feedback #2() -> (w1215:i32)
              n548 = case shown="\"Spectrometer_Measure\"" w1217 {
                tunnel: w1220 -> [w1226 w1235 w1241 w1259 w1342 w1349]
                tunnel: w1219 -> [w1225 w1232 w1242 w1260 _ w1350]
                tunnel: w1218 -> [w1227 w1231 _ _ w1296 w1381]
                tunnel: [w1229 w1237 w1248 w1266 w1280 w1382] -> w1216
                tunnel: w1215 -> [w1229 w1237 w1248 w1266 w1340 w1382]
                tunnel: w1214 -> [w1228 w1236 w1244 w1262 w1341 w1359]
                tunnel: [w1226 w1234 w1239 w1257 w1342 w1349] -> w1213
                tunnel: [w1224 w1236 w1243 w1261 w1341 w1359] -> w1212
                tunnel: [w1223 w1233 w1240 w1258 w1285 w1350] -> w1211
                tunnel: [_ TRUE TRUE TRUE _ _] -> w1210
                tunnel: w1209 -> [_ _ _ _ w1338 w1379]
                tunnel: w1208 -> [_ _ _ _ w1305 w1347]
                tunnel: w1207 -> [_ _ _ _ w1337 w1377]
                tunnel: w1206 -> [_ _ _ _ w1312 w1376]
                tunnel: w1205 -> [_ _ _ _ w1339 _]
                tunnel: w1204 -> [_ _ _ _ w1281 _]
                frame Default {
                  n549 = Enqueue Element(queue=w1228, element=w1227, error in (no error)=w1225) -> (queue out=w1224:refnum<queue>, error out=w1223:errorcluster)  [unwired: 1 in, 1 out]
                }
                frame "Close_Program" {
                  n550 = Enqueue Element At Opposite End(queue=w1235, element=w1231, error in (no error)=w1232) -> (queue out=w1234:refnum<queue>, error out=w1233:errorcluster)  [unwired: 1 in, 1 out]
                }
                frame "Abort" {
                  n551 = Get Queue Status(queue=w1244) -> (queue out=w1246:refnum<queue>, # elements in queue=w1247:i32)  [unwired: 2 in, 6 out]
                  n552 = for {
                    N: w1247 -> [_]
                    shift-right: [w1254] -> w1243
                    shift-left: w1246 -> [w1255]
                    shift-right: [w1251] -> w1239
                    shift-left: w1241 -> [w1252]
                    shift-right: [w1249] -> w1240
                    shift-left: w1242 -> [w1250]
                    n553 = Dequeue Element(queue=w1255) -> (queue out=w1254:refnum<queue>, element=w1253:T6)  [unwired: 2 in, 2 out]
                    n554 = Enqueue Element(queue=w1252, element=w1253, error in (no error)=w1250) -> (queue out=w1251:refnum<queue>, error out=w1249:errorcluster)  [unwired: 1 in, 1 out]
                  }
                  n555 = property on="SpectralStability_Record" class="Bool (strict)"("Value"=FALSE ("SpectralStability_Record")) -> ()  [unwired: 2 in, 2 out]
                }
                frame "Stop_Measurement" {
                  n556 = Get Queue Status(queue=w1262) -> (queue out=w1264:refnum<queue>, # elements in queue=w1265:i32)  [unwired: 2 in, 6 out]
                  n557 = for {
                    N: w1265 -> [_]
                    shift-right: [w1272] -> w1261
                    shift-left: w1264 -> [w1273]
                    shift-right: [w1269] -> w1257
                    shift-left: w1259 -> [w1270]
                    shift-right: [w1267] -> w1258
                    shift-left: w1260 -> [w1268]
                    n558 = Dequeue Element(queue=w1273) -> (queue out=w1272:refnum<queue>, element=w1271:T6)  [unwired: 2 in, 2 out]
                    n559 = Enqueue Element(queue=w1270, element=w1271, error in (no error)=w1268) -> (queue out=w1269:refnum<queue>, error out=w1267:errorcluster)  [unwired: 1 in, 1 out]
                  }
                  n560 = property on="SpectralStability_Record" class="Bool (strict)"("Value"=FALSE ("SpectralStability_Record")) -> ()  [unwired: 2 in, 2 out]
                }
                frame "Spectrometer_Measure" {
                  w1336 = "_"
                  n561 = Increment(x=w1340) -> (x+1=w1280:i32)
                  n562 = Unbundle By Name(w1296) -> ("Numeric Control 2"=w1295:dbl)
                  n563 = Unbundle By Name(w1296) -> ("Data_Raw"=w1334:T11)
                  n564 = Format Into String(format string=w1339, w1340) -> (resulting string=w1294:string)  [unwired: 2 in, 1 out]
                  n565 = Concatenate Strings(w1338, w1336, w1337, w1336) -> (w1307:string)
                  n566 = Unbundle By Name(w1312) -> ("Wavlength"=w1310:dbl[unit][])
                  n567 = Index Array(array=w1334, index=0) -> (element=w1332:T14)
                  n568 = Divide(x=w1280, y=w1281) -> (x/y=w1284:dbl)
                  n569 = Concatenate Strings(w1307, "s" ("string"), w1294, ".smean" ("string")) -> (w1316:string)
                  n570 = Concatenate Strings(w1307, "raw" ("string"), w1294, ".spectra" ("string")) -> (w1324:string)
                  n571 = Unbundle By Name(w1332) -> ("Image"=w1320:dbl[][][])
                  n572 = Concatenate Strings(w1307, "timing.txt" ("string")) -> (w1304:string)
                  n573 = Subtract(x=w1281, y=w1280) -> (x-y=w1276:dbl)
                  "SS_StepsLeft" <- w1276
                  n574 = Number To Exponential String(number=w1295, 1:FALSE ("use system decimal point (T)")) -> (E-format string=w1292:string)  [unwired: 2 in]
                  n575 = Build Path(base path=w1305, name or relative path=w1316) -> (appended path=w1313:path)
                  n576 = Build Path(base path=w1305, name or relative path=w1304) -> (appended path=w1303:path)
                  n577 = Multiply(x=w1284, y=100.0) -> (x*y=w1283:dbl)
                  n578 = property on="SS:PeriodicTime" class="DigNum (strict)"() -> ("Value"=w1278:dbl[unit])  [unwired: 2 in, 2 out]
                  n579 = Build Path(base path=w1305, name or relative path=w1324) -> (appended path=w1321:path)
                  n580 = Index Array(array=w1320, index (dim 1)=0 ("disabled index (row)")) -> (element=w1331:dbl[][])  [unwired: 2 in]
                  n581 = To Unsigned Byte Integer(number=w1283) -> (unsigned 8bit integer=→"Horizontal Progress Bar":u8)
                  n582 = To Unsigned Word Integer(number=w1320) -> (unsigned 16bit integer=w1319:u16[][][])
                  n583 = Open/Create/Replace File(file path (use dialog)=w1303, operation (0:open)=T13."open or create") -> (refnum out=w1301:refnum<file>, error out=w1298:errorcluster)  [unwired: 4 in, 1 out]
                  n584 = Concatenate Strings(w1294, "\t", w1292, "\r\n") -> (w1291:string)
                  n585 = Transpose 2D Array(2D array=w1331) -> (transposed array=w1328:dbl[][])
                  n586 = Write to Binary File(file (use dialog)=w1321, data=w1319) -> (refnum out=w1317:refnum<file>, error out=w1318:errorcluster)  [unwired: 4 in, 1 out]
                  n587 = Multiply(x=w1278, y=w1276) -> (x*y=→"SS_TimePrediction":dbl[unit])
                  n588 = Set File Position(refnum=w1301, from (0:start)=enum16{"start", "end", "current"}."end", error in=w1298) -> (refnum out=w1299:refnum<file>, error out=w1297:errorcluster)  [unwired: 1 in]
                  n589 = Matrix Size(0:w1328) -> (2:w1329:i32)  [unwired: 1 out]
                  n590 = Close File(refnum=w1317, error in=w1318) -> (error out=w1288:errorcluster)  [unwired: 1 out]
                  n591 = Reciprocal(x=w1329) -> (1/x=w1330:dbl)
                  n592 = Write to Text File(file (use dialog)=w1299, text=w1291, error in=w1297) -> (refnum out=w1290:refnum<file>, error out=w1289:errorcluster)  [unwired: 1 in, 1 out]
                  n593 = Initialize Array(w1330, w1329) -> (w1327:dbl[])
                  n594 = call-poly <vilib>:"A x B.vi"("Vector"=w1327, "A"=w1328) -> ("A x Vector"=w1309:dbl[])  [unwired: 1 out]
                  n595 = Bundle("Wavlength"=w1310, "A x Vector"=w1309) -> (w1311:T15)  [unwired: 1 in]
                  n596 = Close File(refnum=w1290, error in=w1289) -> (error out=w1286:errorcluster)  [unwired: 1 out]
                  n597 = Write to Binary File(file (use dialog)=w1313, data=w1309) -> (refnum out=w1315:refnum<file>, error out=w1314:errorcluster)  [unwired: 4 in, 1 out]
                  n598 = Build Array(w1311) -> (w1308:T16)
                  n599 = Close File(refnum=w1315, error in=w1314) -> (error out=w1287:errorcluster)  [unwired: 1 out]
                  n600 = property on="SpectralStability:\nGraph" class="XYGraph (strict)"("Value"=w1308) -> ()  [unwired: 2 in, 2 out]
                  n601 = Merge Errors(w1288, w1287, w1286) -> (w1285:errorcluster)
                }
                frame "Transfer_Settings" {
                  w1352 = "\r\n"
                  w1366 = 0.0
                  w1372 = 0 ("index")
                  n602 = Unbundle By Name(w1376) -> ("Dark"=w1373:T11, "Ref"=w1374:T11, "Wavlength"=w1375:dbl[unit][])
                  n603 = Concatenate Strings(w1379, "_", w1377) -> (w1365:string)
                  n604 = property on="SpectralStability_\nPeriodicTime" class="DigNum (strict)"() -> ("Value"=w1358:dbl[unit])  [unwired: 2 in, 2 out]
                  n605 = Unbundle By Name(w1381) -> ("Device Information"=w1380:string[])
                  n606 = property on="SpectralStability_Duration" class="DigNum (strict)"() -> ("Value"=w1357:dbl[unit])  [unwired: 2 in, 2 out]
                  n607 = Index Array(array=w1373, index=w1372) -> (element=w1370:T14)
                  n608 = Index Array(array=w1374, index=w1372) -> (element=w1371:T14)
                  n609 = Concatenate Strings(w1365, "_add.spin" ("string")) -> (w1362:string)
                  n610 = Concatenate Strings(w1365, "_comments.txt" ("string")) -> (w1348:string)
                  n611 = Unbundle By Name(w1370) -> ("Image"=w1344:dbl[][][])
                  n612 = Unbundle By Name(w1371) -> ("Image"=w1343:dbl[][][])
                  n613 = property on="SpectralStability_\nMeasurementNumber" class="DigNum (strict)"() -> ("Value"=w1356:u32)  [unwired: 2 in, 2 out]
                  n614 = Build Path(base path=w1347, name or relative path=w1362) -> (appended path=w1361:path)
                  n615 = Build Path(base path=w1347, name or relative path=w1348) -> (appended path=w1346:path)
                  n616 = node(w1375) -> (w1367:dbl[])
                  n617 = property on="Duration/Times" class="Bool (strict)"() -> ("Value"=w1355:bool)  [unwired: 2 in, 2 out]
                  n618 = To Unsigned Word Integer(number=w1344) -> (unsigned 16bit integer=w1369:u16[][][])
                  n619 = To Unsigned Word Integer(number=w1343) -> (unsigned 16bit integer=w1368:u16[][][])
                  n620 = call "DeviceInfo2Str.vi"("Device Information"=w1380) -> ("String"=w1354:string)  [unwired: 10 in]
                  n621 = property on="SpectralStability:\nComments" class="Str"() -> ("Value"=w1351:string)  [unwired: 2 in, 2 out]
                  n622 = Bundle(w1369, w1368, w1367, w1366, w1366) -> (w1360:cluster{u16[][][], u16[][][], dbl[], dbl, dbl})  [unwired: 1 in]
                  n623 = call "String_SpectralStabilitySettings.vi"("Duration/Times"=w1355, "Measurement Number"=w1356, "Duration"=w1357, "Periodic Time"=w1358) -> ("String"=w1353:string)  [unwired: 7 in]
                  n624 = Concatenate Strings(w1354, w1352, w1353, w1352, w1351) -> (w1345:string)
                  n625 = Write to Binary File(file (use dialog)=w1361, data=w1360) -> ()  [unwired: 4 in, 3 out]
                  n626 = Write to Text File(file (use dialog)=w1346, text=w1345) -> ()  [unwired: 2 in, 3 out]
                }
              }
              n627 = feedback-in #2(w1216) -> ()
            }
          }
          frame "Save_InSitu" {
            w1386 = "\r\n"
            n628 = Unbundle By Name(w1424) -> ("Time Stamp"=w1422:timestamp, "Device Information"=w1413:string[], "Numeric Control"=w1410:dbl, "Numeric Control 2"=w1409:dbl)
            n629 = Unbundle By Name(w1411) -> ("Dark"=w1430:T11, "Ref"=w1428:T11, "Wavlength"=w1432:dbl[unit][])
            n630 = node(w1432) -> (w1425:dbl[])
            n631 = property on="Frames" class="DigNum (strict)"() -> ("Value"=w1397:i32)  [unwired: 2 in, 2 out]
            n632 = call "DeviceInfo2Str.vi"("Device Information"=w1413) -> ("String"=w1412:string)  [unwired: 10 in]
            n633 = Number To Decimal String(number=w1397) -> (decimal integer string=w1396:string)  [unwired: 1 in]
            n634 = property on="Seconds after Spin" class="DigNum (strict)"() -> ("Value"=w1393:dbl[unit])  [unwired: 2 in, 2 out]
            n635 = property on="Seconds to Spin" class="DigNum (strict)"() -> ("Value"=w1394:dbl[unit])  [unwired: 2 in, 2 out]
            n636 = Index Array(array=w1428, index=0) -> (element=w1426:T14)
            n637 = Index Array(array=w1430, index=0) -> (element=w1427:T14)
            n638 = property on="Measure_FileName" class="Str"() -> ("Value"=w1406:string)  [unwired: 2 in, 2 out]
            n639 = property on="Program Spin Coater" class="Arr (strict)"() -> ("Value"=w1395:T2)  [unwired: 2 in, 2 out]
            n640 = Unbundle By Name(w1427) -> ("Image"=w1383:dbl[][][])
            n641 = Unbundle By Name(w1426) -> ("Image"=w1384:dbl[][][])
            n642 = Format Date/Time String(time format string (%c)="%Y%m%d_%H%M%S", seconds (now)=w1422) -> (date/time string=w1421:string)  [unwired: 1 in]
            n643 = call "MeasurementSpin2String.vi"("Seconds after Spin Stop"=w1393, "Seconds to Spin Start"=w1394, "Program Spin Coater"=w1395) -> ("concatenated string"=w1392:string)
            n644 = property on="Duration after" class="DigNum (strict)"() -> ("Value"=w1389:dbl[unit])  [unwired: 2 in, 2 out]
            n645 = Concatenate Strings(w1421, "_" ("string"), w1406) -> (w1419:string)
            n646 = property on="periodic time" class="DigNum (strict)"() -> ("Value"=w1390:dbl[unit])  [unwired: 2 in, 2 out]
            n647 = To Unsigned Word Integer(number=w1383) -> (unsigned 16bit integer=w1400:u16[][][])
            n648 = property on="Spin at end" class="Bool (strict)"() -> ("Value"=w1388:bool)  [unwired: 2 in, 2 out]
            n649 = To Unsigned Word Integer(number=w1384) -> (unsigned 16bit integer=w1399:u16[][][])
            n650 = call "AfterSpinOptions.vi"("Spin at end"=w1388, "Duration after"=w1389, "periodic time"=w1390) -> ("concatenated string"=w1391:string)  [unwired: 8 in]
            n651 = Concatenate Strings(w1412, w1386, "Frames:\t" ("string"), w1396, w1386, w1392, w1386, w1391, w1386, "Comments:" ("string"), w1386, "Measure_Comments") -> (w1408:string)
            n652 = Bundle(w1400, w1399, w1425, "Numeric Control"=w1410, "Numeric Control 2"=w1409) -> (w1403:T17)  [unwired: 1 in]
            n653 = property on="Measure_SavePath" class="Path"() -> ("Value"=w1405:path)  [unwired: 2 in, 2 out]
            n654 = Concatenate Strings(w1419, "_add.spin" ("string")) -> (w1417:string)
            n655 = Concatenate Strings(w1419, "_comments.txt" ("string")) -> (w1416:string)
            n656 = Build Path(base path=w1405, name or relative path=w1417) -> (appended path=w1404:path)
            n657 = Build Path(base path=w1405, name or relative path=w1416) -> (appended path=w1415:path)
            n658 = Write to Text File(file (use dialog)=w1415, text=w1408) -> (error out=w1402:errorcluster)  [unwired: 2 in, 2 out]
            n659 = Write to Binary File(file (use dialog)=w1404, data=w1403) -> (error out=w1401:errorcluster)  [unwired: 4 in, 2 out]
            n660 = flat-sequence {
              tunnel: w1402 -> [_]
              tunnel: w1401 -> [_]
              frame #0 {
                n661 = property on="Action" class="Str"("Value"="" ("Action")) -> ()  [unwired: 2 in, 2 out]
              }
            }
            n662 = property on="Action" class="Str"("Value"="Saving" ("Action")) -> ()  [unwired: 2 in, 2 out]
          }
          frame "Set_Dark" {
            # "Averaging"
            n663 = Unbundle By Name(w1447) -> ("Wavlength"=w1446:dbl[unit][])
            n664 = Unbundle By Name(w1454) -> ("Data_Dark"=w1444:T11)
            n665 = Index Array(array=w1444, index=0) -> (element=w1449:T14)
            n666 = Unbundle By Name(w1449) -> ("Image"=w1443:dbl[][][])
            n667 = Index Array(array=w1443, index (dim 1)=0 ("disabled index (row)")) -> (element=w1441:dbl[][])  [unwired: 2 in]
            n668 = Transpose 2D Array(2D array=w1441) -> (transposed array=w1438:dbl[][])
            n669 = Matrix Size(0:w1438) -> (2:w1439:i32)  [unwired: 1 out]
            n670 = Reciprocal(x=w1439) -> (1/x=w1440:dbl)
            n671 = Initialize Array(w1440, w1439) -> (w1437:dbl[])
            n672 = call-poly <vilib>:"A x B.vi"("Vector"=w1437, "A"=w1438) -> ("A x Vector"=w1436:dbl[])  [unwired: 1 out]
            n673 = Bundle("Wavlength"=w1446, "A x Vector"=w1436) -> (w1448:T15)  [unwired: 1 in]
            n674 = Build Array(w1448) -> (w1445:T16)
            n675 = property on="Measure_Graph" class="XYGraph (strict)"("Value"=w1445) -> ()  [unwired: 2 in, 2 out]
            n676 = Bundle By Name(cluster=w1447, "Dark"=w1444) -> (w1451:T4)
          }
          frame "Set_Ref" {
            # "Averaging"
            n677 = Unbundle By Name(w1456) -> ("Wavlength"=w1455:dbl[unit][])
            n678 = Unbundle By Name(w1473) -> ("Data_Ref"=w1460:T11)
            n679 = Index Array(array=w1460, index=0) -> (element=w1468:T14)
            n680 = Unbundle By Name(w1468) -> ("Image"=w1467:dbl[][][])
            n681 = Index Array(array=w1467, index (dim 1)=0 ("disabled index (row)")) -> (element=w1465:dbl[][])  [unwired: 2 in]
            n682 = Transpose 2D Array(2D array=w1465) -> (transposed array=w1462:dbl[][])
            n683 = Matrix Size(0:w1462) -> (2:w1463:i32)  [unwired: 1 out]
            n684 = Reciprocal(x=w1463) -> (1/x=w1464:dbl)
            n685 = Initialize Array(w1464, w1463) -> (w1461:dbl[])
            n686 = call-poly <vilib>:"A x B.vi"("Vector"=w1461, "A"=w1462) -> ("A x Vector"=w1457:dbl[])  [unwired: 1 out]
            n687 = Bundle("Wavlength"=w1455, "A x Vector"=w1457) -> (w1459:T15)  [unwired: 1 in]
            n688 = Build Array(w1459) -> (w1458:T16)
            n689 = Bundle By Name(cluster=w1456, "Ref"=w1460) -> (w1470:T4)
            n690 = property on="Measure_Graph" class="XYGraph (strict)"("Value"=w1458) -> ()  [unwired: 2 in, 2 out]
          }
          frame "Set_Wavelength" {
            n691 = Unbundle By Name(w1476) -> ("Wavelength"=w1479:dbl[unit][])
            n692 = Bundle By Name(cluster=w1478, "Wavlength"=w1479) -> (w1477:T4)
          }
          frame "Spectrometer_Preview" {
            w1486 = 0 ("index (page)")
            n693 = Unbundle By Name(w1482) -> ("Data_Raw"=w1490:T11)
            n694 = Unbundle By Name(w1491) -> ("Wavlength"=w1485:dbl[unit][])
            n695 = Unbundle By Name(w1482) -> ("TabControl"=w1481:T8)
            n696 = Index Array(array=w1490, index=0) -> (element=w1488:T14)
            n697 = Unbundle By Name(w1488) -> ("Image"=w1487:dbl[][][])
            n698 = Index Array(array=w1487, index (dim 0)=w1486, index (dim 1)=w1486) -> (element=w1484:dbl[])  [unwired: 1 in]
            n699 = Bundle("Wavlength"=w1485, "Image"=w1484) -> (w1483:cluster{"Wavlength":dbl[unit][], "Image":dbl[]})  [unwired: 1 in]
            n700 = Build Array(w1483) -> (w1480:T3)
            n701 = case shown="Default" w1481 {
              tunnel: w1480 -> [w1494 w1495 _]
              frame "Measure" {
                "Measure_Graph" <- w1494
              }
              frame "Spectral Stability" {
                "SpectralStability_Graph" <- w1495
              }
              frame Default {
              }
            }
          }
        }
      }
      frame Error {
        w1501 = T12 4 items=["no dialog", "OK message", "continue or stop message", "OK message + warnings", "continue/stop + warnings"] ("type of dialog (OK msg:1)")
        n702 = call <vilib>:"General Error Handler.vi"("type of dialog (OK msg:1)"=w1501, "error in (no error)"=w1498) -> ("error out"=w1500:errorcluster)  [unwired: 9 in, 4 out]
        n703 = call <vilib>:"Clear Errors.vi"("error in (no error)"=w1500) -> ("error out"=w1497:errorcluster)  [unwired: 5 in, 1 out]
      }
    }
  }
  n704 = while {
    shift-right: [w1504] -> _
    shift-left: w12 -> [w1502]
    shift-right: [w1507] -> _
    shift-left: w7 -> [w1508]
    shift-right: [w1505] -> _
    shift-left: w8 -> [w1506]
    stop <- w1503 stop-if-true
    # "Producer"
    n705 = event shown="[17] \"Measure: Record_Darkspec\", \"SpectralStability: Record_Darkspec\": Value Change" {
      selector: _ -> [_ _ _ _ _ _ _ _ _ _ _ _ _ _ _ _ _ _ _ _ _ _ _ _ _ _ _ _ _]
      dyn-events: _ -> [_ _ _ _ _ _ _ _ _ _ _ _ _ _ _ _ _ _ _ _ _ _ _ _ _ _ _ _ _]
      timeout: -1 -> [_ _ _ _ _ _ _ _ _ _ _ _ _ _ _ _ _ _ _ _ _ _ _ _ _ _ _ _ _]
      tunnel: w1508 -> [w1511 w1526 w1534 w1547 w1562 w1577 w1582 w1597 w1601 w1610 w1622 w1637 w1661 w1664 w1671 w1707 w1712 w1740 w1746 w1766 w1775 w1784 w1792 w1798 w1807 w1822 w1839 w1845 w1860]
      tunnel: [w1511 w1523 w1533 w1547 w1562 w1577 w1582 w1597 w1601 w1610 w1622 w1637 w1661 w1664 w1671 w1707 w1712 w1740 w1745 w1766 w1775 w1784 w1792 w1798 w1805 w1820 w1839 w1845 w1860] -> w1507
      tunnel: w1506 -> [w1510 w1525 w1537 w1545 w1559 w1576 w1581 w1594 w1602 w1611 w1623 w1635 w1656 w1663 w1668 w1687 w1711 w1731 w1752 w1765 w1774 w1783 w1791 w1797 w1811 w1826 w1840 w1844 w1858]
      tunnel: [w1510 w1519 w1528 w1541 w1558 w1574 w1581 w1593 w1603 w1612 w1624 w1633 w1655 w1663 w1666 w1689 w1709 w1725 w1744 w1760 w1771 w1780 w1791 w1797 w1811 w1826 w1840 w1844 w1855] -> w1505
      tunnel: w1502 -> [w1512 w1527 w1538 w1546 w1561 w1578 w1583 w1596 w1605 w1614 w1626 w1636 w1658 w1665 w1669 w1688 w1713 w1732 w1754 w1767 w1776 w1785 w1793 w1799 w1812 w1827 w1838 w1846 w1859]
      tunnel: [w1512 w1524 w1536 w1542 w1560 w1575 w1583 w1595 w1604 w1613 w1625 w1634 w1657 w1665 w1670 w1690 w1710 w1726 w1753 w1761 w1772 w1781 w1793 w1796 w1810 w1825 w1838 w1846 w1856] -> w1504
      tunnel: [_ TRUE _ _ _ _ _ _ _ _ _ _ _ _ _ _ _ _ _ _ _ _ _ _ _ _ _ _ _] -> w1503
      event Timeout {
        n706 = event-data() -> ()  [unwired: 1 in, 3 out]
      }
      event "Stop Button": Value Change {
        w1515 = T6 {"QueueAction"=enum."TimeOut", "Data"=[], "Data_Raw"=[], "Data_Dark"=[], "Data_Ref"=[], "Device Information"=[], "Numeric Control"=0.0, "Boolean"=FALSE, "Wavelength"=[], "Time"=[], "Time Stamp"=timestamp(0 s since 1904-01-01), "Numeric Control 2"=0.0, "TabControl"=enum."Measure"}  # DataQueue
        w1518 = T9 {"QueueAction"=enum."TimeOut", "Numeric 1"=0.0, "Numeric 2"=0.0, "Boolean 1"=FALSE, "Boolean 2"=FALSE, "Spin Program"=[], "Spin Prg v07"=[], "Time Stamp"=timestamp(0 s since 1904-01-01), "TabControl"=enum."Measure"}  # Device Queue
        n707 = event-data() -> ()  [unwired: 1 in, 6 out]
        n708 = Bundle By Name(cluster=w1518, "QueueAction"=DeviceQueue_Action."Close_Program") -> (w1516:T9)
        n709 = Enqueue Element At Opposite End(queue=w1527, element=w1516, error in (no error)=w1525) -> (queue out=w1524:refnum<queue>, error out=w1520:errorcluster)  [unwired: 1 in, 1 out]
        n710 = Bundle By Name(cluster=w1515, "QueueAction"=DataQueue_Action."Close_Program") -> (w1513:T6)
        n711 = Enqueue Element At Opposite End(queue=w1526, element=w1513, error in (no error)=w1525) -> (queue out=w1523:refnum<queue>, error out=w1521:errorcluster)  [unwired: 1 in, 1 out]
        n712 = Merge Errors(w1521, w1520) -> (w1519:errorcluster)
      }
      event "Abort Button": Value Change {
        w1532 = T6 {"QueueAction"=enum."TimeOut", "Data"=[], "Data_Raw"=[], "Data_Dark"=[], "Data_Ref"=[], "Device Information"=[], "Numeric Control"=0.0, "Boolean"=FALSE, "Wavelength"=[], "Time"=[], "Time Stamp"=timestamp(0 s since 1904-01-01), "Numeric Control 2"=0.0, "TabControl"=enum."Measure"}  # DataQueue
        w1540 = T9 {"QueueAction"=enum."TimeOut", "Numeric 1"=0.0, "Numeric 2"=0.0, "Boolean 1"=FALSE, "Boolean 2"=FALSE, "Spin Program"=[], "Spin Prg v07"=[], "Time Stamp"=timestamp(0 s since 1904-01-01), "TabControl"=enum."Measure"}  # Device Queue
        n713 = event-data() -> ()  [unwired: 1 in, 6 out]
        n714 = Bundle By Name(cluster=w1540, "QueueAction"=DeviceQueue_Action."Abort") -> (w1539:T9)
        n715 = Bundle By Name(cluster=w1532, "QueueAction"=DataQueue_Action."Abort") -> (w1530:T6)
        n716 = Enqueue Element At Opposite End(queue=w1538, element=w1539, error in (no error)=w1537) -> (queue out=w1536:refnum<queue>, error out=w1529:errorcluster)  [unwired: 1 in, 1 out]
        n717 = Enqueue Element At Opposite End(queue=w1534, element=w1530, error in (no error)=w1529) -> (queue out=w1533:refnum<queue>, error out=w1528:errorcluster)  [unwired: 1 in, 1 out]
      }
      event "Init_Spectrometer": Value Change {
        n718 = event-data() -> ()  [unwired: 1 in, 6 out]
        n719 = case shown="False" "Init_Spectrometer" {
          tunnel: [w1549 w1552] -> w1543
          frame True {
            n720 = property on="Tab Control" class="TabCtl (strict)"() -> ("Value"=w1548:T1)  [unwired: 2 in, 2 out]
            n721 = Bundle By Name(cluster=T9 {"QueueAction"=enum."TimeOut", "Numeric 1"=0.0, "Numeric 2"=0.0, "Boolean 1"=FALSE, "Boolean 2"=FALSE, "Spin Program"=[], "Spin Prg v07"=[], "Time Stamp"=timestamp(0 s since 1904-01-01), "TabControl"=enum."Measure"} ("element"), "QueueAction"=DeviceQueue_Action."Spectrometer_Init", "TabControl"=w1548) -> (w1549:T9)
          }
          frame False {
            n722 = Bundle By Name(cluster=T9 {"QueueAction"=enum."TimeOut", "Numeric 1"=0.0, "Numeric 2"=0.0, "Boolean 1"=FALSE, "Boolean 2"=FALSE, "Spin Program"=[], "Spin Prg v07"=[], "Time Stamp"=timestamp(0 s since 1904-01-01), "TabControl"=enum."Measure"} ("element"), "QueueAction"=DeviceQueue_Action."Spectrometer_Close") -> (w1552:T9)
          }
        }
        n723 = Enqueue Element(queue=w1546, element=w1543, error in (no error)=w1545) -> (queue out=w1542:refnum<queue>, error out=w1541:errorcluster)  [unwired: 1 in, 1 out]
      }
      event "Init_Arduino": Value Change {
        # "Shutter is closed after init"
        n724 = event-data() -> ("NewVal"=w1557:bool)  [unwired: 1 in, 5 out]
        n725 = case shown="True" w1557 {
          tunnel: [w1563 w1566] -> w1556
          frame False {
            w1565 = T9 {"QueueAction"=enum."TimeOut", "Numeric 1"=0.0, "Numeric 2"=0.0, "Boolean 1"=FALSE, "Boolean 2"=FALSE, "Spin Program"=[], "Spin Prg v07"=[], "Time Stamp"=timestamp(0 s since 1904-01-01), "TabControl"=enum."Measure"}  # Device Queue
            n726 = Bundle By Name(cluster=w1565, "QueueAction"=DeviceQueue_Action."Arduino_Close") -> (w1563:T9)
          }
          frame True {
            w1568 = T9 {"QueueAction"=enum."TimeOut", "Numeric 1"=0.0, "Numeric 2"=0.0, "Boolean 1"=FALSE, "Boolean 2"=FALSE, "Spin Program"=[], "Spin Prg v07"=[], "Time Stamp"=timestamp(0 s since 1904-01-01), "TabControl"=enum."Measure"}  # Device Queue
            n727 = Bundle By Name(cluster=w1568, "QueueAction"=DeviceQueue_Action."Arduino_Init") -> (w1566:T9)
          }
        }
        n728 = property on="Shutter Toggle" class="Bool (strict)"("Value"=FALSE ("Shutter Toggle")) -> ()  [unwired: 2 in, 2 out]
        n729 = Enqueue Element(queue=w1561, element=w1556, error in (no error)=w1559) -> (queue out=w1560:refnum<queue>, error out=w1558:errorcluster)  [unwired: 1 in, 1 out]
      }
      event "Program Spin Coater": Value Change {
        w1580 = T9 {"QueueAction"=enum."TimeOut", "Numeric 1"=0.0, "Numeric 2"=0.0, "Boolean 1"=FALSE, "Boolean 2"=FALSE, "Spin Program"=[], "Spin Prg v07"=[], "Time Stamp"=timestamp(0 s since 1904-01-01), "TabControl"=enum."Measure"}  # Device Queue
        n730 = event-data() -> ("NewVal"=w1569:T2)  [unwired: 1 in, 5 out]
        n731 = property on="Seconds to Spin" class="DigNum (strict)"() -> ("Value"=w1571:dbl[unit])  [unwired: 2 in, 2 out]
        n732 = node(w1571) -> (w1570:dbl)
        n733 = Bundle By Name(cluster=w1580, "QueueAction"=DeviceQueue_Action."Arduino_LoadProgram", "Spin Prg v07"=w1569, "Numeric 1"=w1570) -> (w1579:T9)
        n734 = Enqueue Element(queue=w1578, element=w1579, error in (no error)=w1576) -> (queue out=w1575:refnum<queue>, error out=w1574:errorcluster)  [unwired: 1 in, 1 out]
        n735 = property on="Measure_IntegrationTime" class="DigNum (strict)"() -> ("Value"=w1572:dbl[unit])  [unwired: 2 in, 2 out]
        n736 = property on="Measure_IntegrationTime" class="DigNum (strict)"("Val(Sgnl)"=w1572) -> ()  [unwired: 2 in, 2 out]
      }
      event "SHUTTER DEBUG": Value Change {
        n737 = event-data() -> ("NewVal"=w1585:bool)  [unwired: 1 in, 5 out]
        n738 = Select(t=u8 0, s=w1585, f=u8 2) -> (s? t:f=w1584:u8)
        n739 = property on="Shutter Position" class="DigNum (strict)"("DisabledEnum"=w1584) -> ()  [unwired: 2 in, 2 out]
        n740 = property on="Shutter Close" class="Bool (strict)"("DisabledEnum"=w1584) -> ()  [unwired: 2 in, 2 out]
        n741 = property on="Shutter Open" class="Bool (strict)"("DisabledEnum"=w1584) -> ()  [unwired: 2 in, 2 out]
      }
      event "Shutter Position": Value Change {
        w1592 = FALSE ("Shutter Close")
        w1590 = T9 {"QueueAction"=enum."TimeOut", "Numeric 1"=0.0, "Numeric 2"=0.0, "Boolean 1"=FALSE, "Boolean 2"=FALSE, "Spin Program"=[], "Spin Prg v07"=[], "Time Stamp"=timestamp(0 s since 1904-01-01), "TabControl"=enum."Measure"}  # Device Queue
        (unwired) DeviceQueue_Action."Arduino_SetSpeed" ("QueueAction")
        (unwired) T9 {"QueueAction"=enum."TimeOut", "Numeric 1"=0.0, "Numeric 2"=0.0, "Boolean 1"=FALSE, "Boolean 2"=FALSE, "Spin Program"=[], "Spin Prg v07"=[], "Time Stamp"=timestamp(0 s since 1904-01-01), "TabControl"=enum."Measure"}  # Device Queue
        n742 = event-data() -> ("NewVal"=w1588:u16)  [unwired: 1 in, 5 out]
        n743 = property on="Shutter Close" class="Bool (strict)"("Value"=w1592) -> ()  [unwired: 2 in, 2 out]
        n744 = property on="Shutter Open" class="Bool (strict)"("Value"=w1592) -> ()  [unwired: 2 in, 2 out]
        n745 = Bundle By Name(cluster=w1590, "QueueAction"=DeviceQueue_Action."Arduino_Shutter_SetPosition", "Numeric 1"=w1588) -> (w1591:T9)
        n746 = Enqueue Element(queue=w1596, element=w1591, error in (no error)=w1594) -> (queue out=w1595:refnum<queue>, error out=w1593:errorcluster)  [unwired: 1 in, 1 out]
      }
      event "Shutter Close": Value Change {
        w1600 = T9 {"QueueAction"=enum."TimeOut", "Numeric 1"=0.0, "Numeric 2"=0.0, "Boolean 1"=FALSE, "Boolean 2"=FALSE, "Spin Program"=[], "Spin Prg v07"=[], "Time Stamp"=timestamp(0 s since 1904-01-01), "TabControl"=enum."Measure"}  # Device Queue
        (unwired) DeviceQueue_Action."Arduino_SetSpeed" ("QueueAction")
        (unwired) T9 {"QueueAction"=enum."TimeOut", "Numeric 1"=0.0, "Numeric 2"=0.0, "Boolean 1"=FALSE, "Boolean 2"=FALSE, "Spin Program"=[], "Spin Prg v07"=[], "Time Stamp"=timestamp(0 s since 1904-01-01), "TabControl"=enum."Measure"}  # Device Queue
        n747 = event-data() -> ()  [unwired: 1 in, 6 out]
        n748 = property on="Shutter Open" class="Bool (strict)"("Value"=FALSE ("Shutter Open")) -> ()  [unwired: 2 in, 2 out]
        n749 = Bundle By Name(cluster=w1600, "QueueAction"=DeviceQueue_Action."Arduino_Shutter_Close") -> (w1599:T9)
        n750 = Enqueue Element(queue=w1605, element=w1599, error in (no error)=w1602) -> (queue out=w1604:refnum<queue>, error out=w1603:errorcluster)  [unwired: 1 in, 1 out]
      }
      event "Shutter Open": Value Change {
        w1609 = T9 {"QueueAction"=enum."TimeOut", "Numeric 1"=0.0, "Numeric 2"=0.0, "Boolean 1"=FALSE, "Boolean 2"=FALSE, "Spin Program"=[], "Spin Prg v07"=[], "Time Stamp"=timestamp(0 s since 1904-01-01), "TabControl"=enum."Measure"}  # Device Queue
        (unwired) DeviceQueue_Action."Arduino_SetSpeed" ("QueueAction")
        (unwired) T9 {"QueueAction"=enum."TimeOut", "Numeric 1"=0.0, "Numeric 2"=0.0, "Boolean 1"=FALSE, "Boolean 2"=FALSE, "Spin Program"=[], "Spin Prg v07"=[], "Time Stamp"=timestamp(0 s since 1904-01-01), "TabControl"=enum."Measure"}  # Device Queue
        n751 = event-data() -> ()  [unwired: 1 in, 6 out]
        n752 = property on="Shutter Close" class="Bool (strict)"("Value"=FALSE ("Shutter Open")) -> ()  [unwired: 2 in, 2 out]
        n753 = Bundle By Name(cluster=w1609, "QueueAction"=DeviceQueue_Action."Arduino_Shutter_Open") -> (w1608:T9)
        n754 = Enqueue Element(queue=w1614, element=w1608, error in (no error)=w1611) -> (queue out=w1613:refnum<queue>, error out=w1612:errorcluster)  [unwired: 1 in, 1 out]
      }
      event "Shutter Toggle": Value Change {
        w1621 = T9 {"QueueAction"=enum."TimeOut", "Numeric 1"=0.0, "Numeric 2"=0.0, "Boolean 1"=FALSE, "Boolean 2"=FALSE, "Spin Program"=[], "Spin Prg v07"=[], "Time Stamp"=timestamp(0 s since 1904-01-01), "TabControl"=enum."Measure"}  # Device Queue
        (unwired) T9 {"QueueAction"=enum."TimeOut", "Numeric 1"=0.0, "Numeric 2"=0.0, "Boolean 1"=FALSE, "Boolean 2"=FALSE, "Spin Program"=[], "Spin Prg v07"=[], "Time Stamp"=timestamp(0 s since 1904-01-01), "TabControl"=enum."Measure"}  # Device Queue
        n755 = event-data() -> ("NewVal"=w1619:bool)  [unwired: 1 in, 5 out]
        n756 = Select(t=DeviceQueue_Action."Arduino_Shutter_Open" ("QueueAction"), s=w1619, f=DeviceQueue_Action."Arduino_Shutter_Close" ("QueueAction")) -> (s? t:f=w1616:T10)
        n757 = Bundle By Name(cluster=w1621, "QueueAction"=w1616) -> (w1620:T9)
        n758 = Enqueue Element(queue=w1626, element=w1620, error in (no error)=w1623) -> (queue out=w1625:refnum<queue>, error out=w1624:errorcluster)  [unwired: 1 in, 1 out]
      }
      event "Measure_IntegrationTime", "SpectralStability_IntegrationTime": Value Change {
        w1639 = T9 {"QueueAction"=enum."TimeOut", "Numeric 1"=0.0, "Numeric 2"=0.0, "Boolean 1"=FALSE, "Boolean 2"=FALSE, "Spin Program"=[], "Spin Prg v07"=[], "Time Stamp"=timestamp(0 s since 1904-01-01), "TabControl"=enum."Measure"}  # Device Queue
        n759 = event-data() -> ("NewVal"=w1631:dbl[unit])  [unwired: 1 in, 5 out]
        n760 = property on="Calculate Frames" class="Bool (strict)"() -> ("Value"=w1627:bool)  [unwired: 2 in, 2 out]
        n761 = node(w1631) -> (w1630:dbl)
        n762 = property on="Tab Control" class="TabCtl (strict)"() -> ("Value"=w1629:T1)  [unwired: 2 in, 2 out]
        n763 = property on="Tab Control" class="TabCtl (strict)"() -> ("Value"=w1628:T1)  [unwired: 2 in, 2 out]
        n764 = case shown="\"Measure\"" w1629 {
          tunnel: w1639 -> [w1640 w1646 w1652]
          tunnel: [w1640 w1643 w1649] -> w1638
          tunnel: DeviceQueue_Action."Spectrometer_SetIntegrationTime" ("QueueAction") -> [_ w1645 w1651]
          tunnel: w1630 -> [_ w1644 w1650]
          tunnel: w1628 -> [_ w1642 w1647]
          tunnel: w1627 -> [_ w1641 _]
          frame Default {
          }
          frame "Measure" {
            n765 = Bundle By Name(cluster=w1646, "QueueAction"=w1645, "Numeric 1"=w1644, "Boolean 1"=w1641, "TabControl"=w1642) -> (w1643:T9)
          }
          frame "Spectral Stability" {
            n766 = Bundle By Name(cluster=w1652, "QueueAction"=w1651, "Numeric 1"=w1650, "Boolean 1"=FALSE, "TabControl"=w1647) -> (w1649:T9)
          }
        }
        n767 = Enqueue Element(queue=w1636, element=w1638, error in (no error)=w1635) -> (queue out=w1634:refnum<queue>, error out=w1633:errorcluster)  [unwired: 1 in, 1 out]
      }
      event "Frames": Value Change {
        w1660 = T9 {"QueueAction"=enum."TimeOut", "Numeric 1"=0.0, "Numeric 2"=0.0, "Boolean 1"=FALSE, "Boolean 2"=FALSE, "Spin Program"=[], "Spin Prg v07"=[], "Time Stamp"=timestamp(0 s since 1904-01-01), "TabControl"=enum."Measure"}  # Device Queue
        n768 = event-data() -> ()  [unwired: 1 in, 6 out]
        n769 = Bundle By Name(cluster=w1660, "QueueAction"=DeviceQueue_Action."Spectrometer_SetFrames", "Numeric 1"="Frames") -> (w1659:T9)
        n770 = Enqueue Element(queue=w1658, element=w1659, error in (no error)=w1656) -> (queue out=w1657:refnum<queue>, error out=w1655:errorcluster)  [unwired: 1 in, 1 out]
      }
      event "Seconds to Spin", "Seconds after Spin": Value Change {
        n771 = event-data() -> ()  [unwired: 1 in, 6 out]
        n772 = property on="Program Spin Coater" class="Arr (strict)"() -> ("Value"=w1662:T2)  [unwired: 2 in, 2 out]
        n773 = property on="Program Spin Coater" class="Arr (strict)"("Val(Sgnl)"=w1662) -> ()  [unwired: 2 in, 2 out]
      }
      event "Calculate Frames": Value Change {
        n774 = event-data() -> ("NewVal"=w1672:bool)  [unwired: 1 in, 5 out]
        n775 = case shown="False" w1672 {
          tunnel: [0 2] -> w1667
          tunnel: w1669 -> [w1674 w1683]
          tunnel: [w1674 w1681] -> w1670
          tunnel: w1668 -> [w1673 w1680]
          tunnel: [w1673 w1676] -> w1666
          frame False {
          }
          frame True {
            w1682 = T9 {"QueueAction"=enum."TimeOut", "Numeric 1"=0.0, "Numeric 2"=0.0, "Boolean 1"=FALSE, "Boolean 2"=FALSE, "Spin Program"=[], "Spin Prg v07"=[], "Time Stamp"=timestamp(0 s since 1904-01-01), "TabControl"=enum."Measure"}  # Device Queue
            n776 = property on="Measure_IntegrationTime" class="DigNum (strict)"() -> ("Value"=w1678:dbl[unit])  [unwired: 2 in, 2 out]
            n777 = node(w1678) -> (w1677:dbl)
            n778 = Bundle By Name(cluster=w1682, "QueueAction"=DeviceQueue_Action."Spectrometer_SetIntegrationTime", "Numeric 1"=w1677) -> (w1684:T9)
            n779 = Enqueue Element(queue=w1683, element=w1684, error in (no error)=w1680) -> (queue out=w1681:refnum<queue>, error out=w1676:errorcluster)  [unwired: 1 in, 1 out]
          }
        }
        n780 = property on="Frames" class="DigNum (strict)"("DisabledEnum"=w1667) -> ()  [unwired: 2 in, 2 out]
      }
      event "Record RefSpec": Value Change {
        w1703 = T9 {"QueueAction"=enum."TimeOut", "Numeric 1"=0.0, "Numeric 2"=0.0, "Boolean 1"=FALSE, "Boolean 2"=FALSE, "Spin Program"=[], "Spin Prg v07"=[], "Time Stamp"=timestamp(0 s since 1904-01-01), "TabControl"=enum."Measure"}  # Device Queue
        n781 = event-data() -> ()  [unwired: 1 in, 6 out]
        n782 = property on="Shutter Toggle" class="Bool (strict)"("Value"=FALSE ("Shutter Toggle")) -> ()  [unwired: 2 in, 2 out]
        n783 = Bundle By Name(cluster=w1703, "QueueAction"=DeviceQueue_Action."Arduino_Shutter_Open") -> (w1700:T9)
        n784 = Bundle By Name(cluster=w1700, "QueueAction"=DeviceQueue_Action."Wait", "Numeric 1"=0.5) -> (w1699:T9)
        n785 = Bundle By Name(cluster=w1699, "QueueAction"=DeviceQueue_Action."Spectrometer_SetReference") -> (w1698:T9)
        n786 = Bundle By Name(cluster=w1698, "QueueAction"=DeviceQueue_Action."Arduino_Shutter_Close") -> (w1691:T9)
        n787 = Enqueue Element(queue=w1688, element=w1700, error in (no error)=w1687) -> (queue out=w1697:refnum<queue>, error out=w1694:errorcluster)  [unwired: 1 in, 1 out]
        n788 = Enqueue Element(queue=w1697, element=w1699, error in (no error)=w1694) -> (queue out=w1696:refnum<queue>, error out=w1693:errorcluster)  [unwired: 1 in, 1 out]
        n789 = Enqueue Element(queue=w1696, element=w1698, error in (no error)=w1693) -> (queue out=w1695:refnum<queue>, error out=w1692:errorcluster)  [unwired: 1 in, 1 out]
        n790 = Enqueue Element(queue=w1695, element=w1691, error in (no error)=w1692) -> (queue out=w1690:refnum<queue>, error out=w1689:errorcluster)  [unwired: 1 in, 1 out]
      }
      event "Measure_Preview", "SpectralStability_Preview": Value Change {
        n791 = event-data() -> ("NewVal"=w1708:bool)  [unwired: 1 in, 5 out]
        n792 = case shown="False" w1708 {
          tunnel: w1713 -> [w1715 w1720]
          tunnel: w1711 -> [w1714 w1719]
          tunnel: [w1715 w1718] -> w1710
          tunnel: [w1714 w1717] -> w1709
          frame False {
          }
          frame True {
            w1723 = T9 {"QueueAction"=enum."TimeOut", "Numeric 1"=0.0, "Numeric 2"=0.0, "Boolean 1"=FALSE, "Boolean 2"=FALSE, "Spin Program"=[], "Spin Prg v07"=[], "Time Stamp"=timestamp(0 s since 1904-01-01), "TabControl"=enum."Measure"}  # Device Queue
            n793 = property on="Tab Control" class="TabCtl (strict)"() -> ("Value"=w1716:T1)  [unwired: 2 in, 2 out]
            n794 = Bundle By Name(cluster=w1723, "QueueAction"=DeviceQueue_Action."Spectrometer_Preview", "TabControl"=w1716) -> (w1722:T9)
            n795 = Enqueue Element(queue=w1720, element=w1722, error in (no error)=w1719) -> (queue out=w1718:refnum<queue>, error out=w1717:errorcluster)  [unwired: 1 in, 1 out]
          }
        }
      }
      event "Measure:\nRecord_Darkspec", "SpectralStability:\nRecord_Darkspec": Value Change {
        w1738 = T9 {"QueueAction"=enum."TimeOut", "Numeric 1"=0.0, "Numeric 2"=0.0, "Boolean 1"=FALSE, "Boolean 2"=FALSE, "Spin Program"=[], "Spin Prg v07"=[], "Time Stamp"=timestamp(0 s since 1904-01-01), "TabControl"=enum."Measure"}  # Device Queue
        n796 = event-data() -> ()  [unwired: 1 in, 6 out]
        n797 = property on="Shutter Toggle" class="Bool (strict)"("Value"=FALSE ("Shutter Toggle")) -> ()  [unwired: 2 in, 2 out]
        n798 = Bundle By Name(cluster=w1738, "QueueAction"=DeviceQueue_Action."Arduino_Shutter_Close") -> (w1737:T9)
        n799 = Bundle By Name(cluster=w1737, "QueueAction"=DeviceQueue_Action."Wait", "Numeric 1"=0.5) -> (w1736:T9)
        n800 = Bundle By Name(cluster=w1736, "QueueAction"=DeviceQueue_Action."Spectrometer_SetDarkspec") -> (w1741:T9)
        n801 = Enqueue Element(queue=w1732, element=w1737, error in (no error)=w1731) -> (queue out=w1730:refnum<queue>, error out=w1729:errorcluster)  [unwired: 1 in, 1 out]
        n802 = Enqueue Element(queue=w1730, element=w1736, error in (no error)=w1729) -> (queue out=w1727:refnum<queue>, error out=w1728:errorcluster)  [unwired: 1 in, 1 out]
        n803 = Enqueue Element(queue=w1727, element=w1741, error in (no error)=w1728) -> (queue out=w1726:refnum<queue>, error out=w1725:errorcluster)  [unwired: 1 in, 1 out]
      }
      event "StartMeasurement_Button": Value Change {
        w1748 = T6 {"QueueAction"=enum."TimeOut", "Data"=[], "Data_Raw"=[], "Data_Dark"=[], "Data_Ref"=[], "Device Information"=[], "Numeric Control"=0.0, "Boolean"=FALSE, "Wavelength"=[], "Time"=[], "Time Stamp"=timestamp(0 s since 1904-01-01), "Numeric Control 2"=0.0, "TabControl"=enum."Measure"}  # DataQueue
        w1756 = T9 {"QueueAction"=enum."TimeOut", "Numeric 1"=0.0, "Numeric 2"=0.0, "Boolean 1"=FALSE, "Boolean 2"=FALSE, "Spin Program"=[], "Spin Prg v07"=[], "Time Stamp"=timestamp(0 s since 1904-01-01), "TabControl"=enum."Measure"}  # Device Queue
        n804 = event-data() -> ()  [unwired: 1 in, 6 out]
        n805 = property on="Measure_Preview" class="Bool (strict)"("Value"=FALSE ("Preview")) -> ()  [unwired: 2 in, 2 out]
        n806 = Get Date/Time In Seconds() -> (seconds since 1Jan1904=w1742:timestamp)
        n807 = Bundle By Name(cluster=w1756, "QueueAction"=DeviceQueue_Action."Measure_InSituAdvanced", "Time Stamp"=w1742) -> (w1755:T9)
        n808 = Enqueue Element(queue=w1754, element=w1755, error in (no error)=w1752) -> (queue out=w1753:refnum<queue>, error out=w1743:errorcluster)  [unwired: 1 in, 1 out]
        n809 = Bundle By Name(cluster=w1748, "QueueAction"=DataQueue_Action."Measure_InSituSpinCoating", "Time Stamp"=w1742) -> (w1749:T6)
        n810 = Enqueue Element(queue=w1746, element=w1749, error in (no error)=w1743) -> (queue out=w1745:refnum<queue>, error out=w1744:errorcluster)  [unwired: 1 in, 1 out]
      }
      event "StartSpin_Button": Value Change {
        w1768 = T9 {"QueueAction"=enum."TimeOut", "Numeric 1"=0.0, "Numeric 2"=0.0, "Boolean 1"=FALSE, "Boolean 2"=FALSE, "Spin Program"=[], "Spin Prg v07"=[], "Time Stamp"=timestamp(0 s since 1904-01-01), "TabControl"=enum."Measure"}  # Device Queue
        n811 = event-data() -> ()  [unwired: 1 in, 6 out]
        n812 = Bundle By Name(cluster=w1768, "QueueAction"=DeviceQueue_Action."Arduino_StartProgram") -> (w1759:T9)
        n813 = Bundle By Name(cluster=w1759, "QueueAction"=DeviceQueue_Action."Arduino_Shutter_Close") -> (w1757:T9)
        n814 = Enqueue Element(queue=w1767, element=w1759, error in (no error)=w1765) -> (queue out=w1762:refnum<queue>, error out=w1763:errorcluster)  [unwired: 1 in, 1 out]
        n815 = Enqueue Element(queue=w1762, element=w1757, error in (no error)=w1763) -> (queue out=w1761:refnum<queue>, error out=w1760:errorcluster)  [unwired: 1 in, 1 out]
      }
      event "ESC_Milliseconds": Value Change {
        w1777 = T9 {"QueueAction"=enum."TimeOut", "Numeric 1"=0.0, "Numeric 2"=0.0, "Boolean 1"=FALSE, "Boolean 2"=FALSE, "Spin Program"=[], "Spin Prg v07"=[], "Time Stamp"=timestamp(0 s since 1904-01-01), "TabControl"=enum."Measure"}  # Device Queue
        n816 = event-data() -> ()  [unwired: 1 in, 6 out]
        n817 = Bundle By Name(cluster=w1777, "QueueAction"=DeviceQueue_Action."Arduino_SetMillis", "Numeric 1"="ESC_Milliseconds") -> (w1773:T9)
        n818 = Enqueue Element(queue=w1776, element=w1773, error in (no error)=w1774) -> (queue out=w1772:refnum<queue>, error out=w1771:errorcluster)  [unwired: 1 in, 1 out]
      }
      event "ESC_Speed": Value Change {
        w1786 = T9 {"QueueAction"=enum."TimeOut", "Numeric 1"=0.0, "Numeric 2"=0.0, "Boolean 1"=FALSE, "Boolean 2"=FALSE, "Spin Program"=[], "Spin Prg v07"=[], "Time Stamp"=timestamp(0 s since 1904-01-01), "TabControl"=enum."Measure"}  # Device Queue
        n819 = event-data() -> ()  [unwired: 1 in, 6 out]
        n820 = Bundle By Name(cluster=w1786, "QueueAction"=DeviceQueue_Action."Arduino_SetSpeed", "Numeric 1"="ESC_Speed") -> (w1782:T9)
        n821 = Enqueue Element(queue=w1785, element=w1782, error in (no error)=w1783) -> (queue out=w1781:refnum<queue>, error out=w1780:errorcluster)  [unwired: 1 in, 1 out]
      }
      event "ESC DEBUG": Value Change {
        n822 = event-data() -> ()  [unwired: 1 in, 6 out]
        n823 = Select(t=u8 0, s="ESC DEBUG", f=u8 2) -> (s? t:f=w1787:u8)
        n824 = property on="ESC_Milliseconds" class="DigNum (strict)"("DisabledEnum"=w1787) -> ()  [unwired: 2 in, 2 out]
        n825 = property on="ESC_Speed" class="DigNum (strict)"("DisabledEnum"=w1787) -> ()  [unwired: 2 in, 2 out]
      }
      event "Measure_FramesSpectrometer", "SpectralStability_FramesSpectrometer": Value Change {
        w1801 = T9 {"QueueAction"=enum."TimeOut", "Numeric 1"=0.0, "Numeric 2"=0.0, "Boolean 1"=FALSE, "Boolean 2"=FALSE, "Spin Program"=[], "Spin Prg v07"=[], "Time Stamp"=timestamp(0 s since 1904-01-01), "TabControl"=enum."Measure"}  # Device Queue
        n826 = event-data() -> ("NewVal"=w1795:dbl)  [unwired: 1 in, 5 out]
        n827 = property on="Tab Control" class="TabCtl (strict)"() -> ("Value"=w1794:T1)  [unwired: 2 in, 2 out]
        n828 = Bundle By Name(cluster=w1801, "QueueAction"=DeviceQueue_Action."Spectrometer_SetFrames", "Numeric 1"=w1795, "TabControl"=w1794) -> (w1802:T9)
        n829 = Enqueue Element(queue=w1799, element=w1802) -> (queue out=w1796:refnum<queue>)  [unwired: 2 in, 2 out]
      }
      event "Measure_MeasureSpectrum", "SpectralStability_MeasureSpectrum": Value Change {
        w1809 = T6 {"QueueAction"=enum."TimeOut", "Data"=[], "Data_Raw"=[], "Data_Dark"=[], "Data_Ref"=[], "Device Information"=[], "Numeric Control"=0.0, "Boolean"=FALSE, "Wavelength"=[], "Time"=[], "Time Stamp"=timestamp(0 s since 1904-01-01), "Numeric Control 2"=0.0, "TabControl"=enum."Measure"}  # DataQueue
        w1814 = T9 {"QueueAction"=enum."TimeOut", "Numeric 1"=0.0, "Numeric 2"=0.0, "Boolean 1"=FALSE, "Boolean 2"=FALSE, "Spin Program"=[], "Spin Prg v07"=[], "Time Stamp"=timestamp(0 s since 1904-01-01), "TabControl"=enum."Measure"}  # Device Queue
        n830 = event-data() -> ()  [unwired: 1 in, 6 out]
        n831 = property on="Tab Control" class="TabCtl (strict)"() -> ("Value"=w1803:T1)  [unwired: 2 in, 2 out]
        n832 = Get Date/Time In Seconds() -> (seconds since 1Jan1904=w1804:timestamp)
        n833 = Bundle By Name(cluster=w1814, "QueueAction"=DeviceQueue_Action."Measure_Spectrum", "Time Stamp"=w1804, "TabControl"=w1803) -> (w1815:T9)
        n834 = Enqueue Element(queue=w1812, element=w1815) -> (queue out=w1810:refnum<queue>)  [unwired: 2 in, 2 out]
        n835 = Bundle By Name(cluster=w1809, "QueueAction"=DataQueue_Action."Measure_Spectrum", "TabControl"=w1803) -> (w1806:T6)
        n836 = Enqueue Element(queue=w1807, element=w1806) -> (queue out=w1805:refnum<queue>)  [unwired: 2 in, 2 out]
      }
      event "SpectralStability_Record": Value Change {
        w1824 = T6 {"QueueAction"=enum."TimeOut", "Data"=[], "Data_Raw"=[], "Data_Dark"=[], "Data_Ref"=[], "Device Information"=[], "Numeric Control"=0.0, "Boolean"=FALSE, "Wavelength"=[], "Time"=[], "Time Stamp"=timestamp(0 s since 1904-01-01), "Numeric Control 2"=0.0, "TabControl"=enum."Measure"}  # DataQueue
        w1829 = T9 {"QueueAction"=enum."TimeOut", "Numeric 1"=0.0, "Numeric 2"=0.0, "Boolean 1"=FALSE, "Boolean 2"=FALSE, "Spin Program"=[], "Spin Prg v07"=[], "Time Stamp"=timestamp(0 s since 1904-01-01), "TabControl"=enum."Measure"}  # Device Queue
        n837 = event-data() -> ()  [unwired: 1 in, 6 out]
        n838 = property on="Duration/\nTimes" class="Bool (strict)"() -> ("Value"=w1817:bool)  [unwired: 2 in, 2 out]
        n839 = case shown="False" w1817 {
          tunnel: ["SpectralStability_\nMeasurementNumber" w1832] -> w1816
          frame False {
            # "Number"
          }
          frame True {
            # "Duration"
            n840 = property on="SpectralStability_\nPeriodicTime" class="DigNum (strict)"() -> ("Value"=w1834:dbl[unit])  [unwired: 2 in, 2 out]
            n841 = Divide(x="SpectralStability_Duration", y=w1834) -> (x/y=w1835:dbl)
            n842 = Round Toward +Infinity(x=w1835) -> (ceil(x): smallest int >= x=w1833:dbl)
            n843 = Increment(x=w1833) -> (x+1=w1832:dbl)
          }
        }
        n844 = Get Date/Time In Seconds() -> (seconds since 1Jan1904=w1818:timestamp)
        n845 = property on="Tab Control" class="TabCtl (strict)"() -> ("Value"=w1819:T1)  [unwired: 2 in, 2 out]
        n846 = Bundle By Name(cluster=w1829, "QueueAction"=DeviceQueue_Action."Measure_SpectralStability", "Time Stamp"=w1818, "TabControl"=w1819, "Numeric 1"=w1816) -> (w1830:T9)
        n847 = property on="SS_StepsLeft" class="DigNum (strict)"("Value"=w1816) -> ()  [unwired: 2 in, 2 out]
        n848 = Enqueue Element(queue=w1827, element=w1830) -> (queue out=w1825:refnum<queue>)  [unwired: 2 in, 2 out]
        n849 = Bundle By Name(cluster=w1824, "QueueAction"=DataQueue_Action."Measure_SpectralStability", "TabControl"=w1819, "Time Stamp"=w1818, "Numeric Control"=w1816) -> (w1821:T6)
        n850 = Enqueue Element(queue=w1822, element=w1821) -> (queue out=w1820:refnum<queue>)  [unwired: 2 in, 2 out]
      }
      event "Automatically \nadjust count": Value Change {
        n851 = event-data() -> ("NewVal"=w1843:bool)  [unwired: 1 in, 5 out]
        n852 = Select(t=u8 2, s=w1843, f=u8 0) -> (s? t:f=w1837:u8)
        n853 = property on="Spectra Count" class="DigNum (strict)"("DisabledEnum"=w1837) -> ()  [unwired: 2 in, 2 out]
      }
      event "Duration/Times": Value Change {
        n854 = event-data() -> ("NewVal"=w1849:bool)  [unwired: 1 in, 5 out]
        n855 = case shown="False" w1849 {
          tunnel: [FALSE TRUE] -> w1848
          tunnel: [TRUE FALSE] -> w1847
          frame False {
          }
          frame True {
          }
        }
        n856 = property on="SpectralStability_Duration" class="DigNum (strict)"("Visible"=w1848) -> ()  [unwired: 2 in, 2 out]
        n857 = property on="SpectralStability_\nMeasurementNumber" class="DigNum (strict)"("Visible"=w1847) -> ()  [unwired: 2 in, 2 out]
      }
      event "Tab Control": Value Change {
        w1854 = FALSE ("SpectralStability_Preview")
        n858 = event-data() -> ("NewVal"=w1857:T1)  [unwired: 1 in]
        n859 = case shown="\"Spectral Stability\"" w1857 {
          tunnel: w1859 -> [w1862 w1875 w1890]
          tunnel: [w1862 w1864 w1881] -> w1856
          tunnel: w1858 -> [w1861 w1874 w1889]
          tunnel: w1857 -> [_ w1873 w1888]
          tunnel: [w1861 w1863 w1880] -> w1855
          frame Default {
          }
          frame "Measure" {
            w1877 = T9 {"QueueAction"=enum."TimeOut", "Numeric 1"=0.0, "Numeric 2"=0.0, "Boolean 1"=FALSE, "Boolean 2"=FALSE, "Spin Program"=[], "Spin Prg v07"=[], "Time Stamp"=timestamp(0 s since 1904-01-01), "TabControl"=enum."Measure"}  # Device Queue
            n860 = property on="Measure_IntegrationTime" class="DigNum (strict)"() -> ("Value"=w1872:dbl[unit])  [unwired: 2 in, 2 out]
            n861 = node(w1872) -> (w1871:dbl)
            n862 = Bundle By Name(cluster=w1877, "QueueAction"=DeviceQueue_Action."Spectrometer_SetIntegrationTime", "Numeric 1"=w1871, "TabControl"=w1873) -> (w1868:T9)
            n863 = property on="Measure_FramesSpectrometer" class="DigNum (strict)"() -> ("Value"=w1866:dbl)  [unwired: 2 in, 2 out]
            n864 = Enqueue Element(queue=w1875, element=w1868, error in (no error)=w1874) -> (queue out=w1870:refnum<queue>, error out=w1869:errorcluster)  [unwired: 1 in, 1 out]
            n865 = Bundle By Name(cluster=w1868, "QueueAction"=DeviceQueue_Action."Spectrometer_SetFrames", "Numeric 1"=w1866) -> (w1865:T9)
            n866 = Enqueue Element(queue=w1870, element=w1865, error in (no error)=w1869) -> (queue out=w1864:refnum<queue>, error out=w1863:errorcluster)  [unwired: 1 in, 1 out]
          }
          frame "Spectral Stability" {
            w1892 = T9 {"QueueAction"=enum."TimeOut", "Numeric 1"=0.0, "Numeric 2"=0.0, "Boolean 1"=FALSE, "Boolean 2"=FALSE, "Spin Program"=[], "Spin Prg v07"=[], "Time Stamp"=timestamp(0 s since 1904-01-01), "TabControl"=enum."Measure"}  # Device Queue
            n867 = property on="SpectralStability_IntegrationTime" class="DigNum (strict)"() -> ("Value"=w1879:dbl[unit])  [unwired: 2 in, 2 out]
            n868 = node(w1879) -> (w1887:dbl)
            n869 = property on="SpectralStability_FramesSpectrometer" class="DigNum (strict)"() -> ("Value"=w1878:dbl)  [unwired: 2 in, 2 out]
            n870 = Bundle By Name(cluster=w1892, "QueueAction"=DeviceQueue_Action."Spectrometer_SetIntegrationTime", "Numeric 1"=w1887, "TabControl"=w1888) -> (w1884:T9)
            n871 = Enqueue Element(queue=w1890, element=w1884, error in (no error)=w1889) -> (queue out=w1886:refnum<queue>, error out=w1885:errorcluster)  [unwired: 1 in, 1 out]
            n872 = Bundle By Name(cluster=w1884, "QueueAction"=DeviceQueue_Action."Spectrometer_SetFrames", "Numeric 1"=w1878) -> (w1882:T9)
            n873 = Enqueue Element(queue=w1886, element=w1882, error in (no error)=w1885) -> (queue out=w1881:refnum<queue>, error out=w1880:errorcluster)  [unwired: 1 in, 1 out]
          }
        }
        n874 = property on="SpectralStability_Preview" class="Bool (strict)"("Value"=w1854) -> ()  [unwired: 2 in, 2 out]
        n875 = property on="Measure_Preview" class="Bool (strict)"("Value"=w1854) -> ()  [unwired: 2 in, 2 out]
      }
    }
  }
  n876 = disable-structure shown="Disabled" {
    frame Disabled {
      w1894 = T9 {"QueueAction"=enum."TimeOut", "Numeric 1"=0.0, "Numeric 2"=0.0, "Boolean 1"=FALSE, "Boolean 2"=FALSE, "Spin Program"=[], "Spin Prg v07"=[], "Time Stamp"=timestamp(0 s since 1904-01-01), "TabControl"=enum."Measure"}  # Device Queue
      w1896 = T9 {"QueueAction"=enum."TimeOut", "Numeric 1"=0.0, "Numeric 2"=0.0, "Boolean 1"=FALSE, "Boolean 2"=FALSE, "Spin Program"=[], "Spin Prg v07"=[], "Time Stamp"=timestamp(0 s since 1904-01-01), "TabControl"=enum."Measure"}  # Device Queue
      n877 = Bundle By Name(cluster=w1894, "QueueAction"=DeviceQueue_Action."Arduino_SetSpeed") -> (w1895:T9)  [unwired: 1 in]
      n878 = Bundle By Name(cluster=w1896) -> ()  [unwired: 2 in, 1 out]
      n879 = Enqueue Element(element=w1895) -> ()  [unwired: 3 in, 3 out]
    }
    frame Enabled {
    }
  }
  n880 = Release Queue(queue=w9) -> ()  [unwired: 2 in, 3 out]
  n881 = Release Queue(queue=w10) -> ()  [unwired: 2 in, 3 out]
